vi "Main.vi"() -> ()   [LabVIEW 2023]
doc: "This Continuous Measurement sample project is based on the Queued Message Handler template.\n\nThe Event Handling Loop generates messages based on user interface actions.\n\nThe Message Handling Loop processes messages generated by the Event Handling Loop, or by other messages. There are also Acquisition and Logging message handling loop subVIs, and a chart updating loop."
uses:
  support/Message Queue/Message Cluster.ctl
  Drivers/Resideo Gas Valve/Type Definitions/Temperature Control.ctl
  controls/Product Type.ctl
  controls/UI Data.ctl
  Modbus/Modbus All Data.ctl
  Modbus/Modbus PLC Data All.ctl
  Modbus/Modbus FVIR Control.ctl
  Modbus/Modbus Timing.ctl
  <vilib>/Utility/miscctls.llb/LVDateTimeRec.ctl
  Modbus/Modbus LDO Control.ctl
  WritingDataFile/Data to Save.ctl
  support/Terminate Conditions Cluster.ctl
  Drivers/Inficon Transmitter/Type Definitions/Inficon Data.ctl
  Modbus/Modbus Gas Meter Data.ctl
  Drivers/Alicat LabVIEW Drivers 2v1/Sub-VIs/Data Cluster.ctl
  Drivers/Alicat LabVIEW Drivers 2v1/Sub-VIs/Units of Measure.ctl
  Gas_Rate/HEWH ANSI Rate.ctl
  Drivers/Resideo Gas Valve/Type Definitions/Vesta Info.ctl
  support/Agilent Data.ctl
  support/Event Booleans.ctl
  support/StartStopIntellifaucet.ctl
  support/Mannequin and Gas Position.ctl
  support/Message Queue/Enqueue Message (Single).vi
  <vilib>/Utility/error.llb/Error Cluster From Error Code.vi
  Tenney/support/Message Queue/Enqueue Message (Single).vi
  <vilib>/ErrorRing/Error Ring.xnode
  support/User Event - Stop/User Event - Stop.lvlib
  support/Message Queue/Message Queue.lvlib
  Modbus/Modbus.lvlib
  WritingDataFile/WritingDataFile.lvlib
  SRI8610C - GasChromatograph/SRI8610C-GasChromatograph.lvlib
  Tenney/support/Message Queue/Tenney Message Queue.lvlib
panel:
  out "elements":T1[](array[typedef])
  out "Input Registers":u16[](array[numeric])
  out "States":string[](array[string])
  in  "error in":errorcluster
  out "Version Info":string
  in  "Tab Control":T2(tab)
  out "Actuator spill can is going to Work Pos - FVIR":bool
  out "Actuator spill can is going to Home Pos - FVIR":bool
  out "Actuator mannequin is going to Work Pos - FVIR":bool
  out "Actuator mannequin is going to Home Pos - FVIR":bool
  out "Burner-FVIR":bool caption="Burner - FVIR"
  in  "Move mannequin - Go to Work Pos":bool
  in  "Move mannequin - Go to Home Pos":bool
  in  "Spill can - Go to Work Pos":bool
  in  "Spill can - Go to Home Pos":bool
  in  "Select test case":i32(listbox)
  in  "Stop Test Case FVIR":bool
  in  "Start Test Case FVIR":bool
  out "Start recording data - FVIR":bool
  out "Test chamber is in sequence - FVIR":bool
  out "Can is spilling - FVIR":bool
  out "Mannequin is moving - FVIR":bool
  out "Higher than 0.9% butane":bool
  in  "Water Outlet Valve Close FVIR":bool
  in  "Water Outlet Valve Open FVIR":bool
  in  "Gas Solenoid Valve Close FVIR":bool
  in  "Gas Solenoid Valve Open FVIR":bool
  in  "Water Inlet Valve Close FVIR":bool
  in  "Water Inlet Valve Open FVIR":bool
  out "Water Outlet Flow Proportional - FVIR":bool
  out "Intellifaucet Start - FVIR":bool
  out "Gas Solenoid Valve - FVIR":bool
  out "Water Inlet Valve - FVIR":bool
  out "Water Outlet Valve - FVIR":bool
  in  "Start - SRI Log":bool
  in  "Stop- SRI Log":bool
  in  "Gas Meter Tare Total FVIR":bool
  in  "Gas Meter Tare Rate FVIR":bool
  in  "Reset Flow Meter FVIR":bool caption="Reset Flow Meter"
  in  "Proportioning Valve - FVIR":dbl caption="Proportioning Valve" max=100.0
  in  "Valve % Open - FVIR":dbl=100.0 caption="Valve % Open" min=15.0 max=100.0
  in  "Temp (°F)-FVIR":dbl=70.0 caption="Temperature (°F)" min=32.0 max=203.0
  in  "Start Intellifaucet DRK375 - FVIR":bool
  in  "Stop Intellifaucet DRK375 - FVIR":bool
  out "FVIR Status":string
  in  "Burner OFF FVIR":bool
  in  "Burner ON FVIR":bool
  in  "Test Type - Rate FVIR":string(combo)="Rate"
  out "FVIR Rate Info":string[][](array[string])
  out "FVIR Data":string[][](array[string])
  out "ANSI Display FVIR":string caption="ANSI Display 1"
  in  "Start ANSI FVIR":bool caption="Start ANSI"
  out "Status for error - FVIR":string caption="Error status for FVIR"
  out "Error - FVIR":bool caption="Error"
  in  "Water Heater Temperature (°F) FVIR":bool
  in  "Water Heater Temp (°F) FVIR 2":T3={"Water Heater Temp (°F)"=120, "Differential  (°F)"=10.0} {"Water Heater Temp (°F)" min=32 max=203}
  in  "EnviraCom (On/Off)":bool
  in  "SET Temperature (°F)-EnviraCom":bool
  in  "Short Draw Flow Rate (GPM)":dbl=0.92 format="%#_13g"
  in  "Reset Flow Meter":bool
  in  "Blower OFF":bool
  in  "Blower ON":bool
  in  "Conveyor OFF":bool
  in  "Conveyor ON":bool
  out "Blower":bool
  out "Conveyor":bool
  out "Rotary Actuator (ON/OFF)":bool
  out "Oil spray 1.33cc/min":bool
  out "Oil spray 1.1cc/min":bool
  out "Oil spray 0.8cc/min":bool
  out "Burner-LDO":bool caption="Burner"
  in  "Gas Meter Tare Total":bool
  in  "Gas Meter Tare Rate":bool
  out "LDO Data":string[][](array[string])
  in  "Proportioning Valve - LDO":dbl caption="Proportioning Valve" max=100.0
  in  "Valve % Open - LDO":dbl=50.0 caption="Valve % Open" min=15.0 max=100.0
  in  "Temp (°F)-LDO":dbl=70.0 caption="Temperature (°F)" min=32.0 max=203.0
  in  "Start Intellifaucet DRK375 - LDO":bool
  in  "Stop Intellifaucet DRK375 - LDO":bool
  out "Start recording data - LDO":bool
  out "Test chamber is in sequence":bool
  out "LDO Auto Stop Condition Met?":bool
  in  "Stop Test Case LDO":bool
  in  "Start Test Case LDO":bool
  in  "Water Outlet Valve Close LDO":bool
  in  "Water Outlet Valve Open LDO":bool
  in  "Water Inlet Valve Close LDO":bool
  in  "Water Inlet Valve Open LDO":bool
  in  "Gas Solenoid Valve Close LDO":bool
  in  "Gas Solenoid Valve Open LDO":bool
  in  "Oil Spray 0.8 cc/min Close":bool
  in  "Oil Spray 0.8 cc/min Open":bool
  in  "Oil Spray 1.1 cc/min Close":bool
  in  "Oil Spray 1.1 cc/min Open":bool
  in  "Oil Spray 1.33 cc/min Close":bool
  in  "Oil Spray 1.33 cc/min Open":bool
  in  "Rotary Actuator OFF":bool
  in  "Rotary Actuator ON":bool
  out "Water Outlet Flow Proportional":bool
  out "Intellifaucet Start_LDO":bool
  out "Gas Solenoid Valve":bool
  out "Water Inlet Valve":bool
  out "Water Outlet Valve":bool
  out "LDO Status":string
  in  "Test Type - Rate":string(combo)="Rate"
  out "LDO Rate Info":string[][](array[string])
  out "ANSI Display LDO":string caption="ANSI Display 1"
  in  "Start ANSI LDO":bool caption="Start ANSI"
  in  "Long Draw Flow Rate (GPM)":dbl=0.92 format="%#_13g"
  in  "LDO-Manual Flow Control?":bool=TRUE
  in  "Reset BINs":bool
  in  "Temperature Parameters":T3={"Water Heater Temp (°F)"=135, "Differential  (°F)"=10.0} {"Water Heater Temp (°F)" min=32 max=203}
  in  "Water Heater Temperature (°F)":bool
  in  "Product Type":T4
  out "XY Graph - LDO":T5(graph)
  out "XY Graph - FVIR":T5(graph)
  in  "Y-Axis2 - FVIR":string(combo)
  in  "Y-Axis1 - FVIR":string(combo)
  in  "X-Axis - FVIR":string(combo)
  in  "Y-Axis2 - LDO":string(combo)
  in  "Y-Axis1 - LDO":string(combo)
  in  "X-Axis - LDO":string(combo)
  in  "HHV-NG-Manual":sgl=1069.0
  in  "Manual Heating Value":bool
  out "Error - LDO":bool caption="Error"
  out "Status for error - LDO":string caption="Error status for LDO"
  in  "EnviraCom LDO COM":refnum<visa-resource-name>="EnviraCom_LDO"
  in  "FVIR Save Rate (Default ms)":i32=500
  in  "stop FVIR test":bool
  in  "Pilot Rate (BTU/hr)-FVIR":dbl=800.0
  out "FVIR - Filepath":path
  out "LDO - Filepath":path
  in  "Vesta ON Temperature FVIR":T3={"Water Heater Temp (°F)"=120, "Differential  (°F)"=10.0} {"Water Heater Temp (°F)" min=32 max=203}
  in  "Vesta OFF Temperature FVIR":T3={"Water Heater Temp (°F)"=55, "Differential  (°F)"=10.0} {"Water Heater Temp (°F)" min=32 max=203}
  in  "Vesta ON Temperature LDO":T3={"Water Heater Temp (°F)"=135, "Differential  (°F)"=10.0} {"Water Heater Temp (°F)" min=32 max=203}
  in  "Vesta OFF Temperature LDO":T3={"Water Heater Temp (°F)"=55, "Differential  (°F)"=10.0} {"Water Heater Temp (°F)" min=32 max=203}
  in  "Agilent 34972A":refnum<visa-resource-name>="34972A"
  in  "stop ldo test":bool
  in  "Debug":bool
  out "Message Loop":string[](array[string])
  in  "Time Pause Between Next Mannequin Sequence":u16=60
  in  "Number of Mannequin Movement":u16=3
  in  "Time Delay of Change direction of Mannequin Actuators (mS)":u16=1000
  in  "Full Mannequin Sequence":bool
  in  "FVIR-Flow Rate (GPM)":dbl=3.0 format="%#_13g"
  in  "Temp (°F) - Automatic Mode (FVIR)":dbl=73.0 min=32.0 max=203.0
  in  "Valve % Open - Automatic Mode (FVIR)":dbl=100.0 min=15.0 max=100.0
  in  "Send parameters to PLC FVIR":bool
  in  "Ultramat 23_FVIR":refnum<visa-resource-name>="ULTRAMAT_FVIR"
  in  "VESTA FVIR COM":refnum<visa-resource-name>="VESTA_FVIR"
  in  "FVIR Alicat VISA":refnum<visa-resource-name>="ALICAT_40SLPM_FVIR"
  in  "Ultramat 23_LDO":refnum<visa-resource-name>="ULTRAMAT_LDO"
  in  "LDO Alicat VISA":refnum<visa-resource-name>="ALICAT_40SLPM_LDO"
  in  "VESTA LDO COM":refnum<visa-resource-name>="VESTA_LDO"
  in  "Reset LDO Timers":bool
  in  "Start Auto GPM Gallons-LDO":dbl=5.0 format="%#_13g"
  in  "Clear Unist Alarm":bool
  in  "Temp (°F) - Automatic Mode (LDO)":dbl=70.0 min=32.0 max=203.0
  in  "Valve % Open - Automatic Mode (LDO)":dbl=50.0 min=15.0 max=100.0
  in  "Precondition Purge Gallons":u16=200 caption="Precondition Purge Time (Sec)"
  in  "Pilot Rate (BTU/hr)-LDO":dbl=800.0
  out "FVIR PLC lifebit":bool
  out "Labview lifebit":bool
  in  "Send parameters to PLC LDO":bool
  in  "Burner cycle 1 to 10 - Duty cycle ON (default 55 min.)":u16=55 caption="Burner cycle 1 to 10 - Duty cycle ON"
  in  "Burner cycle 1 to 10 - Duty cycle OFF (default 5 min.)":u16=5 caption="Burner cycle 1 to 10 - Duty cycle OFF"
  in  "Burner cycle 11 to 12 - Duty cycle ON (default 235 min.)":u16=235 caption="Burner cycle 11 to 12 - Duty cycle ON"
  in  "Burner cycle 11 to 12 - Duty cycle OFF (default 5 min.)":u16=5 caption="Burner cycle 11 to 12 - Duty cycle OFF"
  in  "Burner cycle 13 to end - Duty cycle ON (default 55 min.)":u16=55 caption="Burner cycle 13 to end - Duty cycle ON"
  in  "Burner cycle 13 to end - Duty cycle OFF (default 5 min.)":u16=5 caption="Burner cycle 13 to end - Duty cycle OFF"
  in  "Oil 1st sequence ON (default 5 min.)":u16=5 caption="Oil 1st sequence ON"
  in  "Oil 1st sequence OFF (default 5 min.)":u16=25 caption="Oil 1st sequence OFF"
  in  "All subsequent sequence ON (default 3 min.)":u16=3 caption="All subsequent sequence ON"
  in  "All subsequent sequence OFF (default 27 min.)":u16=27 caption="All subsequent sequence OFF"
  in  "Oil spray preconditioning period ON (default 10 min.)":u16=10 caption="Oil spray preconditioning period ON"
  in  "Oil spray preconditioning period OFF  (default 20 min.)":u16=20 caption="Oil spray preconditioning period OFF"
  in  "PLC IP address":string="10.2.0.11"
  in  "Inficon IP Address":string="192.168.1.32"
  in  "Save Rate (ms)":i32=10000
  in  "PLC Loop Rate Standard":u32=1000
  out "EnviraCom is working":bool
  out "Retry Count":dbl
  out "EnviraCom LDO Loop Count":i32
  out "EnviraCom LDO State":string
  out "Vesta is working":bool
  out "Retry Count":dbl
  out "Vesta LDO Loop Count":i32
  out "Vesta LDO State":string
  out "Modbus Loop Rate":i32
  # "Manual mode"
  # "Automatic mode"
  # "Water Outlet Valve"
  # "Gas Solenoid Valve"
  # "Water Inlet Valve"
  # "Status of valves"
  # "Status of actuators"
  # "Status of chamber"
  # "Intellifaucet Control"
  # "Gas Meter"
  # "Water Flow Meter"
  # "Burner ON/OFF"
  # "Manual mode"
  # "Status of devices"
  # "Status of chamber"
  # "Status of valves"
  # "Intellifaucet Control"
  # "This button resets all saved temperature limits. \nKnob must be on Pilot."
  # "Water Flow Meter"
  # "Blower Control"
  # "Conveyor Control"
  # "Gas Meter"
  # "Automatic mode"
  # "Start and stop LDO test"
  # "Water Outlet Valve"
  # "Water Inlet Valve"
  # "Gas Solenoid Valve"
  # "Oil spray at 0.8 cc/min"
  # "Oil spray at 1.1 cc/min"
  # "Oil spray at 1.33 cc/min"
  # "Rotary Actuator\n(Burner ON/OFF)"
  # "LDO Parameters -"
  # "Changing parameters to PLC"
  # "FVIR Changing parameters to PLC"
  # "EnviraCom Communication"
  # "Vesta Communication"
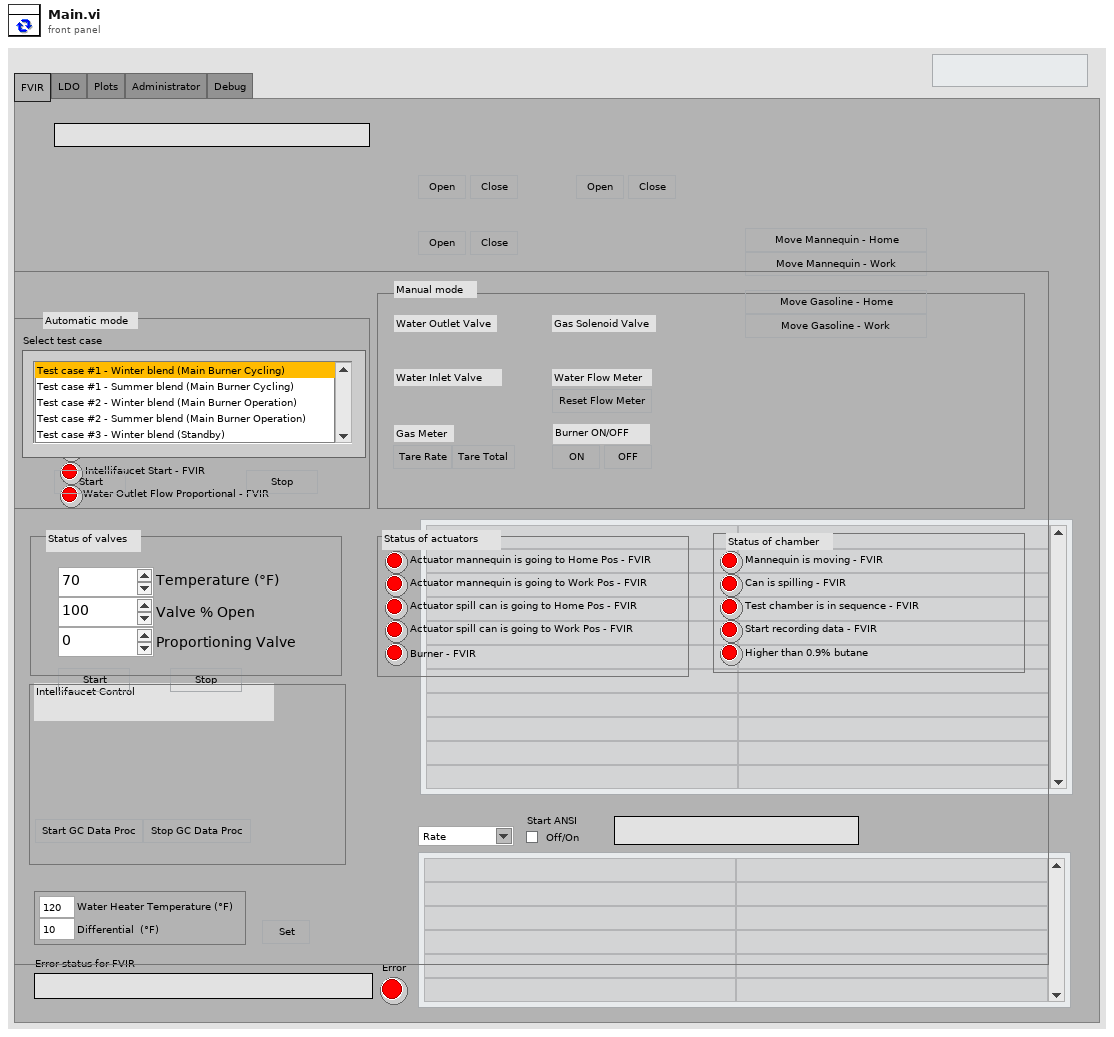
[diagram p1: front panel]
types:
  T1 = typedef "Message Queue.lvlib/Message Cluster.ctl" = cluster{"Message":string, "Message Data":variant}
  T2 = enum32{"FVIR", "LDO", "Plots", "Administrator", "Debug"}
  T3 = typedef "Temperature Control.ctl" = cluster{"Water Heater Temp (°F)":u16, "Differential  (°F)":dbl}
  T4 = typedef "Product Type.ctl" = enum16{"", "Standard ATM", "Power Vent"}
  T5 = cluster{"Time Array Output":dbl[], "Data Array Output":dbl[]}[]
  T6 = typedef "Event Booleans.ctl" = cluster{"Burner ON - LDO":bool, "0.8 ml Bool":bool, "1.1 Bool":bool, "1.33 Bool":bool, "Start recording data-LDO":bool, "Rotary Actuator (ON/OFF)":bool, "Burner ON - FVIR":bool, "Start recording data -FVIR ":bool}
  T7 = typedef "Modbus All Data.ctl" = cluster{"PLC Data":T8, "Inficon Data - ALL":T15, "Gas Data":cluster{"Gas Data - LDO":T16, "Gas Data - FVIR":T16}, "Ultramat 23":cluster{"Ultramat 23 - LDO":string[][], "Ultramat 23 - FVIR":string[][]}, "ANSI Rates":cluster{"ANSI Rate LDO":T19, "ANSI Rate FVIR":T19}, "Vesta Data":cluster{"Vesta LDO":T20, "Vesta FVIR":T20}, "Agilent Data":T21}
  T8 = typedef "Modbus PLC Data All.ctl" = cluster{"PLC Data - FVIR":T9, "PLC Data - LDO":T12, "PLC Registers - ALL":i16[], "Data to Save - ALL":T13, "Terminate Conditions - LDO":T14, "Terminate Conditions - FVIR":cluster{"SRI Butane Values":string[][], "Stop FVIR Test":bool}}
  T9 = typedef "Modbus FVIR Control.ctl" = cluster{"Reset FVIR Totalizer (Status)":bool, "Spare 14":bool, "Actuator mannequin is going to Work Pos - FVIR":bool, "Actuator mannequin is going to Home Pos - FVIR":bool, "Test chamber is in sequence - FVIR ":bool, "Water flow DRK375 is open - FVIR":bool, "Gas Solenoid Valve - FVIR":bool, "Water Inlet Valve - FVIR":bool, "Water Outlet Flow Proportional - FVIR":bool, "Start recording data - FVIR":bool, "Actuator spill can is going to Work Pos - FVIR":bool, "Actuator spill can is going to Home Pos - FVIR":bool, "Water Outlet Valve - FVIR":bool, "Can is spilling - FVIR":bool, "Mannequin is moving - FVIR":bool, "FVIR PLC lifebit":bool, "Status for Error - FVIR":string, "Error-FVIR":bool, "Sensor Data -FVIR":string[][], "Totalized Flow (Gallons)":dbl, "Timing":T10}
  T10 = typedef "Modbus Timing.ctl" = cluster{"First Call Time Ref":dbl, "Precondition Time Ref":dbl, "Test Time Ref":dbl, "Get First Call Time":bool, "Get Precondition Time":bool, "Get Test Time":bool, "Display Time":dbl, "Real-Time Clock":T11, "Absolute Time":dbl}
  T11 = typedef "LVDateTimeRec.ctl" = cluster{"fractional second":dbl, "second":i32, "minute":i32, "hour":i32, "day of month":i32, "month":i32, "year":i32, "day of week":i32, "day of year":i32, "DST":i32}
  T12 = typedef "Modbus LDO Control.ctl" = cluster{"LDO PLC Life Bit":bool, "Start recording data - LDO":bool, "Spare 1":bool, "Water Outlet Valve - LDO":bool, "Water Inlet Valve - LDO":bool, "Gas Solenoid Valve - LDO":bool, "Water flow DRK375 is open - LDO":bool, "Test chamber is in sequence - LDO":bool, "Oil spray 0.8cc/min - LDO":bool, "Oil spray 1.1cc/min - LDO":bool, "Oil spray 1.33cc/min - LDO":bool, "Rotary Actuator (ON/OFF) - LDO":bool, "Water Outlet Flow Proportional - LDO":bool, "Conveyor ON/OFF":bool, "Blower ON/OFF":bool, "Reset LDO Totalizer (Status)":bool, "Status for error - LDO":string, "Error - LDO":bool, "Sensor Data - LDO":string[][], "Thermal Efficiency Rate (GPM)":dbl, "Thermal Efficiency":dbl, "Totalized Flow (Gallons)":dbl, "Counter of oil injections 1.33 cc/min":u16, "Total Cycle Counter":u16, "Counter of oil injections 1.1 cc/min":u16, "Counter of oil injections 0.8 cc/min":u16, "Timing":T10}
  T13 = typedef "Data to Save.ctl" = cluster{"LDO Full Data":string[][], "FVIR Full Data":string[][], "Test Case - FVIR":string, "Test Case - LDO":string}
  T14 = typedef "Terminate Conditions Cluster.ctl" = cluster{"Condition B - Array":dbl[][], "Current Cycle":u16, "Condition C - Array":dbl[][], "Condition A - Array":dbl[][], "400 PPM Disable Counter":bool, "Condition A - Norm":dbl[][], "Condition B - Norm":dbl[][], "Condition C - Norm":dbl[][], "Condition A":bool, "Condition B":bool, "Condition C":bool, "Condition A - Cont Cycle":dbl[][], "Stop Test":bool}
  T15 = typedef "Inficon Data.ctl" = cluster{"Gross Heating Value, Vol (Real, Dry)":dbl, "Nitrogen Component Normalized Mole % (Dry)":dbl, "Methane Component Normalized Mole % (Dry)":dbl, "Carbon Dioxide Component Normalized Mole % (Dry)":dbl, "Ethane Component Normalized Mole % (Dry)":dbl, "Propane Component Normalized Mole % (Dry)":dbl, "i-Pentane Component Normalized Mole % (Dry)":dbl, "i-Butane Component Normalized Mole % (Dry)":dbl, "n-Butane Component Normalized Mole % (Dry)":dbl, "n-Pentane Component Normalized Mole % (Dry)":dbl, "Hexane Component Normalized Mole % (Dry)":dbl, "Heptane Component Normalized Mole % (Dry)":dbl, "Gross Wobbe Index, Real(Dry)":dbl, "Relative Density, Real(Dry)":dbl, "Propylene Component Normalized Mole % (Dry)":dbl, "C4 Olefins Component Normalized Mole % (Dry)":dbl, "Water Component Normalized Mole % (Dry)":dbl}
  T16 = typedef "Modbus Gas Meter Data.ctl" = cluster{"Data Cluster":T17, "Units of Measure Input":T18, "Header Array":string[]}
  T17 = typedef "Data Cluster.ctl" = cluster{"Absolute Pressure":dbl, "Gauge/Diff. Pressure":dbl, "Barometric Pressure":dbl, "Temperature":dbl, "Volumetric Flow":dbl, "Mass Flow":dbl, "Setpoint":dbl, "Valve Drive":dbl, "Totalizer":dbl, "[hr]":dbl, "[min]":dbl, "[sec]":dbl, "Totalizer Average Flow":dbl, "Totalizer Peak Flow":dbl, "Gas selected":string}
  T18 = typedef "Units of Measure.ctl" = cluster{"Abs. Pressure":string, "Gauge/Diff. Press.":string, "Barometric Press.":string, "Temperature":string, "Volume":string, "Mass":string, "Setpoint":string, "Valve Drive":string, "Totalizer":string, "Tot. Timer":string, "Tot. Avg. Flow":string, "Tot. Peak Flow":string}
  T19 = typedef "HEWH ANSI Rate.ctl" = cluster{"Array 1":dbl[], "Array 3":dbl[], "Array 2":dbl[], "Start ANSI":bool, "ANSI Start Time":dbl, "Restart ANSI":bool, "15 Min ANSI Avg (BTU/hr)":dbl, "20 Min ANSI Avg (BTU/hr)":dbl, "25 Min ANSI Avg (BTU/hr)":dbl, "Absolute Pressure":dbl, "Gas Temperature":dbl, "Volumetric Flow Rate":dbl, "Mass Flow Rate":dbl, "Array 4":dbl[], "Array 5":dbl[], "Gas Rate":dbl, "15 Min Pres Avg (PSIA)":dbl, "20 Min Pres Avg (PSIA)":dbl, "25 Min Pres Avg (PSIA)":dbl, "15 Min Temp Avg (°F) ":dbl, "20 Min Temp Avg (°F)":dbl, "25 Min Temp Avg (°F)":dbl, "15 Min Uncorrected Avg (CFH)":dbl, "20 Min Uncorrected Avg (CFH)":dbl, "25 Min Uncorrected Avg (CFH)":dbl, "15 Min Corrected Avg (SCFH)":dbl, "20 Min Corrected Avg (SCFH)":dbl, "25 Min Corrected Avg (SCFH)":dbl, "15 Min Complete":bool, "20 Min Complete":bool, "25 Min Complete":bool, "Heating Value (BTU/ft³)":dbl, "CO CO2 15 Min":string[][], "CO CO2 20 Min":string[][], "CO CO2 25 Min":string[][], "CO CO2 Real Time":string[][]}
  T20 = typedef "Vesta Info.ctl" = cluster{"Temp_W_Raw_U":u16, "Temp_W_Raw_L":u16, "Temperature Water (F)":dbl, "Temperature Water Compensated (F)":dbl, "Temperature Ambient (F)":dbl, "Setpoint Location (F)":dbl, "Heat Request":string, "Fault Ram":string, "PWM DCDC Value":u16, "Pilot Voltage (mV)":dbl, "Setpoint Actual (F)":dbl, "Differential Actual (F)":dbl, "Setpoint User (F)":dbl, "Differential User (F)":dbl, "Termperature FIltered -TCO (F)":dbl, "Temp_C_Raw_1 - Sensor Voltage":string, "Temp_C_Raw_2 - Sensor Voltage":string, "Chamber Sensor Temperature (F)":dbl, "LDO Base Temperature (F)":dbl, "LDO Timer (sec)":i16, "Disabled (0)":bool, "Warming (1)":bool, "Heating (2)":bool, "Cooling Data Write (3)":bool, "Cooling (4)":bool, "Data Read (5)":bool, "N/A":bool, "Temperature Trip (7)":bool, "Burner":bool}
  T21 = typedef "Agilent Data.ctl" = cluster{"Temperature -1 (F)":dbl, "Thermistor Reading -1 (kOhms)":dbl, "Thermistor Reading -2 (kOhms)":dbl, "Temperature -2 (F)":dbl, "Thermistor Reading -3 (kOhms)":dbl, "Temperature -3 (F)":dbl, "Thermistor Reading -4 (kOhms)":dbl, "Temperature -4 (F)":dbl, "Thermistor Reading -5 (kOhms)":dbl, "Temperature -5 (F)":dbl, "Thermistor Reading -6 (kOhms)":dbl, "Temperature -6 (F)":dbl, "Thermistor Reading -7 (kOhms)":dbl, "Temperature -7 (F)":dbl, "Thermistor Reading -8 (kOhms)":dbl, "Temperature -8 (F)":dbl, "Thermistor Reading -9 (kOhms)":dbl, "Temperature -9 (F)":dbl, "Thermistor Reading -10 (kOhms)":dbl, "Temperature -10 (F)":dbl}
  T22 = typedef "UI Data.ctl" = cluster{"Start Ref":refnum<vi>, "Stop Ref":refnum<vi>, "Exit Ref":refnum<vi>, "Status Ref":refnum<vi>, "Connect Ref":refnum<vi>, "Disconnect Ref":refnum<vi>, "Spill can Home pos Ref":refnum<vi>, "Spill can Work pos Ref":refnum<vi>, "Move Mannequin Home pos Ref":refnum<vi>, "Move Mannequin Work pos Ref":refnum<vi>, "Start test case FVIR Ref":refnum<vi>, "Water Outlet Valve Open FVIR Ref":refnum<vi>, "Water Inlet Valve Open FVIR Ref":refnum<vi>, "Gas Solenoid Valve Open FVIR Ref":refnum<vi>, "Water Flow Open FVIR Ref":refnum<vi>, "Listbox Ref":refnum<vi>, "Stop test case FVIR Ref":refnum<vi>, "Water Outlet Valve Close FVIR Ref":refnum<vi>, "Water Inlet Valve Close FVIR Ref":refnum<vi>, "Gas Solenoid Valve Close FVIR Ref":refnum<vi>, "Water Flow Close FVIR Ref":refnum<vi>, "Send Param to PLC FVIR Ref":refnum<vi>, "Water Flow Prop Open FVIR Ref":refnum<vi>, "Water Flow Prop Close FVIR Ref":refnum<vi>, "Start test case LDO Ref":refnum<vi>, "Stop test case LDO Ref":refnum<vi>, "Water Outlet Valve Open LDO Ref":refnum<vi>, "Water Outlet Valve Close LDO Ref":refnum<vi>, "Water Inlet Valve Open LDO Ref":refnum<vi>, "Water Inlet Valve Close LDO Ref":refnum<vi>, "Gas Solenoid Valve Open LDO Ref":refnum<vi>, "Gas Solenoid Valve Close LDO Ref":refnum<vi>, "Water Flow Open LDO Ref":refnum<vi>, "Water Flow Close LDO Ref":refnum<vi>, "Water Flow Prop Open LDO Ref":refnum<vi>, "Water Flow Prop Close LDO Ref":refnum<vi>, "Oil spray 0.8cc/min Open Ref":refnum<vi>, "Oil spray 0.8cc/min Close Ref":refnum<vi>, "Oil spray 1.1cc/min Open Ref":refnum<vi>, "Oil spray 1.1cc/min Close Ref":refnum<vi>, "Oil spray 1.33cc/min Open Ref":refnum<vi>, "Oil spray 1.33cc/min Close Ref":refnum<vi>, "Heater ON Ref":refnum<vi>, "Heater OFF Ref":refnum<vi>, "Send Param to PLC LDO Ref":refnum<vi>}
  T23 = enum8{"Enabled", "Disabled", "Disabled and Grayed Out"}
  T24 = typedef "FileVersionInformation.ctl" = cluster{"FileVersion":string, "ProductName":string, "InternalName":string, "CompanyName":string, "LegalCopyright":string, "FileDescription":string}
  T25 = typedef "Message Queue.lvlib/All Message Queues.ctl" = cluster{"UI":refnum<queue>, "Modbus":refnum<queue>, "Watchdog":refnum<queue>, "ReadDataFile":refnum<queue>, "DataScanning":refnum<queue>, "WriteDataFile":refnum<queue>, "WatchdogWriteFile":refnum<queue>, "OilMachine":refnum<queue>, "Alicat_GasMeter_LDO":refnum<queue>, "Inficon":refnum<queue>, "Ultramat 23_LDO":refnum<queue>, "Alicat_GasMeter_FVIR":refnum<queue>, "Ultramat 23_FVIR":refnum<queue>, "Vesta LDO":refnum<queue>, "Vesta FVIR":refnum<queue>, "Agilent 34972A":refnum<queue>, "EnviraCom LDO":refnum<queue>}
  T26 = typedef "StartStopIntellifaucet.ctl" = enum16{"Start LDO", "Stop LDO", "Start FVIR", "Stop FVIR"}
  T27 = typedef "Mannequin and Gas Position.ctl" = enum16{"Mannequin Home", "Mannequin Work", "Gas Can Home", "Gas Can Work"}
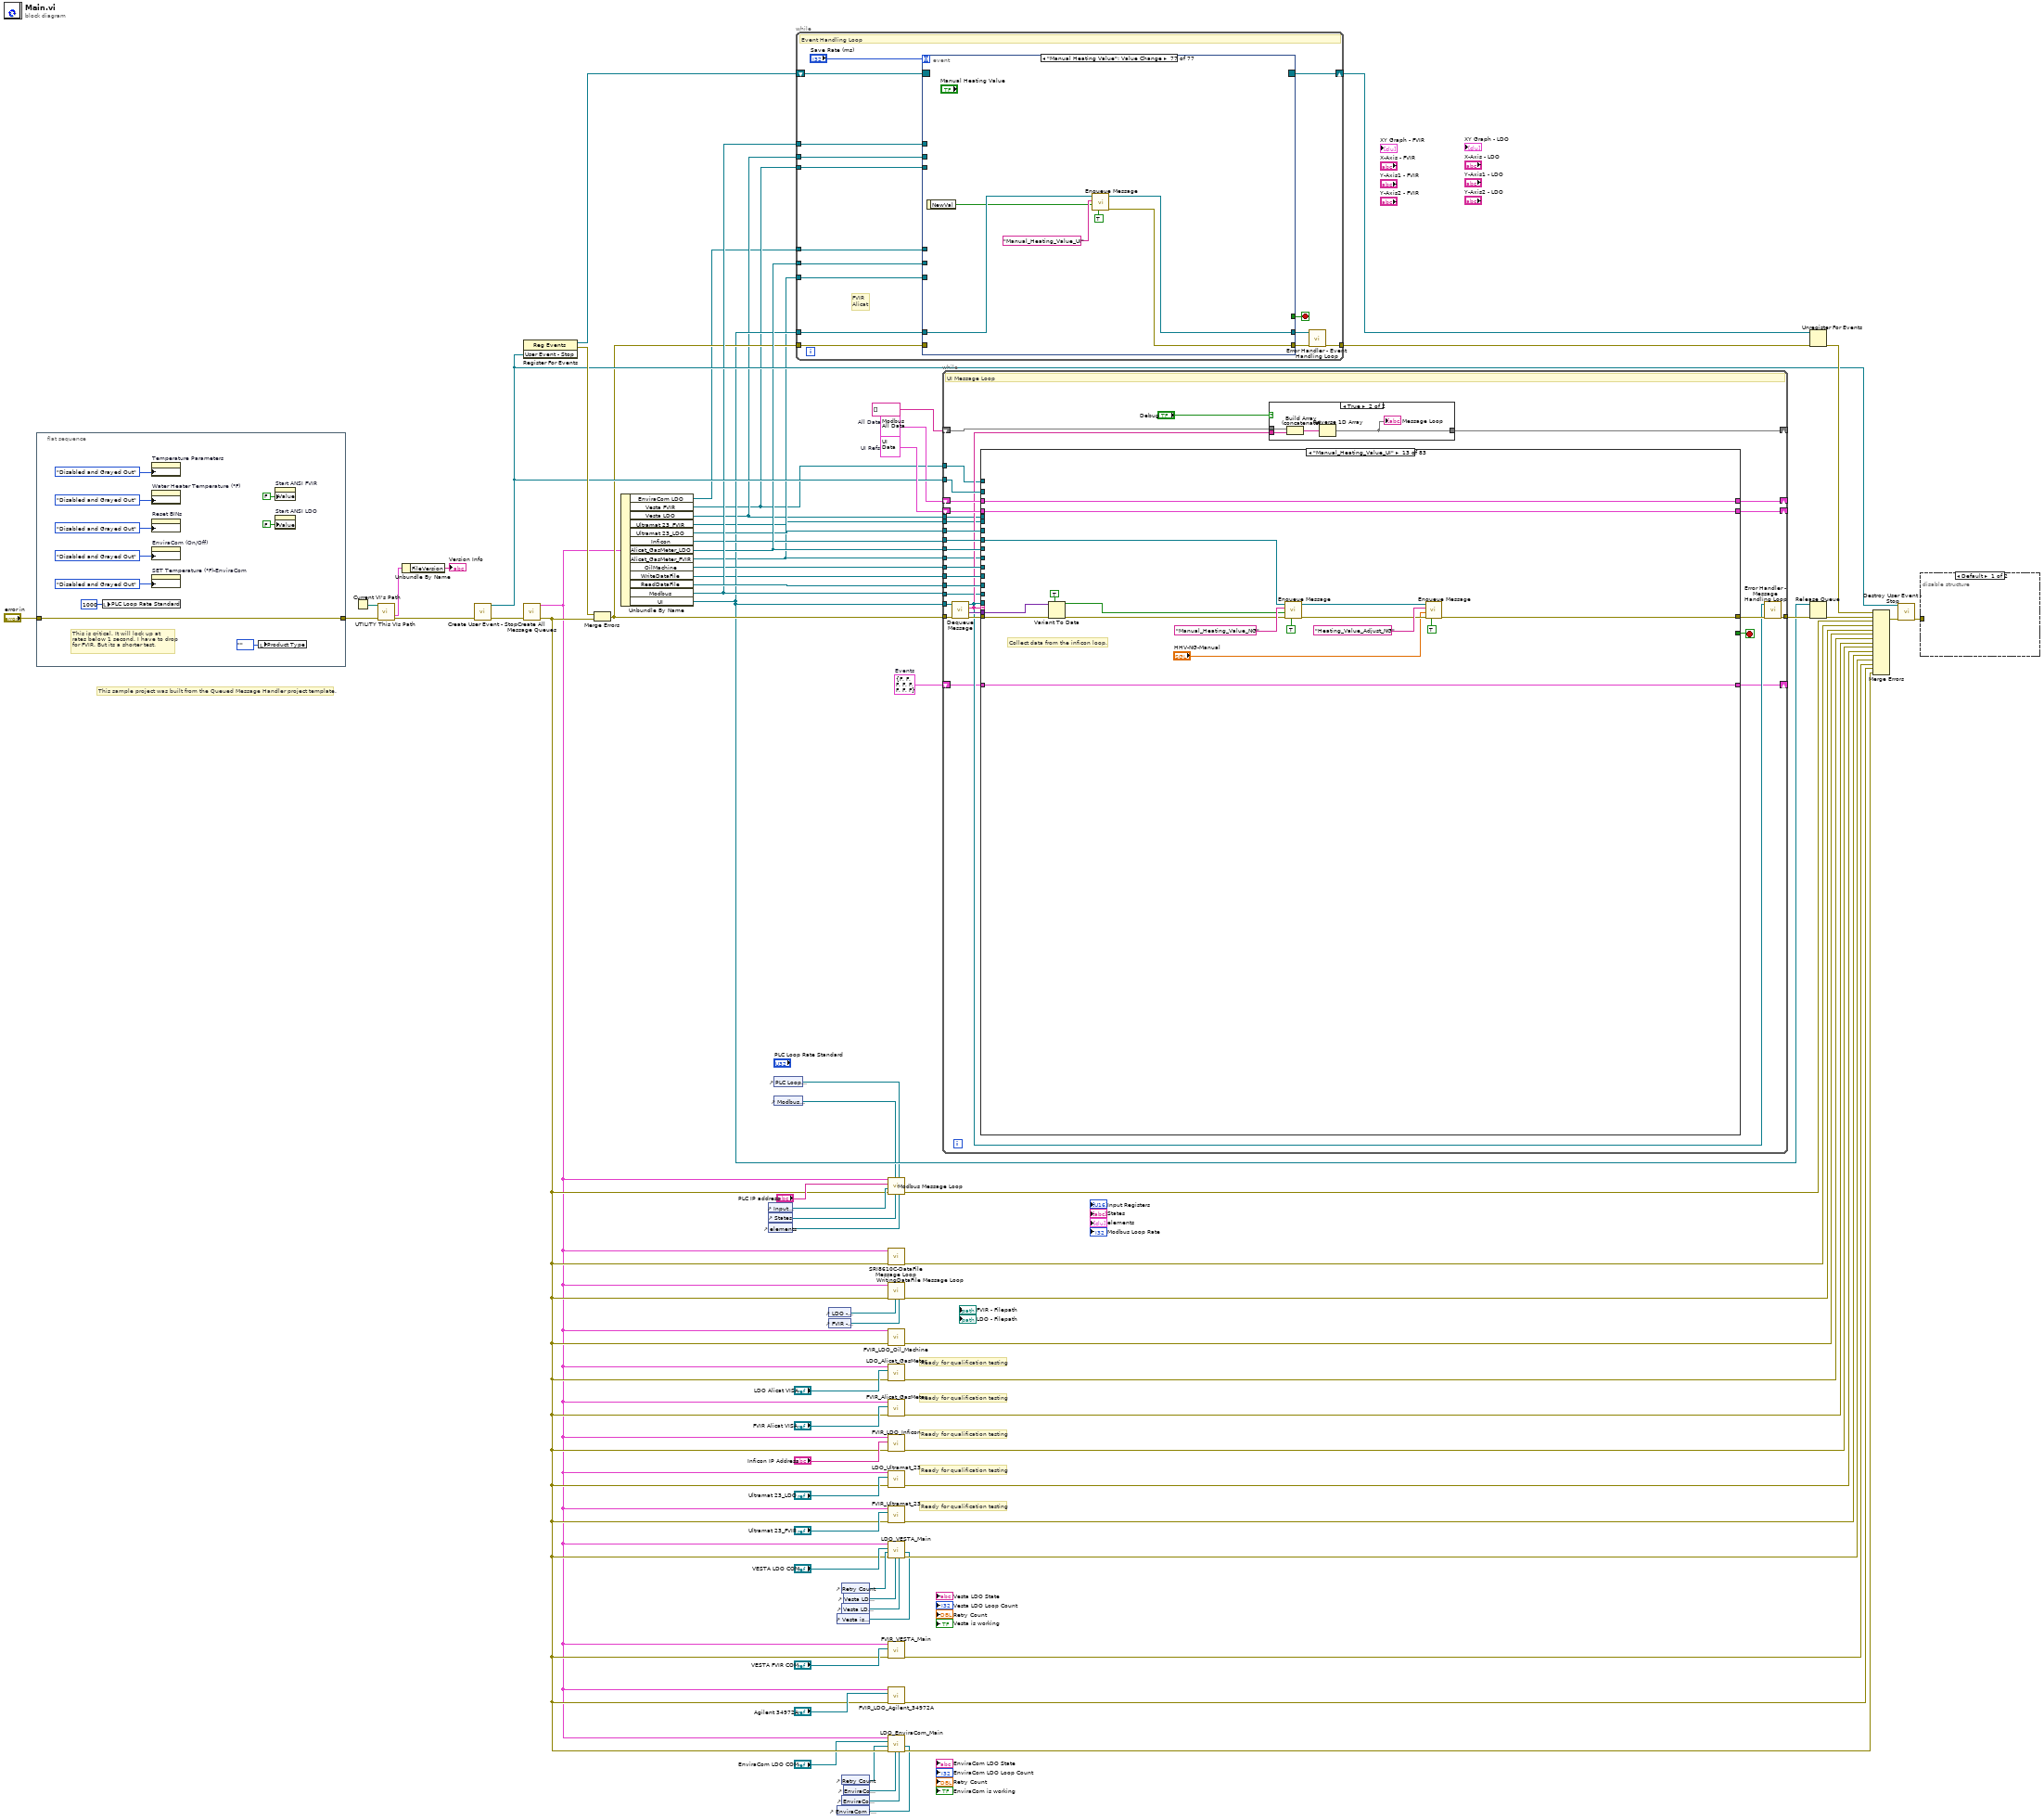
[diagram p0: block diagram]
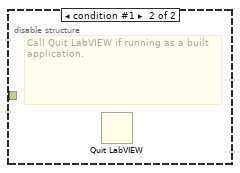
[diagram p2: hidden frame]
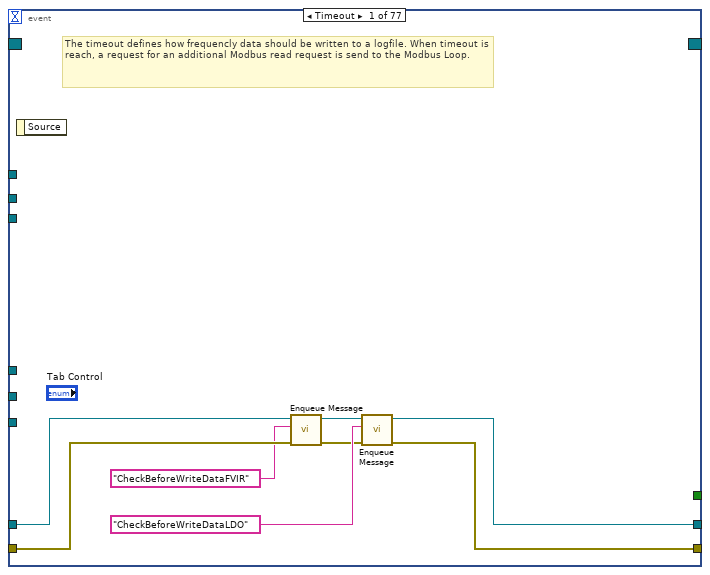
[diagram p3: hidden frame]
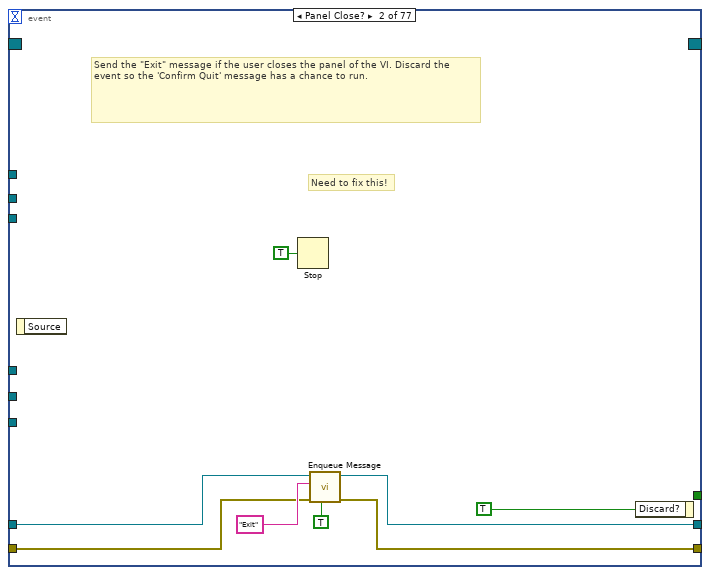
[diagram p4: hidden frame]
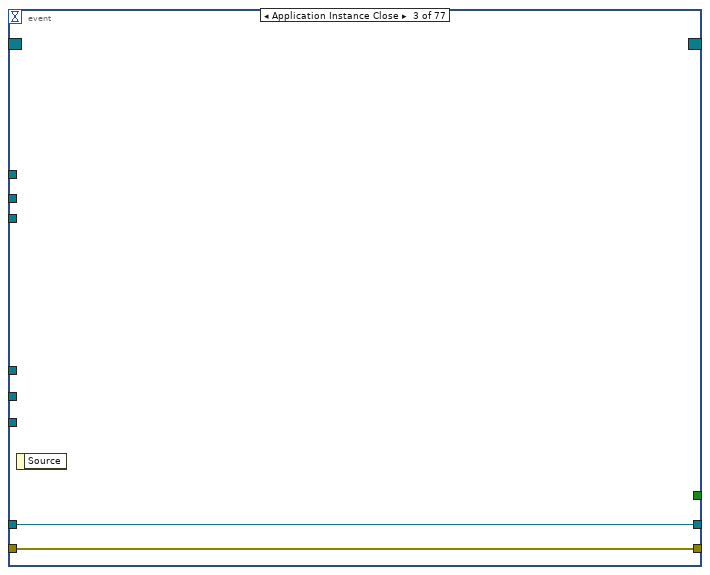
[diagram p5: hidden frame]
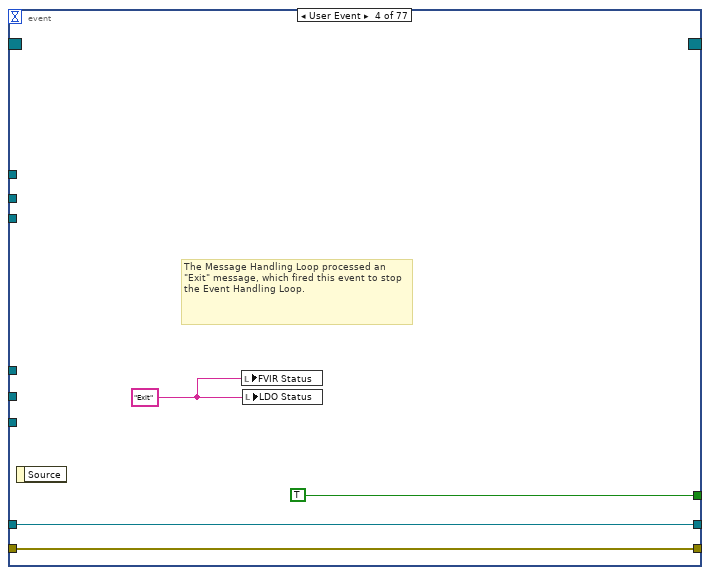
[diagram p6: hidden frame]
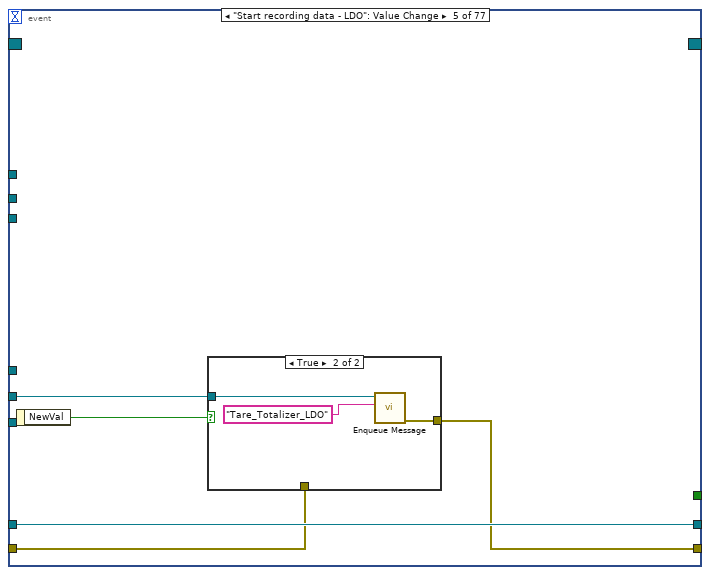
[diagram p7: hidden frame]
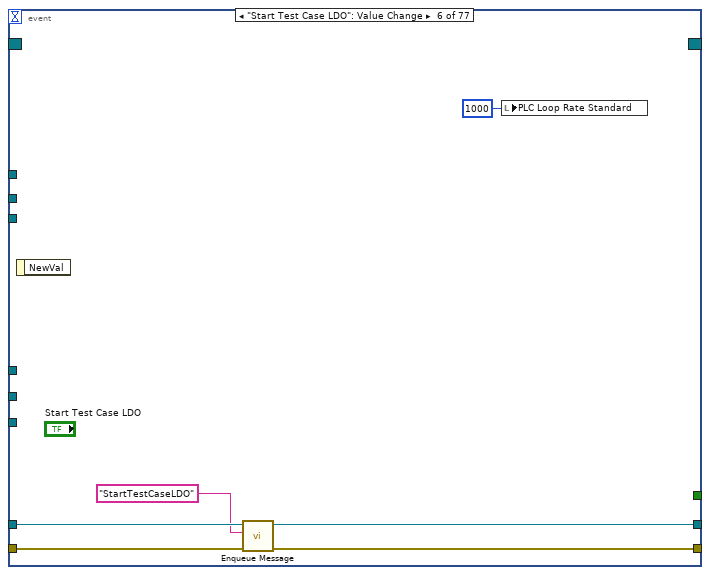
[diagram p9: hidden frame]
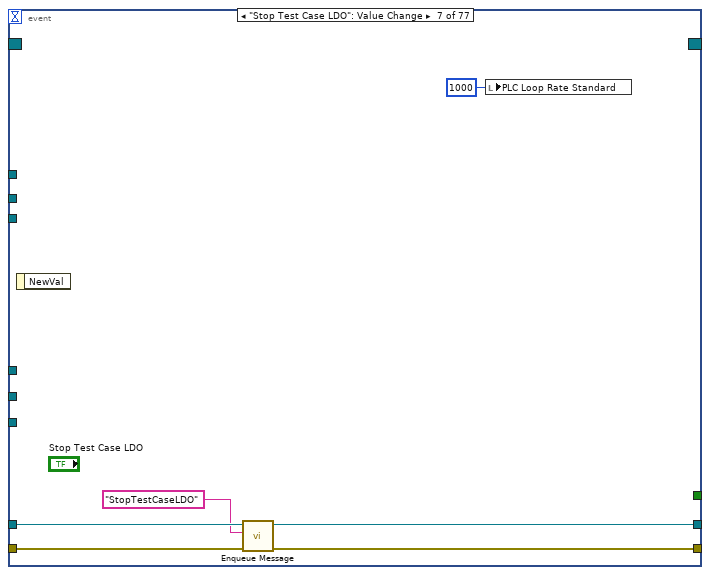
[diagram p10: hidden frame]
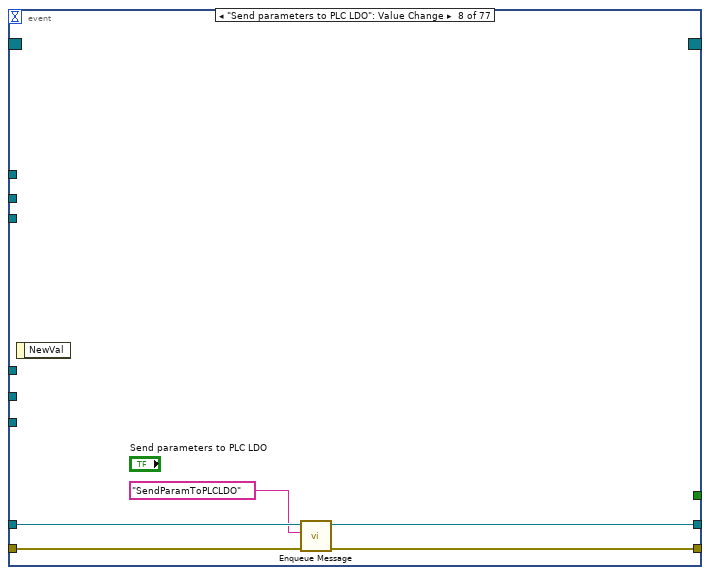
[diagram p11: hidden frame]
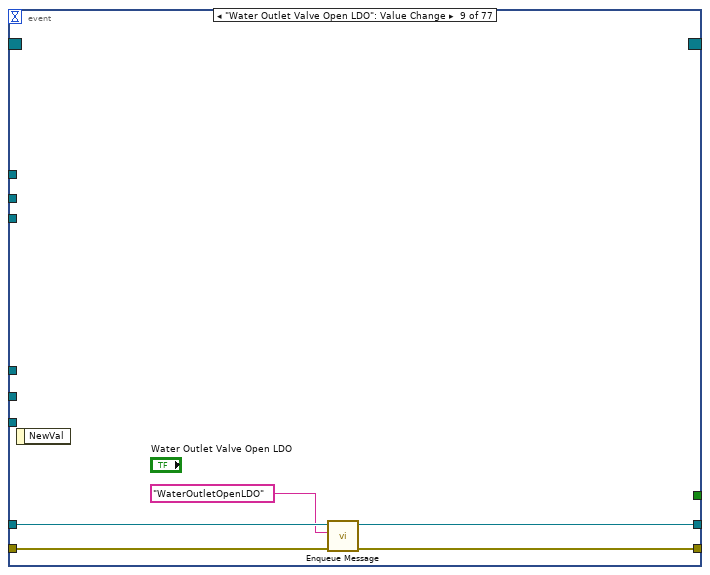
[diagram p12: hidden frame]
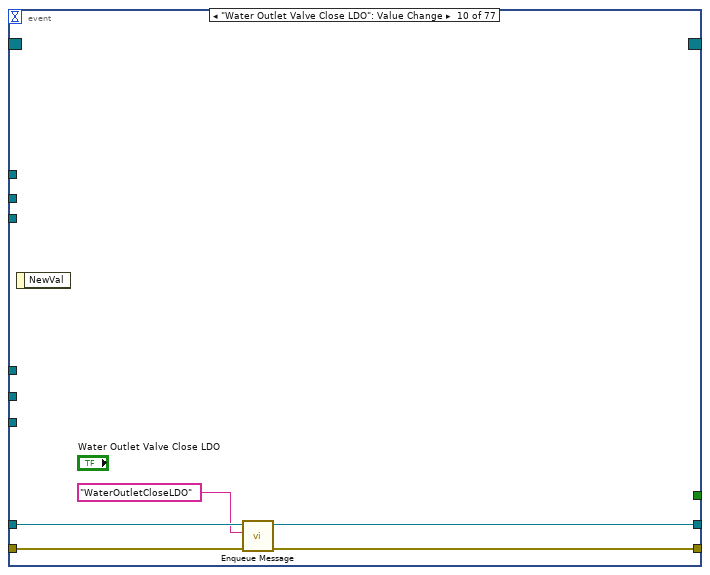
[diagram p13: hidden frame]
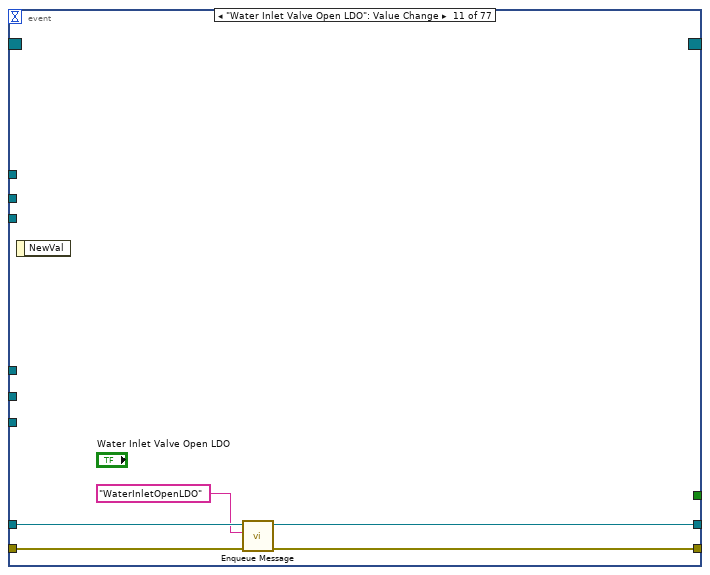
[diagram p14: hidden frame]
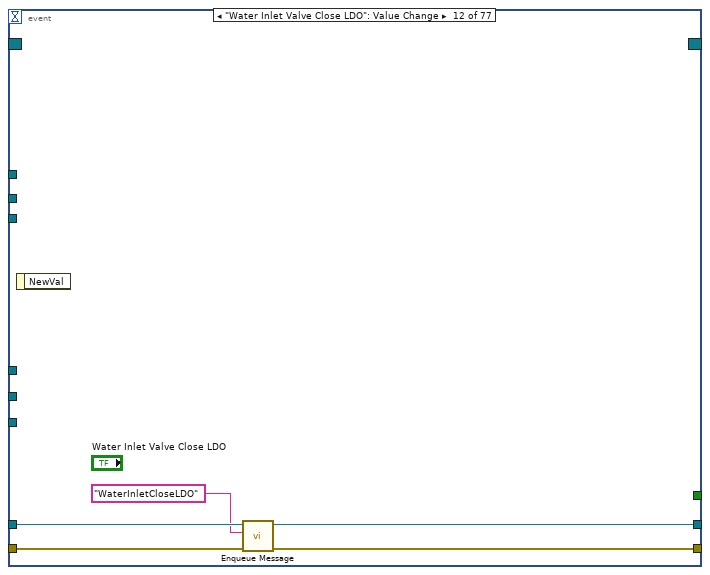
[diagram p15: hidden frame]
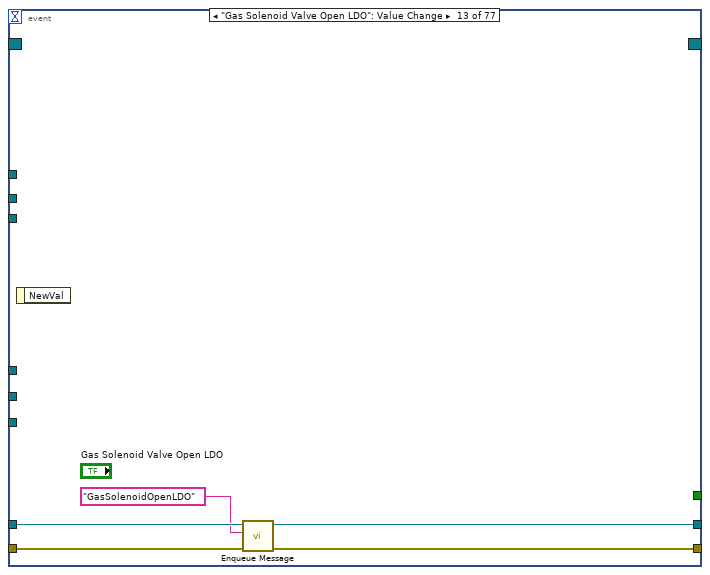
[diagram p16: hidden frame]
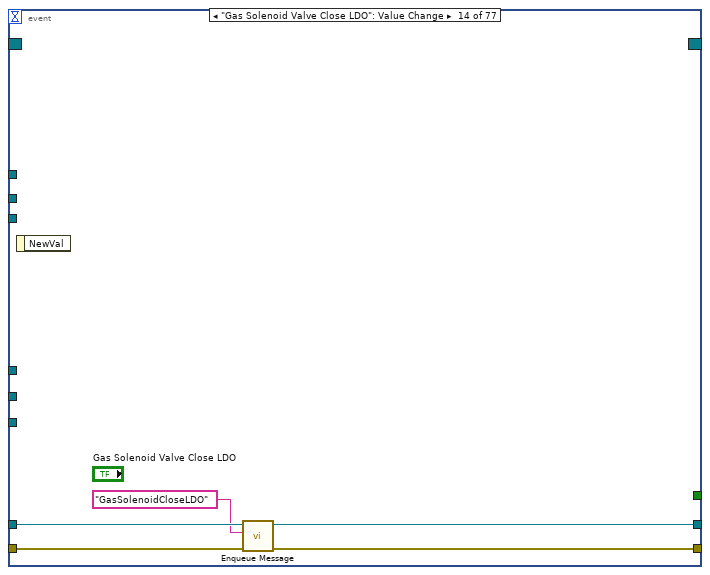
[diagram p17: hidden frame]
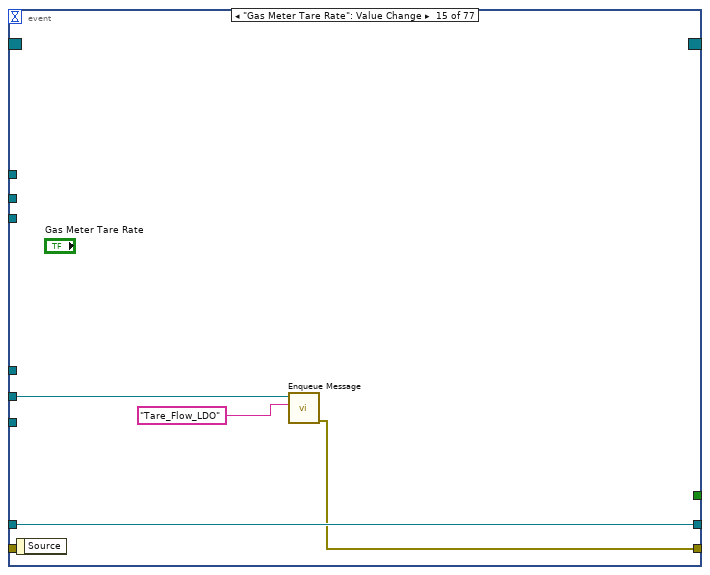
[diagram p18: hidden frame]
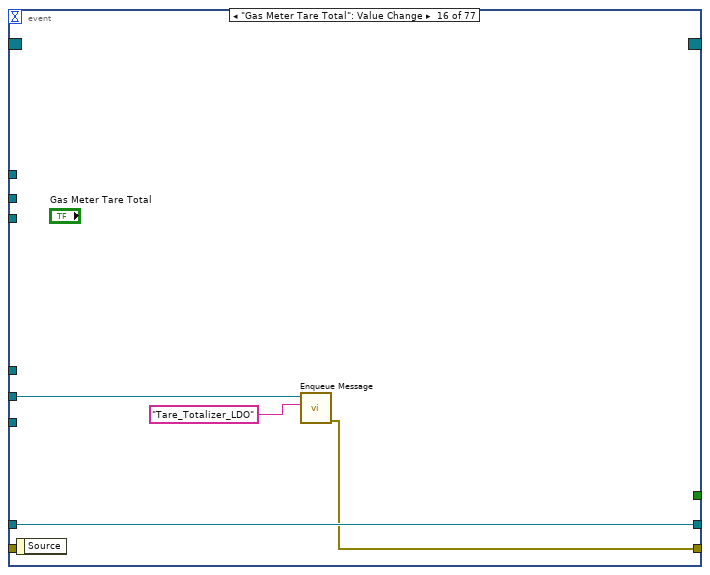
[diagram p19: hidden frame]
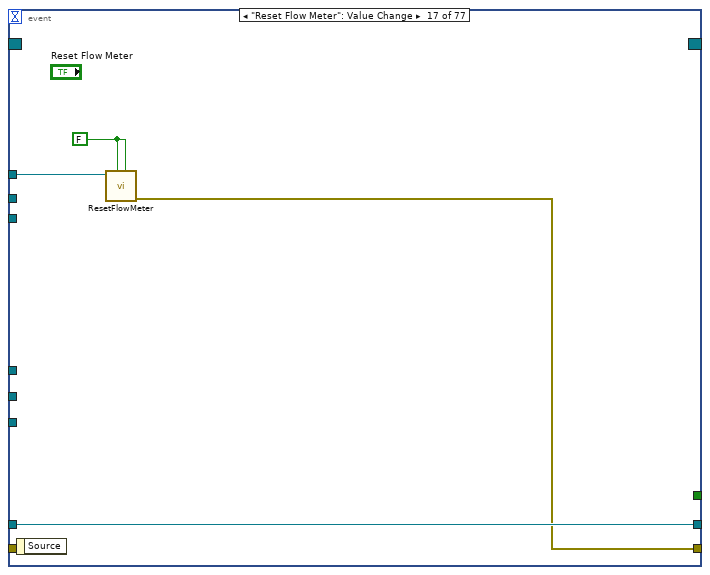
[diagram p20: hidden frame]
diagram:
  w47 = T6 {"Burner ON - LDO"=FALSE, "0.8 ml Bool"=FALSE, "1.1 Bool"=FALSE, "1.33 Bool"=FALSE, "Start recording data-LDO"=FALSE, "Rotary Actuator (ON/OFF)"=FALSE, "Burner ON - FVIR"=FALSE, "Start recording data -FVIR "=FALSE}  # Events
  w56 = T7 {"PLC Data"={"PLC Data - FVIR"={"Reset FVIR Totalizer (Status)"=FALSE, "Spare 14"=FALSE, "Actuator mannequin is going to Work Pos - FVIR"=FALSE, "Actuator mannequin is going to Home Pos - FVIR"=FALSE, "Test chamber is in sequence - FVIR "=FALSE, "Water flow DRK375 is open - FVIR"=FALSE, "Gas Solenoid Valve - FVIR"=FALSE, "Water Inlet Valve - FVIR"=FALSE, "Water Outlet Flow Proportional - FVIR"=FALSE, "Start recording data - FVIR"=FALSE, "Actuator spill can is going to Work Pos - FVIR"=FALSE, "Actuator spill can is going to Home Pos - FVIR"=FALSE, "Water Outlet Valve - FVIR"=FALSE, "Can is spilling - FVIR"=FALSE, "Mannequin is moving - FVIR"=FALSE, "FVIR PLC lifebit"=FALSE, "Status for Error - FVIR"="", "Error-FVIR"=FALSE, "Sensor Data -FVIR"=[], "Totalized Flow (Gallons)"=0.0, "Timing"={"First Call Time Ref"=0.0, "Precondition Time Ref"=0.0, "Test Time Ref"=0.0, "Get First Call Time"=FALSE, "Get Precondition Time"=FALSE, "Get Test Time"=FALSE, "Display Time"=0.0, "Real-Time Clock"={"fractional second"=0.0, "second"=0, "minute"=0, "hour"=0, "day of month"=0, "month"=0, "year"=0, "day of week"=0, "day of year"=0, "DST"=0}, "Absolute Time"=0.0}}, "PLC Data - LDO"={"LDO PLC Life Bit"=FALSE, "Start recording data - LDO"=FALSE, "Spare 1"=FALSE, "Water Outlet Valve - LDO"=FALSE, "Water Inlet Valve - LDO"=FALSE, "Gas Solenoid Valve - LDO"=FALSE, "Water flow DRK375 is open - LDO"=FALSE, "Test chamber is in sequence - LDO"=FALSE, "Oil spray 0.8cc/min - LDO"=FALSE, "Oil spray 1.1cc/min - LDO"=FALSE, "Oil spray 1.33cc/min - LDO"=FALSE, "Rotary Actuator (ON/OFF) - LDO"=FALSE, "Water Outlet Flow Proportional - LDO"=FALSE, "Conveyor ON/OFF"=FALSE, "Blower ON/OFF"=FALSE, "Reset LDO Totalizer (Status)"=FALSE, "Status for error - LDO"="", "Error - LDO"=FALSE, "Sensor Data - LDO"=[], "Thermal Efficiency Rate (GPM)"=0.0, "Thermal Efficiency"=0.0, "Totalized Flow (Gallons)"=0.0, "Counter of oil injections 1.33 cc/min"=0, "Total Cycle Counter"=0, "Counter of oil injections 1.1 cc/min"=0, "Counter of oil injections 0.8 cc/min"=0, "Timing"={"First Call Time Ref"=0.0, "Precondition Time Ref"=0.0, "Test Time Ref"=0.0, "Get First Call Time"=FALSE, "Get Precondition Time"=FALSE, "Get Test Time"=FALSE, "Display Time"=0.0, "Real-Time Clock"={"fractional second"=0.0, "second"=0, "minute"=0, "hour"=0, "day of month"=0, "month"=0, "year"=0, "day of week"=0, "day of year"=0, "DST"=0}, "Absolute Time"=0.0}}, "PLC Registers - ALL"=[], "Data to Save - ALL"={"LDO Full Data"=[], "FVIR Full Data"=[], "Test Case - FVIR"="", "Test Case - LDO"=""}, "Terminate Conditions - LDO"={"Condition B - Array"=[], "Current Cycle"=0, "Condition C - Array"=[], "Condition A - Array"=[], "400 PPM Disable Counter"=FALSE, "Condition A - Norm"=[], "Condition B - Norm"=[], "Condition C - Norm"=[], "Condition A"=FALSE, "Condition B"=FALSE, "Condition C"=FALSE, "Condition A - Cont Cycle"=[], "Stop Test"=FALSE}, "Terminate Conditions - FVIR"={"SRI Butane Values"=[], "Stop FVIR Test"=FALSE}}, "Inficon Data - ALL"={"Gross Heating Value, Vol (Real, Dry)"=0.0, "Nitrogen Component Normalized Mole % (Dry)"=0.0, "Methane Component Normalized Mole % (Dry)"=0.0, "Carbon Dioxide Component Normalized Mole % (Dry)"=0.0, "Ethane Component Normalized Mole % (Dry)"=0.0, "Propane Component Normalized Mole % (Dry)"=0.0, "i-Pentane Component Normalized Mole % (Dry)"=0.0, "i-Butane Component Normalized Mole % (Dry)"=0.0, "n-Butane Component Normalized Mole % (Dry)"=0.0, "n-Pentane Component Normalized Mole % (Dry)"=0.0, "Hexane Component Normalized Mole % (Dry)"=0.0, "Heptane Component Normalized Mole % (Dry)"=0.0, "Gross Wobbe Index, Real(Dry)"=0.0, "Relative Density, Real(Dry)"=0.0, "Propylene Component Normalized Mole % (Dry)"=0.0, "C4 Olefins Component Normalized Mole % (Dry)"=0.0, "Water Component Normalized Mole % (Dry)"=0.0}, "Gas Data"={"Gas Data - LDO"={"Data Cluster"={"Absolute Pressure"=0.0, "Gauge/Diff. Pressure"=0.0, "Barometric Pressure"=0.0, "Temperature"=0.0, "Volumetric Flow"=0.0, "Mass Flow"=0.0, "Setpoint"=0.0, "Valve Drive"=0.0, "Totalizer"=0.0, "[hr]"=0.0, "[min]"=0.0, "[sec]"=0.0, "Totalizer Average Flow"=0.0, "Totalizer Peak Flow"=0.0, "Gas selected"=""}, "Units of Measure Input"={"Abs. Pressure"="", "Gauge/Diff. Press."="", "Barometric Press."="", "Temperature"="", "Volume"="", "Mass"="", "Setpoint"="", "Valve Drive"="", "Totalizer"="", "Tot. Timer"="", "Tot. Avg. Flow"="", "Tot. Peak Flow"=""}, "Header Array"=[]}, "Gas Data - FVIR"={"Data Cluster"={"Absolute Pressure"=0.0, "Gauge/Diff. Pressure"=0.0, "Barometric Pressure"=0.0, "Temperature"=0.0, "Volumetric Flow"=0.0, "Mass Flow"=0.0, "Setpoint"=0.0, "Valve Drive"=0.0, "Totalizer"=0.0, "[hr]"=0.0, "[min]"=0.0, "[sec]"=0.0, "Totalizer Average Flow"=0.0, "Totalizer Peak Flow"=0.0, "Gas selected"=""}, "Units of Measure Input"={"Abs. Pressure"="", "Gauge/Diff. Press."="", "Barometric Press."="", "Temperature"="", "Volume"="", "Mass"="", "Setpoint"="", "Valve Drive"="", "Totalizer"="", "Tot. Timer"="", "Tot. Avg. Flow"="", "Tot. Peak Flow"=""}, "Header Array"=[]}}, "Ultramat 23"={"Ultramat 23 - LDO"=[], "Ultramat 23 - FVIR"=[]}, "ANSI Rates"={"ANSI Rate LDO"={"Array 1"=[], "Array 3"=[], "Array 2"=[], "Start ANSI"=FALSE, "ANSI Start Time"=0.0, "Restart ANSI"=FALSE, "15 Min ANSI Avg (BTU/hr)"=0.0, "20 Min ANSI Avg (BTU/hr)"=0.0, "25 Min ANSI Avg (BTU/hr)"=0.0, "Absolute Pressure"=0.0, "Gas Temperature"=0.0, "Volumetric Flow Rate"=0.0, "Mass Flow Rate"=0.0, "Array 4"=[], "Array 5"=[], "Gas Rate"=0.0, "15 Min Pres Avg (PSIA)"=0.0, "20 Min Pres Avg (PSIA)"=0.0, "25 Min Pres Avg (PSIA)"=0.0, "15 Min Temp Avg (°F) "=0.0, "20 Min Temp Avg (°F)"=0.0, "25 Min Temp Avg (°F)"=0.0, "15 Min Uncorrected Avg (CFH)"=0.0, "20 Min Uncorrected Avg (CFH)"=0.0, "25 Min Uncorrected Avg (CFH)"=0.0, "15 Min Corrected Avg (SCFH)"=0.0, "20 Min Corrected Avg (SCFH)"=0.0, "25 Min Corrected Avg (SCFH)"=0.0, "15 Min Complete"=FALSE, "20 Min Complete"=FALSE, "25 Min Complete"=FALSE, "Heating Value (BTU/ft³)"=0.0, "CO CO2 15 Min"=[], "CO CO2 20 Min"=[], "CO CO2 25 Min"=[], "CO CO2 Real Time"=[]}, "ANSI Rate FVIR"={"Array 1"=[], "Array 3"=[], "Array 2"=[], "Start ANSI"=FALSE, "ANSI Start Time"=0.0, "Restart ANSI"=FALSE, "15 Min ANSI Avg (BTU/hr)"=0.0, "20 Min ANSI Avg (BTU/hr)"=0.0, "25 Min ANSI Avg (BTU/hr)"=0.0, "Absolute Pressure"=0.0, "Gas Temperature"=0.0, "Volumetric Flow Rate"=0.0, "Mass Flow Rate"=0.0, "Array 4"=[], "Array 5"=[], "Gas Rate"=0.0, "15 Min Pres Avg (PSIA)"=0.0, "20 Min Pres Avg (PSIA)"=0.0, "25 Min Pres Avg (PSIA)"=0.0, "15 Min Temp Avg (°F) "=0.0, "20 Min Temp Avg (°F)"=0.0, "25 Min Temp Avg (°F)"=0.0, "15 Min Uncorrected Avg (CFH)"=0.0, "20 Min Uncorrected Avg (CFH)"=0.0, "25 Min Uncorrected Avg (CFH)"=0.0, "15 Min Corrected Avg (SCFH)"=0.0, "20 Min Corrected Avg (SCFH)"=0.0, "25 Min Corrected Avg (SCFH)"=0.0, "15 Min Complete"=FALSE, "20 Min Complete"=FALSE, "25 Min Complete"=FALSE, "Heating Value (BTU/ft³)"=0.0, "CO CO2 15 Min"=[], "CO CO2 20 Min"=[], "CO CO2 25 Min"=[], "CO CO2 Real Time"=[]}}, "Vesta Data"={"Vesta LDO"={"Temp_W_Raw_U"=0, "Temp_W_Raw_L"=0, "Temperature Water (F)"=0.0, "Temperature Water Compensated (F)"=0.0, "Temperature Ambient (F)"=0.0, "Setpoint Location (F)"=0.0, "Heat Request"="", "Fault Ram"="", "PWM DCDC Value"=0, "Pilot Voltage (mV)"=0.0, "Setpoint Actual (F)"=0.0, "Differential Actual (F)"=0.0, "Setpoint User (F)"=0.0, "Differential User (F)"=0.0, "Termperature FIltered -TCO (F)"=0.0, "Temp_C_Raw_1 - Sensor Voltage"="", "Temp_C_Raw_2 - Sensor Voltage"="", "Chamber Sensor Temperature (F)"=0.0, "LDO Base Temperature (F)"=0.0, "LDO Timer (sec)"=0, "Disabled (0)"=FALSE, "Warming (1)"=FALSE, "Heating (2)"=FALSE, "Cooling Data Write (3)"=FALSE, "Cooling (4)"=FALSE, "Data Read (5)"=FALSE, "N/A"=FALSE, "Temperature Trip (7)"=FALSE, "Burner"=FALSE}, "Vesta FVIR"={"Temp_W_Raw_U"=0, "Temp_W_Raw_L"=0, "Temperature Water (F)"=0.0, "Temperature Water Compensated (F)"=0.0, "Temperature Ambient (F)"=0.0, "Setpoint Location (F)"=0.0, "Heat Request"="", "Fault Ram"="", "PWM DCDC Value"=0, "Pilot Voltage (mV)"=0.0, "Setpoint Actual (F)"=0.0, "Differential Actual (F)"=0.0, "Setpoint User (F)"=0.0, "Differential User (F)"=0.0, "Termperature FIltered -TCO (F)"=0.0, "Temp_C_Raw_1 - Sensor Voltage"="", "Temp_C_Raw_2 - Sensor Voltage"="", "Chamber Sensor Temperature (F)"=0.0, "LDO Base Temperature (F)"=0.0, "LDO Timer (sec)"=0, "Disabled (0)"=FALSE, "Warming (1)"=FALSE, "Heating (2)"=FALSE, "Cooling Data Write (3)"=FALSE, "Cooling (4)"=FALSE, "Data Read (5)"=FALSE, "N/A"=FALSE, "Temperature Trip (7)"=FALSE, "Burner"=FALSE}}, "Agilent Data"={"Temperature -1 (F)"=0.0, "Thermistor Reading -1 (kOhms)"=0.0, "Thermistor Reading -2 (kOhms)"=0.0, "Temperature -2 (F)"=0.0, "Thermistor Reading -3 (kOhms)"=0.0, "Temperature -3 (F)"=0.0, "Thermistor Reading -4 (kOhms)"=0.0, "Temperature -4 (F)"=0.0, "Thermistor Reading -5 (kOhms)"=0.0, "Temperature -5 (F)"=0.0, "Thermistor Reading -6 (kOhms)"=0.0, "Temperature -6 (F)"=0.0, "Thermistor Reading -7 (kOhms)"=0.0, "Temperature -7 (F)"=0.0, "Thermistor Reading -8 (kOhms)"=0.0, "Temperature -8 (F)"=0.0, "Thermistor Reading -9 (kOhms)"=0.0, "Temperature -9 (F)"=0.0, "Thermistor Reading -10 (kOhms)"=0.0, "Temperature -10 (F)"=0.0}}  # All Data
  w70 = T22 {"Start Ref"=refnum, "Stop Ref"=refnum, "Exit Ref"=refnum, "Status Ref"=refnum, "Connect Ref"=refnum, "Disconnect Ref"=refnum, "Spill can Home pos Ref"=refnum, "Spill can Work pos Ref"=refnum, "Move Mannequin Home pos Ref"=refnum, "Move Mannequin Work pos Ref"=refnum, "Start test case FVIR Ref"=refnum, "Water Outlet Valve Open FVIR Ref"=refnum, "Water Inlet Valve Open FVIR Ref"=refnum, "Gas Solenoid Valve Open FVIR Ref"=refnum, "Water Flow Open FVIR Ref"=refnum, "Listbox Ref"=refnum, "Stop test case FVIR Ref"=refnum, "Water Outlet Valve Close FVIR Ref"=refnum, "Water Inlet Valve Close FVIR Ref"=refnum, "Gas Solenoid Valve Close FVIR Ref"=refnum, "Water Flow Close FVIR Ref"=refnum, "Send Param to PLC FVIR Ref"=refnum, "Water Flow Prop Open FVIR Ref"=refnum, "Water Flow Prop Close FVIR Ref"=refnum, "Start test case LDO Ref"=refnum, "Stop test case LDO Ref"=refnum, "Water Outlet Valve Open LDO Ref"=refnum, "Water Outlet Valve Close LDO Ref"=refnum, "Water Inlet Valve Open LDO Ref"=refnum, "Water Inlet Valve Close LDO Ref"=refnum, "Gas Solenoid Valve Open LDO Ref"=refnum, "Gas Solenoid Valve Close LDO Ref"=refnum, "Water Flow Open LDO Ref"=refnum, "Water Flow Close LDO Ref"=refnum, "Water Flow Prop Open LDO Ref"=refnum, "Water Flow Prop Close LDO Ref"=refnum, "Oil spray 0.8cc/min Open Ref"=refnum, "Oil spray 0.8cc/min Close Ref"=refnum, "Oil spray 1.1cc/min Open Ref"=refnum, "Oil spray 1.1cc/min Close Ref"=refnum, "Oil spray 1.33cc/min Open Ref"=refnum, "Oil spray 1.33cc/min Close Ref"=refnum, "Heater ON Ref"=refnum, "Heater OFF Ref"=refnum, "Send Param to PLC LDO Ref"=refnum}  # UI Refs
  # "Ready for qualification testing"
  # "Ready for qualification testing"
  # "Ready for qualification testing"
  # "Ready for qualification testing"
  # "Ready for qualification testing"
  # "This sample project was built from the Queued Message Handler project template."
  n1 = flat-sequence {
    tunnel: "error in" -> [w84]
    tunnel: [w84] -> w31
    frame #0 {
      # "This is critical. It will lock up at \nrates below 1 second. I have to drop\nfor FVIR. But its a shorter test."
      n2 = local write "PLC Loop Rate Standard"(u32 1000 ("PLC Loop Rate Standard")) -> ()
      n3 = property on="Temperature Parameters" class="Clust (strict)"("DisabledEnum"=T23."Disabled and Grayed Out" ("Disabled")) -> ()  [unwired: 2 in, 2 out]
      n4 = property on="Water Heater Temperature (°F)" class="Bool"("DisabledEnum"=T23."Disabled and Grayed Out" ("Disabled")) -> ()  [unwired: 2 in, 2 out]
      n5 = property on="Reset BINs" class="Bool"("DisabledEnum"=T23."Disabled and Grayed Out" ("Disabled")) -> ()  [unwired: 2 in, 2 out]
      n6 = property on="EnviraCom (On/Off)" class="Bool (strict)"("DisabledEnum"=T23."Disabled and Grayed Out" ("Disabled")) -> ()  [unwired: 2 in, 2 out]
      n7 = property on="SET Temperature (°F)-EnviraCom" class="Bool"("DisabledEnum"=T23."Disabled and Grayed Out" ("Disabled")) -> ()  [unwired: 2 in, 2 out]
      n8 = local write "Product Type"(Product_Type."" ("Product Type")) -> ()
      n9 = property on="Start ANSI FVIR" class="Bool (strict)"("Value"=FALSE ("Start ANSI FVIR")) -> ()  [unwired: 2 in, 2 out]
      n10 = property on="Start ANSI LDO" class="Bool (strict)"("Value"=FALSE ("Start ANSI LDO")) -> ()  [unwired: 2 in, 2 out]
    }
  }
  n11 = Current VI's Path() -> (path=w41:path)
  n12 = call "UTILITY This VIs Path.vi"("path"=w41, "error in (no error)"=w31) -> ("FileVersionInfo Out"=w40:T24, "error out"=w42:errorcluster)  [unwired: 7 in, 5 out]
  n13 = Unbundle By Name(w40) -> ("FileVersion"=→"Version Info":string)
  n14 = call "Create User Event - Stop.vi"("error in (no error)"=w42) -> ("error out"=w73:errorcluster, "User Event - Stop"=w65:refnum<user-event>)  [unwired: 9 in]
  n15 = register-events(w65) -> (reference out=w67:refnum<event-registration>, error out=w66:errorcluster)  [unwired: 2 in]
  n16 = call "Create All Message Queues.vi"("error in (no error)"=w73) -> ("error out"=w11:errorcluster, "Message Queues out"=w9:T25)  [unwired: 9 in]
  n17 = Merge Errors(w66, w11) -> (w46:errorcluster)
  n18 = Unbundle By Name(w9) -> ("EnviraCom LDO"=w3:refnum<queue>, "Vesta FVIR"=w23:refnum<queue>, "Vesta LDO"=w26:refnum<queue>, "Ultramat 23_FVIR"=w35:refnum<queue>, "Ultramat 23_LDO"=w48:refnum<queue>, "Inficon"=w54:refnum<queue>, "Alicat_GasMeter_LDO"=w55:refnum<queue>, "Alicat_GasMeter_FVIR"=w38:refnum<queue>, "OilMachine"=w58:refnum<queue>, "WriteDataFile"=w34:refnum<queue>, "ReadDataFile"=w64:refnum<queue>, "Modbus"=w63:refnum<queue>, "UI"=w44:refnum<queue>)
  n19 = control-ref of="Input Registers"() -> (w21:refnum<vi>)
  n20 = control-ref of="States"() -> (w22:refnum<vi>)
  n21 = control-ref of="elements"() -> (w20:refnum<vi>)
  n22 = control-ref of="PLC Loop Rate Standard"() -> (w2:refnum<vi>)
  n23 = control-ref of="Modbus Loop Rate"() -> (w1:refnum<vi>)
  n24 = while {
    tunnel: w44 -> [w99]
    tunnel: [w96] -> w74
    shift-right: [w98] -> w71
    shift-left: w67 -> [w100]
    tunnel: w63 -> [w93]
    tunnel: w55 -> [w92]
    tunnel: w46 -> [w91]
    tunnel: w38 -> [w90]
    tunnel: w26 -> [w89]
    tunnel: w23 -> [w88]
    tunnel: w3 -> [w86]
    stop <- w97 stop-if-true
    # "FVIR\nAlicat"
    # "Event Handling Loop"
    n25 = event shown="[76] \"Manual Heating Value\": Value Change" {
      selector: w100 -> [_ _ _ _ _ _ _ _ _ _ _ _ _ _ _ _ _ _ _ _ _ _ _ _ _ _ _ _ _ _ _ _ _ _ _ _ _ _ _ _ _ _ _ _ _ _ _ _ _ _ _ _ _ _ _ _ _ _ _ _ _ _ _ _ _ _ _ _ _ _ _ _ _ _ _ _ _]
      dyn-events: [_ _ _ _ _ _ _ _ _ _ _ _ _ _ _ _ _ _ _ _ _ _ _ _ _ _ _ _ _ _ _ _ _ _ _ _ _ _ _ _ _ _ _ _ _ _ _ _ _ _ _ _ _ _ _ _ _ _ _ _ _ _ _ _ _ _ _ _ _ _ _ _ _ _ _ _ _] -> w98
      timeout: "Save Rate (ms)" -> [_ _ _ _ _ _ _ _ _ _ _ _ _ _ _ _ _ _ _ _ _ _ _ _ _ _ _ _ _ _ _ _ _ _ _ _ _ _ _ _ _ _ _ _ _ _ _ _ _ _ _ _ _ _ _ _ _ _ _ _ _ _ _ _ _ _ _ _ _ _ _ _ _ _ _ _ _]
      tunnel: [_ _ _ TRUE ("Discard?") _ _ _ _ _ _ _ _ _ _ _ _ _ _ _ _ _ _ _ _ _ _ _ _ _ _ _ _ _ _ _ _ _ _ _ _ _ _ _ _ _ _ _ _ _ _ _ _ _ _ _ _ _ _ _ _ _ _ _ _ _ _ _ _ _ _ _ _ _ _ _ _ _] -> w97
      tunnel: w99 -> [w102 w114 w118 w121 w127 w137 w143 w148 w153 w158 w163 w168 w173 w178 w182 w186 w190 w194 w200 w204 w209 w215 w220 w225 w233 w238 w243 w251 w256 w261 w271 w304 w325 w331 w337 w343 w348 w353 w355 w360 w365 w370 w379 w385 w390 w395 w400 w414 w423 w435 w441 w447 w452 w458 w476 w482 w488 w494 w500 w506 w512 w518 w524 w530 w536 w542 w548 w553 w558 w563 w571 w573 w580 w587 w593 w598 w612]
      tunnel: [w108 w112 w117 w119 w125 w135 w141 w146 w151 w156 w161 w166 w171 w176 w179 w183 w188 w191 w198 w201 w206 w213 w218 w224 w231 w236 w241 w249 w254 w259 w268 _ w323 w328 w335 w341 w346 w351 w356 w361 w366 w371 w375 w381 w386 w393 w401 w413 w426 w433 w439 w445 w451 w457 w474 w480 w486 w492 w498 w504 w510 w516 w521 w528 w533 w540 w546 w550 w555 w561 w568 w574 w577 w585 w591 w595 w610] -> w95
      tunnel: [w101 w113 w118 w121 w127 w134 w140 w145 w150 w155 w160 w165 w170 w175 w182 w186 w190 w193 w199 w202 w208 w212 w217 w223 w230 w235 w242 w248 w253 w260 w271 w304 w325 w331 w337 w343 w345 w350 w354 w359 w364 w369 w379 w385 w390 w395 w399 w414 w422 w432 w438 w444 w450 w456 w473 w479 w485 w491 w497 w503 w509 w515 w524 w530 w536 w539 w545 w553 w558 w563 w571 w572 w579 w584 w590 w597 w611] -> w94
      tunnel: w93 -> [_ _ _ _ _ _ _ _ _ _ _ _ _ _ _ _ w189 _ _ _ _ _ _ _ _ _ _ _ _ _ _ _ _ _ _ _ _ _ _ _ _ _ w377 w383 w388 w392 _ _ _ _ _ _ _ _ _ _ _ _ _ _ _ _ w522 w529 w534 _ _ _ _ w562 w569 _ _ _ _ _ _]
      tunnel: w92 -> [_ _ _ _ w126 _ _ _ _ _ _ _ _ _ w180 w184 _ _ _ _ _ _ _ _ _ _ _ _ _ _ _ _ _ _ _ _ _ _ _ _ _ _ _ _ _ _ _ _ _ _ _ _ _ _ _ _ _ _ _ _ _ _ _ _ _ _ _ _ _ _ _ _ _ _ _ _ _]
      tunnel: w91 -> [w107 w110 w117 w119 w123 w133 w139 w144 w149 w154 w159 w164 w169 w174 _ _ _ w192 w197 w203 w207 w211 w216 w221 w229 w234 w239 w247 w252 w257 w269 _ w324 w329 w336 w342 w344 w349 w357 w362 w367 w372 _ _ _ _ w402 w411 w425 w431 w437 w443 w449 w455 w472 w478 w484 w490 w496 w502 w508 w514 _ _ _ w538 w544 _ _ _ _ w575 w578 w583 w589 w596 _]
      tunnel: w90 -> [_ _ _ _ _ _ _ _ _ _ _ _ _ _ _ _ _ _ _ _ _ _ _ _ _ _ _ _ _ _ _ _ _ _ _ _ _ _ _ _ _ _ _ _ _ _ _ w412 _ _ _ _ _ _ _ _ _ _ _ _ _ _ _ _ _ _ _ w551 w556 _ _ _ _ _ _ _ _]
      tunnel: w89 -> [_ _ _ _ _ _ _ _ _ _ _ _ _ _ _ _ _ _ _ _ _ _ _ _ _ _ _ _ _ _ w265 _ w322 _ w334 _ _ _ _ _ _ _ _ _ _ _ _ _ _ _ _ _ _ _ _ _ _ _ _ _ _ _ _ _ _ _ _ _ _ _ _ _ _ _ _ _ _]
      tunnel: w88 -> [_ _ _ _ _ _ _ _ _ _ _ _ _ _ _ _ _ _ _ _ _ _ _ _ _ _ _ _ _ _ _ _ _ _ _ w339 _ _ _ _ _ _ _ _ _ _ _ _ _ _ _ _ _ _ _ _ _ _ _ _ _ _ _ _ _ _ _ _ _ _ _ _ _ _ _ _ _]
      tunnel: w86 -> [_ _ _ _ _ _ _ _ _ _ _ _ _ _ _ _ _ _ _ _ _ _ _ _ _ _ _ _ _ _ w266 _ _ w326 _ _ _ _ _ _ _ _ _ _ _ _ _ _ _ _ _ _ _ _ _ _ _ _ _ _ _ _ _ _ _ _ _ _ _ _ _ _ _ _ _ _ _]
      event Timeout {
        # "The timeout defines how frequencly data should be written to a logfile. When timeout is reach, a request for an additional Modbus read request is send to the Modbus Loop."
        n26 = event-data() -> ()  [unwired: 1 in, 1 out]
        n27 = call-poly "Enqueue Message.vi"("error in (no error)"=w107, "Message"="CheckBeforeWriteDataFVIR", "Message Queue"=w102) -> ("error out"=w104:errorcluster, "dup Message Queue"=w106:refnum<queue>)  [unwired: 7 in]
        n28 = call-poly "Enqueue Message.vi"("error in (no error)"=w104, "Message"="CheckBeforeWriteDataLDO", "Message Queue"=w106) -> ("error out"=w108:errorcluster, "dup Message Queue"=w101:refnum<queue>)  [unwired: 7 in]
      }
      event Panel Close? {
        # "Need to fix this!"
        # "Send the \"Exit\" message if the user closes the panel of the VI. Discard the event so the 'Confirm Quit' message has a chance to run."
        n29 = event-data() -> ()  [unwired: 1 in, 1 out]
        n30 = Stop(stop? (T)=TRUE) -> ()
        n31 = call-poly "Enqueue Message.vi"("Priority Message? (F)"=TRUE, "error in (no error)"=w110, "Message"="Exit", "Message Queue"=w114) -> ("error out"=w112:errorcluster, "dup Message Queue"=w113:refnum<queue>)  [unwired: 6 in]
        n32 = event-data("Discard?"=TRUE) -> ()  [unwired: 1 in, 1 out]
      }
      event Application Instance Close {
        n33 = event-data() -> ()  [unwired: 1 in, 1 out]
      }
      event User Event {
        w120 = "Exit" ("Exit String")
        # "The Message Handling Loop processed an \"Exit\" message, which fired this event to stop the Event Handling Loop."
        n34 = event-data() -> ()  [unwired: 1 in, 1 out]
        n35 = local write "FVIR Status"(w120) -> ()
        n36 = local write "LDO Status"(w120) -> ()
      }
      event "Start recording data - LDO": Value Change {
        n37 = event-data() -> ("NewVal"=w124:bool)  [unwired: 1 in]
        n38 = case shown="True" w124 {
          tunnel: w126 -> [_ w130]
          tunnel: [w128 w129] -> w125
          tunnel: w123 -> [w128 _]
          frame False {
          }
          frame True {
            n39 = call-poly "Enqueue Message.vi"("Message"="Tare_Totalizer_LDO", "Message Queue"=w130) -> ("error out"=w129:errorcluster)  [unwired: 8 in, 1 out]
          }
        }
      }
      event "Start Test Case LDO": Value Change {
        n40 = event-data() -> ()  [unwired: 1 in, 1 out]
        n41 = call-poly "Enqueue Message.vi"("error in (no error)"=w133, "Message"="StartTestCaseLDO", "Message Queue"=w137) -> ("error out"=w135:errorcluster, "dup Message Queue"=w134:refnum<queue>)  [unwired: 7 in]
        n42 = local write "PLC Loop Rate Standard"(u32 1000 ("PLC Loop Rate Standard")) -> ()
      }
      event "Stop Test Case LDO": Value Change {
        n43 = event-data() -> ()  [unwired: 1 in, 1 out]
        n44 = call-poly "Enqueue Message.vi"("error in (no error)"=w139, "Message"="StopTestCaseLDO", "Message Queue"=w143) -> ("error out"=w141:errorcluster, "dup Message Queue"=w140:refnum<queue>)  [unwired: 7 in]
        n45 = local write "PLC Loop Rate Standard"(u32 1000 ("PLC Loop Rate Standard")) -> ()
      }
      event "Send parameters to PLC LDO": Value Change {
        n46 = event-data() -> ()  [unwired: 1 in, 1 out]
        n47 = call-poly "Enqueue Message.vi"("error in (no error)"=w144, "Message"="SendParamToPLCLDO", "Message Queue"=w148) -> ("error out"=w146:errorcluster, "dup Message Queue"=w145:refnum<queue>)  [unwired: 7 in]
      }
      event "Water Outlet Valve Open LDO": Value Change {
        n48 = event-data() -> ()  [unwired: 1 in, 1 out]
        n49 = call-poly "Enqueue Message.vi"("error in (no error)"=w149, "Message"="WaterOutletOpenLDO", "Message Queue"=w153) -> ("error out"=w151:errorcluster, "dup Message Queue"=w150:refnum<queue>)  [unwired: 7 in]
      }
      event "Water Outlet Valve Close LDO": Value Change {
        n50 = event-data() -> ()  [unwired: 1 in, 1 out]
        n51 = call-poly "Enqueue Message.vi"("error in (no error)"=w154, "Message"="WaterOutletCloseLDO", "Message Queue"=w158) -> ("error out"=w156:errorcluster, "dup Message Queue"=w155:refnum<queue>)  [unwired: 7 in]
      }
      event "Water Inlet Valve Open LDO": Value Change {
        n52 = event-data() -> ()  [unwired: 1 in, 1 out]
        n53 = call-poly "Enqueue Message.vi"("error in (no error)"=w159, "Message"="WaterInletOpenLDO", "Message Queue"=w163) -> ("error out"=w161:errorcluster, "dup Message Queue"=w160:refnum<queue>)  [unwired: 7 in]
      }
      event "Water Inlet Valve Close LDO": Value Change {
        n54 = event-data() -> ()  [unwired: 1 in, 1 out]
        n55 = call-poly "Enqueue Message.vi"("error in (no error)"=w164, "Message"="WaterInletCloseLDO", "Message Queue"=w168) -> ("error out"=w166:errorcluster, "dup Message Queue"=w165:refnum<queue>)  [unwired: 7 in]
      }
      event "Gas Solenoid Valve Open LDO": Value Change {
        n56 = event-data() -> ()  [unwired: 1 in, 1 out]
        n57 = call-poly "Enqueue Message.vi"("error in (no error)"=w169, "Message"="GasSolenoidOpenLDO", "Message Queue"=w173) -> ("error out"=w171:errorcluster, "dup Message Queue"=w170:refnum<queue>)  [unwired: 7 in]
      }
      event "Gas Solenoid Valve Close LDO": Value Change {
        n58 = event-data() -> ()  [unwired: 1 in, 1 out]
        n59 = call-poly "Enqueue Message.vi"("error in (no error)"=w174, "Message"="GasSolenoidCloseLDO", "Message Queue"=w178) -> ("error out"=w176:errorcluster, "dup Message Queue"=w175:refnum<queue>)  [unwired: 7 in]
      }
      event "Gas Meter Tare Rate": Value Change {
        n60 = event-data() -> ()  [unwired: 1 in, 1 out]
        n61 = call-poly "Enqueue Message.vi"("Message"="Tare_Flow_LDO", "Message Queue"=w180) -> ("error out"=w179:errorcluster)  [unwired: 8 in, 1 out]
      }
      event "Gas Meter Tare Total": Value Change {
        n62 = event-data() -> ()  [unwired: 1 in, 1 out]
        n63 = call-poly "Enqueue Message.vi"("Message"="Tare_Totalizer_LDO", "Message Queue"=w184) -> ("error out"=w183:errorcluster)  [unwired: 8 in, 1 out]
      }
      event "Reset Flow Meter": Value Change {
        w187 = FALSE ("FVIR?")
        n64 = event-data() -> ()  [unwired: 1 in, 1 out]
        n65 = call "ResetFlowMeter.vi"("Initialize?"=w187, "FVIR?"=w187, "Modbus Queue in"=w189) -> ("error out"=w188:errorcluster)  [unwired: 7 in, 1 out]
      }
      event "Reset LDO Timers": Value Change {
        n66 = event-data() -> ()  [unwired: 1 in, 6 out]
        n67 = call-poly "Enqueue Message.vi"("error in (no error)"=w192, "Message"="ResetLDOTimer", "Message Queue"=w194) -> ("error out"=w191:errorcluster, "dup Message Queue"=w193:refnum<queue>)  [unwired: 7 in]
      }
      event "Start Intellifaucet DRK375 - LDO": Value Change {
        n68 = event-data() -> ()  [unwired: 1 in, 1 out]
        n69 = call "Intellifaucet_Control.vi"("Type"=StartStopIntellifaucet."Start LDO" ("Enum"), "error in (no error)"=w197, "Queue in"=w200) -> ("error out"=w198:errorcluster, "Queue out"=w199:refnum<queue>)  [unwired: 7 in]
      }
      event "Stop Intellifaucet DRK375 - LDO": Value Change {
        n70 = event-data() -> ()  [unwired: 1 in, 1 out]
        n71 = call "Intellifaucet_Control.vi"("Type"=StartStopIntellifaucet."Stop LDO" ("Enum"), "error in (no error)"=w203, "Queue in"=w204) -> ("error out"=w201:errorcluster, "Queue out"=w202:refnum<queue>)  [unwired: 7 in]
      }
      event "Clear Unist Alarm": Value Change {
        n72 = event-data() -> ()  [unwired: 1 in, 6 out]
        n73 = call-poly "Enqueue Message.vi"("error in (no error)"=w207, "Message"="Oil_Alarm", "Message Queue"=w209) -> ("error out"=w206:errorcluster, "dup Message Queue"=w208:refnum<queue>)  [unwired: 7 in]
      }
      event "Oil Spray 0.8 cc/min Open": Value Change {
        n74 = event-data() -> ()  [unwired: 1 in, 1 out]
        n75 = call-poly "Enqueue Message.vi"("error in (no error)"=w211, "Message"="OilSpray08Open", "Message Queue"=w215) -> ("error out"=w213:errorcluster, "dup Message Queue"=w212:refnum<queue>)  [unwired: 7 in]
      }
      event "Oil Spray 0.8 cc/min Close": Value Change {
        n76 = event-data() -> ()  [unwired: 1 in, 1 out]
        n77 = call-poly "Enqueue Message.vi"("error in (no error)"=w216, "Message"="OilSpray08Close", "Message Queue"=w220) -> ("error out"=w218:errorcluster, "dup Message Queue"=w217:refnum<queue>)  [unwired: 7 in]
      }
      event "Oil spray 0.8cc/min": Value Change {
        n78 = event-data() -> ("NewVal"=w226:bool)  [unwired: 1 in]
        n79 = case shown="False" w226 {
          tunnel: ["OilSpray08Close" ("Message") "OilSpray08Open" ("Message")] -> w222
          frame False {
          }
          frame True {
          }
        }
        n80 = call-poly "Enqueue Message.vi"("error in (no error)"=w221, "Message"=w222, "Message Queue"=w225) -> ("error out"=w224:errorcluster, "dup Message Queue"=w223:refnum<queue>)  [unwired: 7 in]
      }
      event "Oil Spray 1.1 cc/min Open": Value Change {
        n81 = event-data() -> ()  [unwired: 1 in, 1 out]
        n82 = call-poly "Enqueue Message.vi"("error in (no error)"=w229, "Message"="OilSpray11Open", "Message Queue"=w233) -> ("error out"=w231:errorcluster, "dup Message Queue"=w230:refnum<queue>)  [unwired: 7 in]
      }
      event "Oil Spray 1.1 cc/min Close": Value Change {
        n83 = event-data() -> ()  [unwired: 1 in, 1 out]
        n84 = call-poly "Enqueue Message.vi"("error in (no error)"=w234, "Message"="OilSpray11Close", "Message Queue"=w238) -> ("error out"=w236:errorcluster, "dup Message Queue"=w235:refnum<queue>)  [unwired: 7 in]
      }
      event "Oil spray 1.1cc/min": Value Change {
        n85 = event-data() -> ("NewVal"=w240:bool)  [unwired: 1 in]
        n86 = case shown="True" w240 {
          tunnel: ["OilSpray11Close" ("Message") "OilSpray11Open" ("Message")] -> w244
          frame False {
          }
          frame True {
          }
        }
        n87 = call-poly "Enqueue Message.vi"("error in (no error)"=w239, "Message"=w244, "Message Queue"=w243) -> ("error out"=w241:errorcluster, "dup Message Queue"=w242:refnum<queue>)  [unwired: 7 in]
      }
      event "Oil Spray 1.33 cc/min Open": Value Change {
        n88 = event-data() -> ()  [unwired: 1 in, 1 out]
        n89 = call-poly "Enqueue Message.vi"("error in (no error)"=w247, "Message"="OilSpray133Open", "Message Queue"=w251) -> ("error out"=w249:errorcluster, "dup Message Queue"=w248:refnum<queue>)  [unwired: 7 in]
      }
      event "Oil Spray 1.33 cc/min Close": Value Change {
        n90 = event-data() -> ()  [unwired: 1 in, 1 out]
        n91 = call-poly "Enqueue Message.vi"("error in (no error)"=w252, "Message"="OilSpray133Close", "Message Queue"=w256) -> ("error out"=w254:errorcluster, "dup Message Queue"=w253:refnum<queue>)  [unwired: 7 in]
      }
      event "Oil spray 1.33cc/min": Value Change {
        n92 = event-data() -> ("NewVal"=w258:bool)  [unwired: 1 in]
        n93 = case shown="True" w258 {
          tunnel: ["OilSpray133Close" ("Message") "OilSpray133Open" ("Message")] -> w262
          frame False {
          }
          frame True {
          }
        }
        n94 = call-poly "Enqueue Message.vi"("error in (no error)"=w257, "Message"=w262, "Message Queue"=w261) -> ("error out"=w259:errorcluster, "dup Message Queue"=w260:refnum<queue>)  [unwired: 7 in]
      }
      event "Rotary Actuator (ON/OFF)": Value Change {
        n95 = event-data() -> ("NewVal"=w270:bool)  [unwired: 1 in]
        n96 = case shown="\"Power Vent\"" "Product Type" {
          tunnel: w270 -> [_ w278 w289]
          tunnel: w269 -> [w272 w277 w290]
          tunnel: w266 -> [_ _ w291]
          tunnel: [w272 w276 w292] -> w268
          tunnel: w265 -> [_ w273 _]
          frame "", Default {
          }
          frame "Standard ATM" {
            n97 = case shown="False" w278 {
              tunnel: "Vesta ON Temperature LDO" -> [_ w285]
              tunnel: "Vesta OFF Temperature LDO" -> [w280 _]
              tunnel: [w282 w287] -> w276
              tunnel: w277 -> [w281 w286]
              tunnel: w273 -> [w279 w284]
              frame False {
                n98 = call-poly "Enqueue Message.vi"("error in (no error)"=w281, "Message Data"=w280, "Message"="PUT_Vesta_Temp_LDO", "Message Queue"=w279) -> ("error out"=w282:errorcluster)  [unwired: 6 in, 1 out]
              }
              frame True {
                n99 = call-poly "Enqueue Message.vi"("error in (no error)"=w286, "Message Data"=w285, "Message"="PUT_Vesta_Temp_LDO", "Message Queue"=w284) -> ("error out"=w287:errorcluster)  [unwired: 6 in, 1 out]
              }
            }
          }
          frame "Power Vent" {
            n100 = case shown="True" w289 {
              tunnel: [w296 w301] -> w292
              tunnel: w290 -> [w295 w300]
              tunnel: w291 -> [w294 w299]
              frame False {
                w293 = FALSE  # Turn OFF Heater
                n101 = call-poly "Enqueue Message.vi"("error in (no error)"=w295, "Message Data"=w293, "Message"="PUT_EnviraCom_Temp_LDO", "Message Queue"=w294) -> ("error out"=w296:errorcluster)  [unwired: 6 in, 1 out]
              }
              frame True {
                w298 = TRUE  # Turn ON Heater
                n102 = call-poly "Enqueue Message.vi"("error in (no error)"=w300, "Message Data"=w298, "Message"="PUT_EnviraCom_Temp_LDO", "Message Queue"=w299) -> ("error out"=w301:errorcluster)  [unwired: 6 in, 1 out]
              }
            }
          }
        }
      }
      event Value Change {
        n103 = event-data() -> ("NewVal"=w303:T4)  [unwired: 1 in, 5 out]
        n104 = case shown="\"Power Vent\"" w303 {
          frame "Standard ATM" {
            n105 = property on="Temperature Parameters" class="Clust (strict)"("DisabledEnum"=T23."Enabled" ("Disabled")) -> ()  [unwired: 2 in, 2 out]
            n106 = property on="Water Heater Temperature (°F)" class="Bool"("DisabledEnum"=T23."Enabled" ("Disabled")) -> ()  [unwired: 2 in, 2 out]
            n107 = property on="Reset BINs" class="Bool"("DisabledEnum"=T23."Enabled" ("Disabled")) -> ()  [unwired: 2 in, 2 out]
            n108 = property on="EnviraCom (On/Off)" class="Bool (strict)"("DisabledEnum"=T23."Disabled and Grayed Out" ("Disabled")) -> ()  [unwired: 2 in, 2 out]
            n109 = property on="SET Temperature (°F)-EnviraCom" class="Bool"("DisabledEnum"=T23."Disabled and Grayed Out" ("Disabled")) -> ()  [unwired: 2 in, 2 out]
          }
          frame "Power Vent" {
            n110 = property on="Temperature Parameters" class="Clust (strict)"("DisabledEnum"=T23."Disabled and Grayed Out" ("Disabled")) -> ()  [unwired: 2 in, 2 out]
            n111 = property on="Water Heater Temperature (°F)" class="Bool"("DisabledEnum"=T23."Disabled and Grayed Out" ("Disabled")) -> ()  [unwired: 2 in, 2 out]
            n112 = property on="Reset BINs" class="Bool"("DisabledEnum"=T23."Disabled and Grayed Out" ("Disabled")) -> ()  [unwired: 2 in, 2 out]
            n113 = property on="EnviraCom (On/Off)" class="Bool (strict)"("DisabledEnum"=T23."Enabled" ("Disabled")) -> ()  [unwired: 2 in, 2 out]
            n114 = property on="SET Temperature (°F)-EnviraCom" class="Bool"("DisabledEnum"=T23."Enabled" ("Disabled")) -> ()  [unwired: 2 in, 2 out]
          }
          frame Default {
            n115 = property on="Temperature Parameters" class="Clust (strict)"("DisabledEnum"=T23."Disabled and Grayed Out" ("Disabled")) -> ()  [unwired: 2 in, 2 out]
            n116 = property on="Water Heater Temperature (°F)" class="Bool"("DisabledEnum"=T23."Disabled and Grayed Out" ("Disabled")) -> ()  [unwired: 2 in, 2 out]
            n117 = property on="Reset BINs" class="Bool"("DisabledEnum"=T23."Disabled and Grayed Out" ("Disabled")) -> ()  [unwired: 2 in, 2 out]
            n118 = property on="EnviraCom (On/Off)" class="Bool (strict)"("DisabledEnum"=T23."Disabled and Grayed Out" ("Disabled")) -> ()  [unwired: 2 in, 2 out]
            n119 = property on="SET Temperature (°F)-EnviraCom" class="Bool"("DisabledEnum"=T23."Disabled and Grayed Out" ("Disabled")) -> ()  [unwired: 2 in, 2 out]
          }
        }
      }
      event "Water Heater Temperature (°F)": Value Change {
        n120 = event-data() -> ()  [unwired: 1 in, 1 out]
        n121 = call-poly "Enqueue Message.vi"("error in (no error)"=w324, "Message Data"="Temperature Parameters", "Message"="PUT_Vesta_Temp_LDO", "Message Queue"=w322) -> ("error out"=w323:errorcluster)  [unwired: 6 in, 1 out]
      }
      event "SET Temperature (°F)-EnviraCom": Value Change {
        n122 = event-data() -> ()  [unwired: 1 in, 6 out]
        n123 = call-poly "Enqueue Message.vi"("error in (no error)"=w329, "Message Data"="EnviraCom (On/Off)", "Message"="PUT_EnviraCom_Temp_LDO", "Message Queue"=w326) -> ("error out"=w328:errorcluster)  [unwired: 6 in, 1 out]
      }
      event "Reset BINs": Value Change {
        # "Setting the temperature to zero\nwill reset the BINs. It has to be in\ncooling state."
        n124 = event-data() -> ()  [unwired: 1 in, 1 out]
        n125 = call-poly "Enqueue Message.vi"("error in (no error)"=w336, "Message Data"=T3 {"Water Heater Temp (°F)"=0, "Differential  (°F)"=10.0} ("Temperature Parameters 2"), "Message"="PUT_Vesta_Temp_LDO", "Message Queue"=w334) -> ("error out"=w335:errorcluster)  [unwired: 6 in, 1 out]
      }
      event "Water Heater Temperature (°F) FVIR": Value Change {
        n126 = event-data() -> ()  [unwired: 1 in, 1 out]
        n127 = call-poly "Enqueue Message.vi"("error in (no error)"=w342, "Message Data"="Water Heater Temp (°F) FVIR 2", "Message"="PUT_Vesta_Temp_FVIR", "Message Queue"=w339) -> ("error out"=w341:errorcluster)  [unwired: 6 in, 1 out]
      }
      event "Rotary Actuator ON": Value Change {
        n128 = event-data() -> ()  [unwired: 1 in, 1 out]
        n129 = call-poly "Enqueue Message.vi"("error in (no error)"=w344, "Message"="HeaterON_LDO", "Message Queue"=w348) -> ("error out"=w346:errorcluster, "dup Message Queue"=w345:refnum<queue>)  [unwired: 7 in]
      }
      event "Rotary Actuator OFF": Value Change {
        n130 = event-data() -> ()  [unwired: 1 in, 1 out]
        n131 = call-poly "Enqueue Message.vi"("error in (no error)"=w349, "Message"="HeaterOFF_LDO", "Message Queue"=w353) -> ("error out"=w351:errorcluster, "dup Message Queue"=w350:refnum<queue>)  [unwired: 7 in]
      }
      event "Conveyor ON": Value Change {
        n132 = event-data() -> ()  [unwired: 1 in, 6 out]
        n133 = call-poly "Enqueue Message.vi"("error in (no error)"=w357, "Message"="ConveyorON", "Message Queue"=w355) -> ("error out"=w356:errorcluster, "dup Message Queue"=w354:refnum<queue>)  [unwired: 7 in]
      }
      event "Conveyor OFF": Value Change {
        n134 = event-data() -> ()  [unwired: 1 in, 6 out]
        n135 = call-poly "Enqueue Message.vi"("error in (no error)"=w362, "Message"="ConveyorOFF", "Message Queue"=w360) -> ("error out"=w361:errorcluster, "dup Message Queue"=w359:refnum<queue>)  [unwired: 7 in]
      }
      event "Blower ON": Value Change {
        n136 = event-data() -> ()  [unwired: 1 in, 6 out]
        n137 = call-poly "Enqueue Message.vi"("error in (no error)"=w367, "Message"="BlowerON", "Message Queue"=w365) -> ("error out"=w366:errorcluster, "dup Message Queue"=w364:refnum<queue>)  [unwired: 7 in]
      }
      event "Blower OFF": Value Change {
        n138 = event-data() -> ()  [unwired: 1 in, 6 out]
        n139 = call-poly "Enqueue Message.vi"("error in (no error)"=w372, "Message"="BlowerOFF", "Message Queue"=w370) -> ("error out"=w371:errorcluster, "dup Message Queue"=w369:refnum<queue>)  [unwired: 7 in]
      }
      event "Temp (°F)-LDO": Value Change {
        n140 = event-data() -> ()  [unwired: 1 in, 1 out]
        n141 = call-poly "Enqueue Message.vi"("Priority Message? (F)"=TRUE, "Message Data"="Temp (°F)-LDO", "Message"="TempChangeDRK375_LDO", "Message Queue"=w377) -> ("error out"=w375:errorcluster)  [unwired: 6 in, 1 out]
      }
      event "Valve % Open - LDO": Value Change {
        n142 = event-data() -> ()  [unwired: 1 in, 1 out]
        n143 = call-poly "Enqueue Message.vi"("Priority Message? (F)"=TRUE, "Message Data"="Valve % Open - LDO", "Message"="ValveChangeDRK375_LDO", "Message Queue"=w383) -> ("error out"=w381:errorcluster)  [unwired: 6 in, 1 out]
      }
      event "Proportioning Valve - LDO": Value Change {
        n144 = event-data() -> ()  [unwired: 1 in, 1 out]
        n145 = call-poly "Enqueue Message.vi"("Message Data"="Proportioning Valve - LDO", "Message"="ValveChangeEPV_LDO", "Message Queue"=w388) -> ("error out"=w386:errorcluster)  [unwired: 7 in, 1 out]
      }
      event "Burner-LDO": Value Change {
        n146 = event-data() -> ("NewVal"=w394:bool)  [unwired: 1 in, 5 out]
        n147 = case shown="False" w394 {
          tunnel: ["Water_Heater_Status_OFF_LDO" ("Message") "Water_Heater_Status_ON_LDO" ("Message")] -> w391
          frame False {
          }
          frame True {
          }
        }
        n148 = call-poly "Enqueue Message.vi"("Message"=w391, "Message Queue"=w392) -> ("error out"=w393:errorcluster)  [unwired: 8 in, 1 out]
      }
      event "Start ANSI LDO": Value Change {
        n149 = event-data() -> ("NewVal"=w398:bool)  [unwired: 1 in]
        n150 = case shown="True" w398 {
          tunnel: w402 -> [w403 w409]
          tunnel: [w403 w408] -> w401
          tunnel: w400 -> [w404 w407]
          tunnel: [w404 w406] -> w399
          frame False {
          }
          frame True {
            n151 = call-poly "Enqueue Message.vi"("error in (no error)"=w409, "Message"="Start ANSI LDO", "Message Queue"=w407) -> ("error out"=w408:errorcluster, "dup Message Queue"=w406:refnum<queue>)  [unwired: 7 in]
          }
        }
      }
      event "Start recording data - FVIR": Value Change {
        n152 = event-data() -> ("NewVal"=w410:bool)  [unwired: 1 in]
        n153 = case shown="True" w410 {
          tunnel: w412 -> [_ w418]
          tunnel: [w415 w417] -> w413
          tunnel: w411 -> [w415 _]
          frame False {
          }
          frame True {
            n154 = call-poly "Enqueue Message.vi"("Priority Message? (F)"=TRUE, "Message"="Tare_Totalizer_FVIR", "Message Queue"=w418) -> ("error out"=w417:errorcluster)  [unwired: 7 in, 1 out]
          }
        }
      }
      event "Start Test Case FVIR": Value Change {
        n155 = event-data() -> ()  [unwired: 1 in, 1 out]
        n156 = call-poly "Enqueue Message.vi"("Priority Message? (F)"=TRUE, "error in (no error)"=w425, "Message"="StartTestCaseFVIR", "Message Queue"=w423) -> ("error out"=w426:errorcluster, "dup Message Queue"=w422:refnum<queue>)  [unwired: 6 in]
        n157 = local write "Save Rate (ms)"("FVIR Save Rate (Default ms)") -> ()
        n158 = local write "PLC Loop Rate Standard"(u32 500 ("PLC Loop Rate Standard")) -> ()
      }
      event "Stop Test Case FVIR": Value Change {
        n159 = event-data() -> ()  [unwired: 1 in, 1 out]
        n160 = call-poly "Enqueue Message.vi"("Priority Message? (F)"=TRUE, "error in (no error)"=w431, "Message"="StopTestCaseFVIR", "Message Queue"=w435) -> ("error out"=w433:errorcluster, "dup Message Queue"=w432:refnum<queue>)  [unwired: 6 in]
        n161 = local write "PLC Loop Rate Standard"(u32 1000 ("PLC Loop Rate Standard")) -> ()
        n162 = local write "Save Rate (ms)"(10000 ("Save Rate (ms)")) -> ()
      }
      event "Send parameters to PLC FVIR": Value Change {
        n163 = event-data() -> ()  [unwired: 1 in, 1 out]
        n164 = call-poly "Enqueue Message.vi"("Priority Message? (F)"=TRUE, "error in (no error)"=w437, "Message"="SendParamToPLCFVIR", "Message Queue"=w441) -> ("error out"=w439:errorcluster, "dup Message Queue"=w438:refnum<queue>)  [unwired: 6 in]
      }
      event "Start - SRI Log": Value Change {
        n165 = event-data() -> ()  [unwired: 1 in, 1 out]
        n166 = call-poly "Enqueue Message.vi"("Priority Message? (F)"=TRUE, "error in (no error)"=w443, "Message"="Start SRI Log", "Message Queue"=w447) -> ("error out"=w445:errorcluster, "dup Message Queue"=w444:refnum<queue>)  [unwired: 6 in]
      }
      event "Stop- SRI Log": Value Change {
        n167 = event-data() -> ()  [unwired: 1 in, 1 out]
        n168 = call-poly "Enqueue Message.vi"("Priority Message? (F)"=TRUE, "error in (no error)"=w449, "Message"="Start SRI Log", "Message Queue"=w452) -> ("error out"=w451:errorcluster, "dup Message Queue"=w450:refnum<queue>)  [unwired: 6 in]
      }
      event "Full Mannequin Sequence": Value Change {
        n169 = event-data() -> ("NewVal"=w454:bool)  [unwired: 1 in]
        n170 = case shown="True" w454 {
          tunnel: w458 -> [w461 w470]
          tunnel: [w460 w468] -> w457
          tunnel: [w459 w467] -> w456
          tunnel: w455 -> [w462 w466]
          frame False {
            n171 = call-poly "Enqueue Message.vi"("Priority Message? (F)"=TRUE, "error in (no error)"=w462, "Message"="StopManSeq", "Message Queue"=w461) -> ("error out"=w460:errorcluster, "dup Message Queue"=w459:refnum<queue>)  [unwired: 6 in]
          }
          frame True {
            n172 = call-poly "Enqueue Message.vi"("Priority Message? (F)"=TRUE, "error in (no error)"=w466, "Message"="StartManSeq", "Message Queue"=w470) -> ("error out"=w468:errorcluster, "dup Message Queue"=w467:refnum<queue>)  [unwired: 6 in]
          }
        }
      }
      event "Move mannequin - Go to Home Pos": Value Change {
        n173 = event-data() -> ()  [unwired: 1 in, 1 out]
        n174 = call-poly "Enqueue Message.vi"("Priority Message? (F)"=TRUE, "error in (no error)"=w472, "Message"="MannequinHomePos", "Message Queue"=w476) -> ("error out"=w474:errorcluster, "dup Message Queue"=w473:refnum<queue>)  [unwired: 6 in]
      }
      event "Move mannequin - Go to Work Pos": Value Change {
        n175 = event-data() -> ()  [unwired: 1 in, 1 out]
        n176 = call-poly "Enqueue Message.vi"("Priority Message? (F)"=TRUE, "error in (no error)"=w478, "Message"="MannequinWorkPos", "Message Queue"=w482) -> ("error out"=w480:errorcluster, "dup Message Queue"=w479:refnum<queue>)  [unwired: 6 in]
      }
      event "Spill can - Go to Home Pos": Value Change {
        n177 = event-data() -> ()  [unwired: 1 in, 1 out]
        n178 = call-poly "Enqueue Message.vi"("Priority Message? (F)"=TRUE, "error in (no error)"=w484, "Message"="SpillCanHomePos", "Message Queue"=w488) -> ("error out"=w486:errorcluster, "dup Message Queue"=w485:refnum<queue>)  [unwired: 6 in]
      }
      event "Spill can - Go to Work Pos": Value Change {
        n179 = event-data() -> ()  [unwired: 1 in, 1 out]
        n180 = call-poly "Enqueue Message.vi"("Priority Message? (F)"=TRUE, "error in (no error)"=w490, "Message"="SpillCanWorkPos", "Message Queue"=w494) -> ("error out"=w492:errorcluster, "dup Message Queue"=w491:refnum<queue>)  [unwired: 6 in]
      }
      event "Water Outlet Valve Open FVIR": Value Change {
        n181 = event-data() -> ()  [unwired: 1 in, 1 out]
        n182 = call-poly "Enqueue Message.vi"("Priority Message? (F)"=TRUE, "error in (no error)"=w496, "Message"="WaterOutletOpenFVIR", "Message Queue"=w500) -> ("error out"=w498:errorcluster, "dup Message Queue"=w497:refnum<queue>)  [unwired: 6 in]
      }
      event "Water Outlet Valve Close FVIR": Value Change {
        n183 = event-data() -> ()  [unwired: 1 in, 1 out]
        n184 = call-poly "Enqueue Message.vi"("Priority Message? (F)"=TRUE, "error in (no error)"=w502, "Message"="WaterOutletCloseFVIR", "Message Queue"=w506) -> ("error out"=w504:errorcluster, "dup Message Queue"=w503:refnum<queue>)  [unwired: 6 in]
      }
      event "Water Inlet Valve Open FVIR": Value Change {
        n185 = event-data() -> ()  [unwired: 1 in, 1 out]
        n186 = call-poly "Enqueue Message.vi"("Priority Message? (F)"=TRUE, "error in (no error)"=w508, "Message"="WaterInletOpenFVIR", "Message Queue"=w512) -> ("error out"=w510:errorcluster, "dup Message Queue"=w509:refnum<queue>)  [unwired: 6 in]
      }
      event "Water Inlet Valve Close FVIR": Value Change {
        n187 = event-data() -> ()  [unwired: 1 in, 1 out]
        n188 = call-poly "Enqueue Message.vi"("Priority Message? (F)"=TRUE, "error in (no error)"=w514, "Message"="WaterInletCloseFVIR", "Message Queue"=w518) -> ("error out"=w516:errorcluster, "dup Message Queue"=w515:refnum<queue>)  [unwired: 6 in]
      }
      event "Temp (°F)-FVIR": Value Change {
        n189 = event-data() -> ()  [unwired: 1 in, 1 out]
        n190 = call-poly "Enqueue Message.vi"("Priority Message? (F)"=TRUE, "Message Data"="Temp (°F)-FVIR", "Message"="TempChangeDRK375_FVIR", "Message Queue"=w522) -> ("error out"=w521:errorcluster)  [unwired: 6 in, 1 out]
      }
      event "Valve % Open - FVIR": Value Change {
        n191 = event-data() -> ()  [unwired: 1 in, 1 out]
        n192 = call-poly "Enqueue Message.vi"("Priority Message? (F)"=TRUE, "Message Data"="Valve % Open - FVIR", "Message"="ValveChangeDRK375_FVIR", "Message Queue"=w529) -> ("error out"=w528:errorcluster)  [unwired: 6 in, 1 out]
      }
      event "Proportioning Valve - FVIR": Value Change {
        n193 = event-data() -> ()  [unwired: 1 in, 6 out]
        n194 = call-poly "Enqueue Message.vi"("Priority Message? (F)"=TRUE, "Message Data"="Proportioning Valve - FVIR", "Message"="ValveChangeEPV_FVIR", "Message Queue"=w534) -> ("error out"=w533:errorcluster)  [unwired: 6 in, 1 out]
      }
      event "Gas Solenoid Valve Open FVIR": Value Change {
        n195 = event-data() -> ()  [unwired: 1 in, 1 out]
        n196 = call-poly "Enqueue Message.vi"("Priority Message? (F)"=TRUE, "error in (no error)"=w538, "Message"="GasSolenoidOpenFVIR", "Message Queue"=w542) -> ("error out"=w540:errorcluster, "dup Message Queue"=w539:refnum<queue>)  [unwired: 6 in]
      }
      event "Gas Solenoid Valve Close FVIR": Value Change {
        n197 = event-data() -> ()  [unwired: 1 in, 1 out]
        n198 = call-poly "Enqueue Message.vi"("Priority Message? (F)"=TRUE, "error in (no error)"=w544, "Message"="GasSolenoidCloseFVIR", "Message Queue"=w548) -> ("error out"=w546:errorcluster, "dup Message Queue"=w545:refnum<queue>)  [unwired: 6 in]
      }
      event "Gas Meter Tare Rate FVIR": Value Change {
        n199 = event-data() -> ()  [unwired: 1 in, 6 out]
        n200 = call-poly "Enqueue Message.vi"("Priority Message? (F)"=TRUE, "Message"="Tare_Flow_FVIR", "Message Queue"=w551) -> ("error out"=w550:errorcluster)  [unwired: 7 in, 1 out]
      }
      event "Gas Meter Tare Total FVIR": Value Change {
        n201 = event-data() -> ()  [unwired: 1 in, 6 out]
        n202 = call-poly "Enqueue Message.vi"("Priority Message? (F)"=TRUE, "Message"="Tare_Totalizer_FVIR", "Message Queue"=w556) -> ("error out"=w555:errorcluster)  [unwired: 7 in, 1 out]
      }
      event "Burner-FVIR": Value Change {
        n203 = event-data() -> ("NewVal"=w560:bool)  [unwired: 1 in, 5 out]
        n204 = case shown="True" w560 {
          tunnel: ["Water_Heater_Status_OFF_FVIR" ("Message") "Water_Heater_Status_ON_FVIR" ("Message")] -> w564
          frame False {
          }
          frame True {
          }
        }
        n205 = call-poly "Enqueue Message.vi"("Priority Message? (F)"=TRUE, "Message"=w564, "Message Queue"=w562) -> ("error out"=w561:errorcluster)  [unwired: 7 in, 1 out]
      }
      event "Reset Flow Meter FVIR": Value Change {
        n206 = event-data() -> ()  [unwired: 1 in, 6 out]
        n207 = call "ResetFlowMeter.vi"("Initialize?"=FALSE, "FVIR?"=TRUE, "Modbus Queue in"=w569) -> ("error out"=w568:errorcluster)  [unwired: 7 in, 1 out]
      }
      event "Start Intellifaucet DRK375 - FVIR": Value Change {
        n208 = event-data() -> ()  [unwired: 1 in, 6 out]
        n209 = call "Intellifaucet_Control.vi"("Type"=StartStopIntellifaucet."Start FVIR" ("Enum"), "error in (no error)"=w575, "Queue in"=w573) -> ("error out"=w574:errorcluster, "Queue out"=w572:refnum<queue>)  [unwired: 7 in]
      }
      event "Stop Intellifaucet DRK375 - FVIR": Value Change {
        n210 = event-data() -> ()  [unwired: 1 in, 6 out]
        n211 = call "Intellifaucet_Control.vi"("Type"=StartStopIntellifaucet."Stop FVIR" ("Enum"), "error in (no error)"=w578, "Queue in"=w580) -> ("error out"=w577:errorcluster, "Queue out"=w579:refnum<queue>)  [unwired: 7 in]
      }
      event "Burner ON FVIR": Value Change {
        n212 = event-data() -> ()  [unwired: 1 in, 1 out]
        n213 = call-poly "Enqueue Message.vi"("Priority Message? (F)"=TRUE, "error in (no error)"=w583, "Message"="HeaterON_FVIR", "Message Queue"=w587) -> ("error out"=w585:errorcluster, "dup Message Queue"=w584:refnum<queue>)  [unwired: 6 in]
      }
      event "Burner OFF FVIR": Value Change {
        n214 = event-data() -> ()  [unwired: 1 in, 1 out]
        n215 = call-poly "Enqueue Message.vi"("Priority Message? (F)"=TRUE, "error in (no error)"=w589, "Message"="HeaterOFF_FVIR", "Message Queue"=w593) -> ("error out"=w591:errorcluster, "dup Message Queue"=w590:refnum<queue>)  [unwired: 6 in]
      }
      event "Start ANSI FVIR": Value Change {
        n216 = event-data() -> ("NewVal"=w594:bool)  [unwired: 1 in]
        n217 = case shown="True" w594 {
          tunnel: w598 -> [w600 w605]
          tunnel: [w600 w604] -> w597
          tunnel: w596 -> [w599 w603]
          tunnel: [w599 w602] -> w595
          frame False {
          }
          frame True {
            n218 = call-poly "Enqueue Message.vi"("Priority Message? (F)"=TRUE, "error in (no error)"=w603, "Message"="Start ANSI FVIR", "Message Queue"=w605) -> ("error out"=w602:errorcluster, "dup Message Queue"=w604:refnum<queue>)  [unwired: 6 in]
          }
        }
      }
      event "Manual Heating Value": Value Change {
        n219 = event-data() -> ("NewVal"=w607:bool)  [unwired: 1 in]
        n220 = call-poly "Enqueue Message.vi"("Priority Message? (F)"=TRUE, "Message Data"=w607, "Message"="Manual_Heating_Value_UI", "Message Queue"=w612) -> ("error out"=w610:errorcluster, "dup Message Queue"=w611:refnum<queue>)  [unwired: 6 in]
      }
    }
    n221 = call "Error Handler - Event Handling Loop.vi"("error in (no error)"=w95, "Message Queue"=w94) -> ("dup error in"=w96:errorcluster)  [unwired: 8 in, 1 out]
  }
  n222 = control-ref of="LDO - Filepath"() -> (w12:refnum<vi>)
  n223 = control-ref of="FVIR - Filepath"() -> (w13:refnum<vi>)
  n224 = control-ref of="Vesta is working"() -> (w14:refnum<vi>)
  n225 = control-ref of="EnviraCom is working"() -> (w4:refnum<vi>)
  n226 = control-ref of="Retry Count"() -> (w15:refnum<vi>)
  n227 = control-ref of="Vesta LDO Loop Count"() -> (w16:refnum<vi>)
  n228 = control-ref of="Retry Count"() -> (w7:refnum<vi>)
  n229 = control-ref of="EnviraCom LDO Loop Count"() -> (w5:refnum<vi>)
  n230 = control-ref of="Vesta LDO State"() -> (w17:refnum<vi>)
  n231 = control-ref of="EnviraCom LDO State"() -> (w6:refnum<vi>)
  n232 = call "Modbus Message Loop.vi"("Elements"=w20, "Loop Rate Standard"=w2, "States"=w22, "Loop Rate"=w1, "error in (no error)"=w11, "Input Registers"=w21, "PLC IP address"="PLC IP address", "Message Queues in"=w9) -> ("error out"=w62:errorcluster)  [unwired: 3 in]
  n233 = call "SRI8610C-DataFile Message Loop.vi"("error in (no error)"=w11, "Message Queues"=w9) -> ("error out"=w29:errorcluster)  [unwired: 8 in]
  n234 = call "WritingDataFile Message Loop.vi"("FV Ref"=w13, "LDO Ref"=w12, "error in (no error)"=w11, "Message Queues"=w9) -> ("error out"=w61:errorcluster)  [unwired: 7 in]
  n235 = call "FVIR_LDO_Oil_Machine.vi"("error in"=w11, "Message Queues"=w9) -> ("error out"=w59:errorcluster)  [unwired: 9 in]
  n236 = call "LDO_Alicat_GasMeter.vi"("error in"=w11, "VISA Refnum in"="LDO Alicat VISA", "Message Queues"=w9) -> ("error out"=w52:errorcluster)  [unwired: 8 in]
  n237 = call "FVIR_Alicat_GasMeter.vi"("error in"=w11, "VISA Refnum in"="FVIR Alicat VISA", "Message Queues"=w9) -> ("error out"=w43:errorcluster)  [unwired: 8 in]
  n238 = call "FVIR_LDO_Inficon.vi"("error in"=w11, "Remote IP Address"="Inficon IP Address", "Message Queues"=w9) -> ("error out"=w51:errorcluster)  [unwired: 8 in]
  n239 = call "LDO_Ultramat_23.vi"("error in"=w11, "VISA resource name"="Ultramat 23_LDO", "Message Queues"=w9) -> ("error out"=w50:errorcluster)  [unwired: 8 in]
  n240 = call "FVIR_Ultramat_23.vi"("error in"=w11, "VISA resource name"="Ultramat 23_FVIR", "Message Queues"=w9) -> ("error out"=w37:errorcluster)  [unwired: 8 in]
  n241 = call "LDO_VESTA_Main.vi"("Vesta is working"=w14, "Loop Count"=w16, "State"=w17, "error in"=w11, "Retry Count"=w15, "VISA resource name"="VESTA LDO COM", "Message Queues"=w9) -> ("error out"=w27:errorcluster)  [unwired: 4 in]
  n242 = call "FVIR_VESTA_Main.vi"("error in"=w11, "VISA resource name"="VESTA FVIR COM", "Message Queues"=w9) -> ("error out"=w24:errorcluster)  [unwired: 8 in]
  n243 = call "FVIR_LDO_Agilent_34972A.vi"("error in"=w11, "VISA Refnum in"="Agilent 34972A", "Message Queues"=w9) -> ("error out"=w19:errorcluster)  [unwired: 8 in]
  n244 = call "LDO_EnviraCom_Main.vi"("Vesta is working"=w4, "Loop Count"=w5, "State"=w6, "error in"=w11, "Retry Count"=w7, "VISA resource name"="EnviraCom LDO COM", "Message Queues"=w9) -> ("error out"=w10:errorcluster)  [unwired: 4 in]
  n245 = while {
    tunnel: w44 -> [w637]
    tunnel: w65 -> [w641]
    shift-right: [w635] -> _
    shift-left: w70 -> [w636]
    tunnel: w46 -> [w640]
    tunnel: [w634] -> w75
    tunnel: w63 -> [w616]
    tunnel: w64 -> [w631]
    tunnel: w34 -> [w630]
    tunnel: w58 -> [w629]
    tunnel: w55 -> [w628]
    shift-right: [w627] -> _
    shift-left: w56 -> [w626]
    tunnel: w54 -> [w625]
    tunnel: w48 -> [w624]
    shift-right: [w622] -> _
    shift-left: w47 -> [w623]
    shift-right: [w619] -> _
    shift-left: string[] [] -> [w621]
    tunnel: w38 -> [w618]
    tunnel: w35 -> [w617]
    tunnel: w26 -> [w614]
    tunnel: w23 -> [w613]
    stop <- w642 stop-if-true
    # "UI Message Loop"
    n246 = call "Dequeue Message.vi"("error in (no error)"=w640, "Message Queue"=w637) -> ("error out"=w639:errorcluster, "Message Data"=w638:variant, "Message"=w620:string, "dup Message Queue"=w632:refnum<queue>)  [unwired: 6 in]
    n247 = case "Message Cases" shown="\"Manual_Heating_Value_UI\"" w620 {
      selector: w620 -> [w651 _ _ _ _ _ _ _ _ _ _ _ _ _ _ _ _ _ _ _ _ _ _ _ _ _ _ _ _ _ _ _ _ _ _ _ _ _ _ _ _ _ _ _ _ _ _ _ _ _ _ _ _ _ _ _ _ _ _ _ _ _ _ _ _ _ _ _ _ _ _ _ _ _ _ _ _ _ _ _ _ _ _]
      tunnel: w632 -> [_ w676 _ _ _ _ _ w812 w832 w878 _ _ _ _ w980 w990 w1021 _ _ w1070 w1082 w1094 w1106 w1118 w1130 w1142 w1154 w1162 w1174 w1186 w1197 w1211 w1223 w1243 w1259 w1270 w1282 w1294 w1306 w1318 w1330 w1342 _ w1360 w1370 w1385 _ w1397 w1408 _ w1449 w1472 w1491 _ _ w1515 w1526 w1538 w1550 w1562 w1574 w1586 w1598 w1610 w1618 w1630 w1648 w1660 w1666 w1678 w1693 w1712 w1731 w1750 w1770 w1780 w1792 _ w1818 w1836 _ w1854 w1865]
      tunnel: w639 -> [_ w675 w684 w736 w740 w766 w789 w815 w845 w886 w927 w932 w951 w958 w975 w991 w1022 w1032 w1043 w1071 w1083 w1095 w1107 w1119 w1131 w1143 w1155 w1165 w1177 w1189 w1201 w1213 w1225 w1244 w1260 w1271 w1283 w1295 w1307 w1319 w1331 w1343 w1352 w1363 w1375 w1384 w1392 w1399 w1421 w1435 w1450 w1466 w1492 w1502 w1508 w1516 w1527 w1539 w1551 w1563 w1575 w1587 w1599 w1611 w1621 w1633 w1649 w1661 w1669 w1681 w1695 w1714 w1733 w1752 w1773 w1785 w1797 w1804 w1817 w1833 w1849 w1856 w1878]
      tunnel: [w650 w670 w684 w737 w742 w776 w788 w790 w833 w876 w922 w931 w941 w957 w979 w987 w999 w1033 w1042 w1073 w1085 w1097 w1109 w1121 w1133 w1145 w1157 w1164 w1176 w1188 w1200 w1212 w1224 w1233 w1249 w1273 w1285 w1297 w1309 w1321 w1333 w1345 w1352 w1358 w1371 w1386 w1394 w1398 w1409 w1435 w1461 w1470 w1477 w1495 w1507 w1517 w1529 w1541 w1553 w1565 w1577 w1589 w1601 w1613 w1620 w1632 w1641 w1653 w1672 w1684 w1688 w1708 w1726 w1744 w1768 w1781 w1793 w1803 w1813 w1827 w1851 w1855 w1866] -> w633
      tunnel: [_ _ _ _ _ TRUE _ _ _ _ _ _ _ _ _ _ _ _ _ _ _ _ _ _ _ _ _ _ _ _ _ _ _ _ _ _ _ _ _ _ _ _ _ _ _ _ _ _ _ _ _ _ _ _ _ _ _ _ _ _ _ _ _ _ _ _ _ _ _ _ _ _ _ _ _ _ _ _ _ _ _ _ _] -> w642
      tunnel: w638 -> [_ _ _ w735 w743 w773 _ w814 _ _ w926 w930 w950 _ _ _ _ w1031 _ _ _ _ _ _ _ _ _ _ _ _ _ _ _ _ _ _ _ _ _ _ _ _ _ w1362 w1374 w1378 _ _ _ _ _ _ _ w1501 _ _ _ _ _ _ _ _ _ _ _ _ _ _ _ _ _ _ _ _ w1772 w1784 w1796 w1802 _ _ _ _ _]
      tunnel: w641 -> [_ _ _ _ _ w777 _ _ _ _ _ _ _ _ _ _ _ _ _ _ _ _ _ _ _ _ _ _ _ _ _ _ _ _ _ _ _ _ _ _ _ _ _ _ _ _ _ _ _ _ _ _ _ _ _ _ _ _ _ _ _ _ _ _ _ _ _ _ _ _ _ _ _ _ _ _ _ _ _ _ _ _ _]
      tunnel: w636 -> [w652 w680 w686 w733 w746 w775 w787 w806 w856 w905 w924 w936 w953 w956 w983 w993 w1020 w1027 w1045 w1068 w1080 w1092 w1104 w1116 w1128 w1140 w1152 w1170 w1182 w1194 w1206 w1218 w1230 w1241 w1257 w1269 w1281 w1293 w1305 w1317 w1329 w1341 w1351 w1364 w1376 w1388 w1396 w1405 w1423 w1438 w1463 w1473 w1490 w1498 w1510 w1514 w1524 w1536 w1548 w1560 w1572 w1584 w1596 w1608 w1626 w1638 w1647 w1659 w1667 w1679 w1694 w1713 w1732 w1751 w1774 w1786 w1798 w1807 w1814 w1830 w1853 w1862 w1880]
      tunnel: [w652 w680 w685 w733 w746 w775 w787 w806 w856 w905 w924 w936 w953 w956 w983 w993 w1020 w1027 w1045 w1068 w1080 w1092 w1104 w1116 w1128 w1140 w1152 w1170 w1182 w1194 w1206 w1218 w1230 w1241 w1257 w1269 w1281 w1293 w1305 w1317 w1329 w1341 w1351 w1364 w1376 w1388 w1396 w1405 w1423 w1438 w1463 w1473 w1490 w1498 w1510 w1514 w1524 w1536 w1548 w1560 w1572 w1584 w1596 w1608 w1626 w1638 w1647 w1659 w1667 w1679 w1694 w1713 w1732 w1751 w1774 w1786 w1798 w1807 w1814 w1830 w1853 w1862 w1880] -> w635
      tunnel: w616 -> [_ w666 _ _ _ w771 _ _ _ _ _ _ _ _ w966 w992 w998 _ w1044 w1069 w1081 w1093 w1105 w1117 w1129 w1141 w1153 w1163 w1175 w1187 w1196 w1210 w1222 w1242 w1258 _ _ _ _ _ _ _ _ _ _ _ _ _ _ _ w1448 w1464 w1480 _ w1509 _ w1525 w1537 w1549 w1561 w1573 w1585 w1597 w1609 w1619 w1631 _ _ w1668 w1680 w1687 w1706 w1725 w1745 _ _ _ _ _ _ _ _ _]
      tunnel: w631 -> [_ _ _ _ _ w769 _ _ _ _ _ _ _ _ _ _ _ _ _ _ _ _ _ _ _ _ _ _ _ _ _ _ _ _ _ _ _ _ _ _ _ _ _ _ _ _ _ _ _ _ _ _ _ _ _ _ _ _ _ _ _ _ _ _ _ _ _ _ _ _ _ _ _ _ _ _ _ _ w1811 w1831 _ _ _]
      tunnel: w630 -> [_ _ _ _ _ w767 _ _ _ _ _ _ _ _ w978 _ _ _ _ _ _ _ _ _ _ _ _ _ _ _ _ _ _ _ _ _ _ _ _ _ _ _ _ _ _ _ w1389 _ _ _ w1460 _ _ _ _ _ _ _ _ _ _ _ _ _ _ _ _ _ _ _ _ _ _ _ _ _ _ _ _ _ w1846 _ _]
      tunnel: w629 -> [_ _ _ _ _ w764 _ _ _ _ _ _ _ _ _ _ _ _ _ _ _ _ _ _ _ _ _ _ _ _ _ _ _ _ _ w1267 w1278 w1290 w1302 w1314 w1326 w1338 _ _ _ _ _ _ _ _ _ _ _ _ _ _ _ _ _ _ _ _ _ _ _ _ _ _ _ _ _ _ _ _ _ _ _ _ _ _ _ _ _]
      tunnel: w628 -> [_ w665 _ _ _ w763 _ _ _ _ _ _ _ _ w964 _ _ _ _ _ _ _ _ _ _ _ _ _ _ _ _ _ _ _ _ _ _ _ _ _ _ _ _ _ _ _ _ _ _ _ _ _ _ _ _ _ _ _ _ _ _ _ _ _ _ _ _ _ _ _ _ _ _ _ _ _ _ _ _ _ _ _ _]
      tunnel: w626 -> [w649 w672 w683 w730 w739 w762 w786 w798 w827 w885 w921 w929 w938 w955 w972 w986 w1005 w1026 w1036 w1065 w1077 w1089 w1101 w1113 w1125 w1137 w1149 w1161 w1173 w1184 w1199 w1209 w1220 w1238 w1254 w1266 w1277 w1289 w1301 w1313 w1325 w1337 w1349 w1356 w1369 w1382 w1391 w1402 w1414 w1437 w1457 w1468 w1485 w1497 w1505 w1512 w1521 w1533 w1545 w1557 w1569 w1581 w1593 w1605 w1617 w1629 w1645 w1657 w1665 w1677 w1692 w1711 w1730 w1749 w1766 w1779 w1791 w1801 w1809 w1829 w1848 w1859 w1871]
      tunnel: [w649 w672 w683 w730 w739 w762 w786 w796 w826 w881 w920 w928 w938 w955 w972 w986 w1005 w1026 w1036 w1065 w1077 w1089 w1101 w1113 w1125 w1137 w1149 w1161 w1173 w1184 w1199 w1209 w1220 w1238 w1254 w1266 w1277 w1289 w1301 w1313 w1325 w1337 w1348 w1355 w1368 w1381 w1391 w1403 w1413 w1437 w1457 w1468 w1485 w1497 w1505 w1512 w1521 w1533 w1545 w1557 w1569 w1581 w1593 w1605 w1617 w1629 w1645 w1657 w1665 w1677 w1692 w1711 w1730 w1749 w1765 w1778 w1790 w1800 w1809 w1829 w1848 w1860 w1870] -> w627
      tunnel: w625 -> [_ _ _ _ _ w760 _ _ _ _ _ _ w937 _ _ _ _ _ _ _ _ _ _ _ _ _ _ _ _ _ _ _ _ _ _ _ _ _ _ _ _ _ _ _ _ _ _ _ _ _ _ _ _ _ _ _ _ _ _ _ _ _ _ _ _ _ _ _ _ _ _ _ _ _ _ _ _ _ _ _ _ _ _]
      tunnel: w624 -> [_ _ _ _ _ w758 _ _ _ _ _ _ _ _ _ _ _ _ _ _ _ _ _ _ _ _ _ _ _ _ _ _ _ _ _ _ _ _ _ _ _ _ _ _ _ _ _ _ _ _ _ _ _ _ _ _ _ _ _ _ _ _ _ _ _ _ _ _ _ _ _ _ _ _ _ _ _ _ _ _ _ _ _]
      tunnel: w623 -> [w648 w671 w682 w729 w738 w757 w785 w795 w838 w884 w923 w935 w952 w954 w973 w985 w1004 w1025 w1037 w1064 w1076 w1088 w1100 w1112 w1124 w1136 w1148 w1160 w1172 w1185 w1198 w1208 w1221 w1237 w1253 w1265 w1276 w1288 w1300 w1312 w1324 w1336 w1350 w1353 w1365 w1377 w1393 w1404 w1422 w1436 w1458 w1467 w1484 w1496 w1506 w1511 w1520 w1532 w1544 w1556 w1568 w1580 w1592 w1604 w1616 w1628 w1644 w1656 w1664 w1676 w1691 w1710 w1729 w1748 w1763 w1775 w1788 w1806 w1808 w1828 w1850 w1861 w1879]
      tunnel: [w648 w671 w682 w729 w738 w757 w785 w795 w830 w883 w923 w935 w952 w954 w973 w985 w1004 w1025 w1037 w1064 w1076 w1088 w1100 w1112 w1124 w1136 w1148 w1160 w1172 w1185 w1198 w1208 w1221 w1237 w1253 w1265 w1276 w1288 w1300 w1312 w1324 w1336 w1350 w1353 w1365 w1377 w1393 w1404 w1422 w1436 w1458 w1467 w1484 w1496 w1506 w1511 w1520 w1532 w1544 w1556 w1568 w1580 w1592 w1604 w1616 w1628 w1644 w1656 w1664 w1676 w1691 w1710 w1729 w1748 w1763 w1775 w1788 w1806 w1808 w1828 w1850 w1861 w1879] -> w622
      tunnel: w618 -> [_ _ _ _ _ w754 _ _ _ _ _ _ _ _ _ _ _ _ _ _ _ _ _ _ _ _ _ _ _ _ _ _ _ _ _ _ _ _ _ _ _ _ _ _ _ _ _ _ _ _ w1446 _ _ _ _ _ _ _ _ _ _ _ _ _ _ _ _ _ _ _ _ _ _ _ _ _ _ _ _ _ _ _ _]
      tunnel: w617 -> [_ _ _ _ _ w752 _ _ _ _ _ _ _ _ _ _ _ _ _ _ _ _ _ _ _ _ _ _ _ _ _ _ _ _ _ _ _ _ _ _ _ _ _ _ _ _ _ _ _ _ _ _ _ _ _ _ _ _ _ _ _ _ _ _ _ _ _ _ _ _ _ _ _ _ _ _ _ _ _ _ _ _ _]
      tunnel: w614 -> [_ w660 _ _ _ w747 _ _ _ _ _ _ _ _ w960 _ _ _ _ _ _ _ _ _ _ _ _ _ _ _ _ _ _ w1232 w1248 _ _ _ _ _ _ _ _ _ _ _ _ _ _ _ _ _ _ _ _ _ _ _ _ _ _ _ _ _ _ _ _ _ _ _ _ _ _ _ _ _ _ _ _ _ _ _ _]
      tunnel: w613 -> [_ w661 _ _ _ _ _ _ _ _ _ _ _ _ _ _ _ _ _ _ _ _ _ _ _ _ _ _ _ _ _ _ _ _ _ _ _ _ _ _ _ _ _ _ _ _ _ _ _ _ w1447 _ _ _ _ _ _ _ _ _ _ _ _ _ _ _ w1640 w1652 _ _ _ _ _ _ _ _ _ _ _ _ _ _ _]
      frame Default {
        # "'Default' case only runs if there is a message that isn't defined in any of the other cases.  Output a programming error."
        n248 = xnode "Error Ring"("parameter 0"=w651) -> ("error out"=w650:errorcluster)
      }
      frame "Initialize" {
        # "Reset all values of the HMI"
        # "Initialize - Get configuration settings, then message the UI to initialize, and broadcast the settings to the other message loops."
        n249 = call-poly "Enqueue Message.vi"("error in (no error)"=w675, "Message Data"=u16[] [0, 0, 0, 0, 0, 0, 0, 0] ("Input Registers"), "Message"="DisplayValuesFromPLC", "Message Queue"=w676) -> ("error out"=w674:errorcluster, "dup Message Queue"=w673:refnum<queue>)  [unwired: 6 in]
        n250 = call-poly "Enqueue Message.vi"("error in (no error)"=w674, "Message"="Init UI Refs", "Message Queue"=w673) -> ("error out"=w668:errorcluster, "dup Message Queue"=w664:refnum<queue>)  [unwired: 7 in]
        n251 = call "Support FVIR Setup.vi"("UI"=w664, "Modbus"=w666, "Initialize?"=TRUE, "Alicat_GasMeter"=w665, "Vesta FVIR"=w661, "error in (no error)"=w668) -> ("UI Output"=w662:refnum<queue>, "error out"=w667:errorcluster)  [unwired: 7 in, 1 out]
        n252 = call "LDO_Setup_Parameters.vi"("UI in"=w662, "Modbus"=w666, "Initialize?"=TRUE, "Alicat_GasMeter"=w665, "Vesta LDO"=w660, "error in (no error)"=w667) -> ("error out"=w670:errorcluster)  [unwired: 9 in]
      }
      frame "Init UI Refs" {
        # "Init UI Refs - Store control references for UI controls.  Also enable/disable controls appropriately."
        n253 = disable-structure shown="Enabled" {
          disable-tunnel: w686 -> [w727 w728]
          disable-tunnel: [w726 w728] -> w685
          frame Disabled {
            n254 = control-ref of="Start - SRI Log"() -> (w723:refnum<vi>)
            n255 = control-ref of="Stop- SRI Log"() -> (w707:refnum<vi>)
            n256 = control-ref of="Start Test Case FVIR"() -> (w708:refnum<vi>)
            n257 = control-ref of="Stop Test Case FVIR"() -> (w720:refnum<vi>)
            n258 = control-ref of="Water Outlet Valve Open FVIR"() -> (w719:refnum<vi>)
            n259 = control-ref of="Water Outlet Valve Close FVIR"() -> (w718:refnum<vi>)
            n260 = control-ref of="Water Inlet Valve Open FVIR"() -> (w717:refnum<vi>)
            n261 = control-ref of="Water Inlet Valve Close FVIR"() -> (w716:refnum<vi>)
            n262 = control-ref of="Gas Solenoid Valve Open FVIR"() -> (w709:refnum<vi>)
            n263 = control-ref of="Gas Solenoid Valve Close FVIR"() -> (w710:refnum<vi>)
            n264 = control-ref of="Spill can - Go to Home Pos"() -> (w711:refnum<vi>)
            n265 = control-ref of="Spill can - Go to Work Pos"() -> (w712:refnum<vi>)
            n266 = control-ref of="Move mannequin - Go to Home Pos"() -> (w713:refnum<vi>)
            n267 = control-ref of="Move mannequin - Go to Work Pos"() -> (w714:refnum<vi>)
            n268 = control-ref of="Send parameters to PLC FVIR"() -> (w706:refnum<vi>)
            n269 = control-ref of="Start Test Case LDO"() -> (w705:refnum<vi>)
            n270 = control-ref of="Stop Test Case LDO"() -> (w704:refnum<vi>)
            n271 = control-ref of="Water Outlet Valve Open LDO"() -> (w703:refnum<vi>)
            n272 = control-ref of="Water Outlet Valve Close LDO"() -> (w702:refnum<vi>)
            n273 = control-ref of="Water Inlet Valve Open LDO"() -> (w701:refnum<vi>)
            n274 = control-ref of="Water Inlet Valve Close LDO"() -> (w700:refnum<vi>)
            n275 = control-ref of="Gas Solenoid Valve Open LDO"() -> (w699:refnum<vi>)
            n276 = control-ref of="Gas Solenoid Valve Close LDO"() -> (w698:refnum<vi>)
            n277 = control-ref of="Start Intellifaucet DRK375 - LDO"() -> (w697:refnum<vi>)
            n278 = control-ref of="Stop Intellifaucet DRK375 - LDO"() -> (w696:refnum<vi>)
            n279 = control-ref of="Oil Spray 0.8 cc/min Open"() -> (w695:refnum<vi>)
            n280 = control-ref of="Oil Spray 0.8 cc/min Close"() -> (w694:refnum<vi>)
            n281 = control-ref of="Oil Spray 1.1 cc/min Open"() -> (w693:refnum<vi>)
            n282 = control-ref of="Oil Spray 1.1 cc/min Close"() -> (w692:refnum<vi>)
            n283 = control-ref of="Oil Spray 1.33 cc/min Open"() -> (w691:refnum<vi>)
            n284 = control-ref of="Oil Spray 1.33 cc/min Close"() -> (w690:refnum<vi>)
            n285 = control-ref of="Rotary Actuator ON"() -> (w689:refnum<vi>)
            n286 = control-ref of="Rotary Actuator OFF"() -> (w688:refnum<vi>)
            n287 = control-ref of="Select test case"() -> (w715:refnum<vi>)
            n288 = control-ref of="FVIR Status"() -> (w687:refnum<vi>)
            n289 = Build Array(w723) -> (w721:refnum<vi>[])
            n290 = Build Array(w688, w689, w690, w691, w692, w693, w694, w695, w696, w697, w698, w699, w700, w701, w702, w703, w704, w705, w706, w715, w714, w713, w712, w711, w710, w709, w716, w717, w718, w719, w720, w708, w707) -> (w722:refnum<vi>[])
            n291 = call "Set Enable State on Multiple Controls.vi"("Enable?"=TRUE, "Controls"=w721) -> ()  [unwired: 10 in]
            n292 = call "Set Enable State on Multiple Controls.vi"("Enable?"=FALSE, "Controls"=w722) -> ()  [unwired: 10 in]
            n293 = Bundle By Name(cluster=w727, "Start Ref"=w723, "Stop Ref"=w707, "Status Ref"=w687, "Start test case FVIR Ref"=w708, "Stop test case FVIR Ref"=w720, "Water Outlet Valve Open FVIR Ref"=w719, "Water Outlet Valve Close FVIR Ref"=w718, "Water Inlet Valve Open FVIR Ref"=w717, "Water Inlet Valve Close FVIR Ref"=w716, "Gas Solenoid Valve Open FVIR Ref"=w709, "Gas Solenoid Valve Close FVIR Ref"=w710, "Spill can Home pos Ref"=w711, "Spill can Work pos Ref"=w712, "Move Mannequin Home pos Ref"=w713, "Move Mannequin Work pos Ref"=w714, "Listbox Ref"=w715, "Send Param to PLC FVIR Ref"=w706, "Start test case LDO Ref"=w705, "Stop test case LDO Ref"=w704, "Water Outlet Valve Open LDO Ref"=w703, "Water Outlet Valve Close LDO Ref"=w702, "Water Inlet Valve Open LDO Ref"=w701, "Water Inlet Valve Close LDO Ref"=w700, "Gas Solenoid Valve Open LDO Ref"=w699, "Gas Solenoid Valve Close LDO Ref"=w698, "Water Flow Open LDO Ref"=w697, "Water Flow Close LDO Ref"=w696, "Oil spray 0.8cc/min Open Ref"=w695, "Oil spray 0.8cc/min Close Ref"=w694, "Oil spray 1.1cc/min Open Ref"=w693, "Oil spray 1.1cc/min Close Ref"=w692, "Oil spray 1.33cc/min Open Ref"=w691, "Oil spray 1.33cc/min Close Ref"=w690, "Heater ON Ref"=w689, "Heater OFF Ref"=w688) -> (w726:T22)
          }
          frame Enabled {
          }
        }
        n294 = property on="Stop Test Case LDO" class="Bool"("DisabledEnum"=T23."Enabled" ("Disabled")) -> ()  [unwired: 2 in, 2 out]
      }
      frame "ShowLabViewLifeBit" {
        # "Update Status - Convert the message data to a string to display in the Status indicator."
        n295 = Variant To Data(error in=w736, type=TRUE, Variant=w735) -> (data=→"Labview lifebit":bool, error out=w734:errorcluster)
        n296 = Merge Errors(w734) -> (w737:errorcluster)
      }
      frame "Error" {
        # "Error - Display an error dialog. This message is sent by the \"Error Handler\" VIs at the end of other loops in this application."
        n297 = Variant To Data(error in=w740, type=errorcluster {"status"=FALSE, "code"=0, "source"=""} ("error constant"), Variant=w743) -> (data=w741:errorcluster, error out=w744:errorcluster)
        n298 = call <vilib>:"Simple Error Handler.vi"("error in (no error)"=w741) -> ()  [unwired: 4 in, 5 out]
        n299 = Merge Errors(w744) -> (w742:errorcluster)
      }
      frame "Exit" {
        w749 = TRUE ("Priority Message? (F)")
        w748 = "Exit" ("Message")
        # "Popup an error dialog if 'Exit' was called as a result of an error."
        # "Stop the VI"
        # "Exit - Send Exit messages to the Acquisition and Logging loops, and fire the user event to stop the Event Handling Loop."
        n300 = Variant To Data(type=errorcluster {"status"=FALSE, "code"=0, "source"=""} ("error constant"), Variant=w773) -> (data=w772:errorcluster)  [unwired: 1 in, 1 out]
        n301 = call <vilib>:"Simple Error Handler.vi"("error in (no error)"=w772) -> ()  [unwired: 4 in, 5 out]
        n302 = call-poly "Enqueue Message.vi"("Priority Message? (F)"=w749, "error in (no error)"=w766, "Message"=w748, "Message Queue"=w771) -> ("error out"=w770:errorcluster)  [unwired: 6 in, 1 out]
        n303 = call-poly "Enqueue Message.vi"("Priority Message? (F)"=w749, "error in (no error)"=w770, "Message"=w748, "Message Queue"=w769) -> ("error out"=w768:errorcluster)  [unwired: 6 in, 1 out]
        n304 = call-poly "Enqueue Message.vi"("Priority Message? (F)"=w749, "error in (no error)"=w768, "Message"=w748, "Message Queue"=w767) -> ("error out"=w765:errorcluster)  [unwired: 6 in, 1 out]
        n305 = call-poly "Enqueue Message.vi"("Priority Message? (F)"=w749, "error in (no error)"=w765, "Message"=w748, "Message Queue"=w764) -> ("error out"=w756:errorcluster)  [unwired: 6 in, 1 out]
        n306 = call-poly "Enqueue Message.vi"("Priority Message? (F)"=w749, "error in (no error)"=w756, "Message"=w748, "Message Queue"=w754) -> ("error out"=w755:errorcluster)  [unwired: 6 in, 1 out]
        n307 = disable-structure shown="Enabled" {
          disable-tunnel: w763 -> [w783 _]
          disable-tunnel: [w782 w784] -> w761
          disable-tunnel: w755 -> [w781 w784]
          disable-tunnel: w749 -> [w780 _]
          disable-tunnel: w748 -> [w779 _]
          frame Disabled {
            n308 = call-poly "Enqueue Message.vi"("Priority Message? (F)"=w780, "error in (no error)"=w781, "Message"=w779, "Message Queue"=w783) -> ("error out"=w782:errorcluster)  [unwired: 6 in, 1 out]
          }
          frame Enabled {
          }
        }
        n309 = call-poly "Enqueue Message.vi"("Priority Message? (F)"=w749, "error in (no error)"=w761, "Message"=w748, "Message Queue"=w760) -> ("error out"=w759:errorcluster)  [unwired: 6 in, 1 out]
        n310 = call-poly "Enqueue Message.vi"("Priority Message? (F)"=w749, "error in (no error)"=w759, "Message"=w748, "Message Queue"=w758) -> ("error out"=w753:errorcluster)  [unwired: 6 in, 1 out]
        n311 = call-poly "Enqueue Message.vi"("Priority Message? (F)"=w749, "error in (no error)"=w753, "Message"=w748, "Message Queue"=w752) -> ("error out"=w751:errorcluster)  [unwired: 6 in, 1 out]
        n312 = call-poly "Enqueue Message.vi"("Priority Message? (F)"=w749, "error in (no error)"=w751, "Message"=w748, "Message Queue"=w747) -> ("error out"=w750:errorcluster)  [unwired: 6 in, 1 out]
        n313 = call "Fire User Event - Stop.vi"("error in (no error)"=w750, "User Event - Stop"=w777) -> ("error out"=w776:errorcluster)  [unwired: 9 in]
      }
      frame "---Display and Processing---" {
        # "Duplicate this frame when creating new messages.  Change this comment in the duplicated frame to describe this message."
        n314 = Merge Errors(w789) -> (w788:errorcluster)
      }
      frame "DisplayValuesFromPLC" {
        # "Update Status - Convert the message data to a string to display in the Status indicator."
        n315 = Unbundle By Name(w798) -> ("PLC Data"=w794:T8)
        n316 = Variant To Data(error in=w815, type=u16[] [1, 0, 0, 0, 0, 0, 0, 0] ("Input Registers"), Variant=w814) -> (data=w810:u16[], error out=w809:errorcluster)
        n317 = call "DisplayValuesFromPLC.vi"("error in"=w809, "PLC Data"=w794, "Input Registers"=w810) -> ("error out"=w808:errorcluster, "PLC Data Out"=w807:T8)  [unwired: 7 in]
        n318 = call "DisplayValuesFromPLC_LDO.vi"("error in"=w808, "PLC Data"=w807) -> ("error out"=w803:errorcluster, "PLC Data Out"=w805:T8)  [unwired: 8 in]
        n319 = call "FVIR Button Disable.vi"("UI Refs"=w806, "error in (no error)"=w803, "PLC Data In"=w805, "Queue in"=w812) -> ("error out"=w802:errorcluster, "PLC Data Out"=w804:T8, "Queue out"=w811:refnum<queue>)  [unwired: 5 in]
        n320 = call "LDO Button Disable.vi"("UI Refs"=w806, "error in (no error)"=w802, "PLC Data In"=w804, "Queue in"=w811) -> ("error out"=w799:errorcluster, "PLC Data Out"=w797:T8, "dup Message Queue"=w800:refnum<queue>)  [unwired: 5 in]
        n321 = call-poly "Enqueue Message.vi"("error in (no error)"=w799, "Message"="DisplayAllData_LDO", "Message Queue"=w800) -> ("error out"=w792:errorcluster, "dup Message Queue"=w791:refnum<queue>)  [unwired: 7 in]
        n322 = Bundle By Name(cluster=w798, "PLC Data"=w797) -> (w796:T7)
        n323 = call-poly "Enqueue Message.vi"("error in (no error)"=w792, "Message"="DisplayAllData_FVIR", "Message Queue"=w791) -> ("error out"=w790:errorcluster)  [unwired: 7 in, 1 out]
      }
      frame "DisplayAllData_LDO" {
        n324 = Unbundle By Name(w827) -> ("PLC Data"=w828:T8)
        n325 = Unbundle By Name(w828) -> ("PLC Data - LDO.Start recording data - LDO"=→"Start recording data - LDO":bool, "PLC Data - LDO.Water Outlet Valve - LDO"=→"Water Outlet Valve":bool, "PLC Data - LDO.Water Inlet Valve - LDO"=→"Water Inlet Valve":bool, "PLC Data - LDO.Gas Solenoid Valve - LDO"=→"Gas Solenoid Valve":bool, "PLC Data - LDO.Water flow DRK375 is open - LDO"=→"Intellifaucet Start_LDO":bool, "PLC Data - LDO.Oil spray 0.8cc/min - LDO"=→"Oil spray 0.8cc/min":bool, "PLC Data - LDO.Oil spray 1.1cc/min - LDO"=→"Oil spray 1.1cc/min":bool, "PLC Data - LDO.Oil spray 1.33cc/min - LDO"=→"Oil spray 1.33cc/min":bool, "PLC Data - LDO.Rotary Actuator (ON/OFF) - LDO"=→"Rotary Actuator (ON/OFF)":bool, "PLC Data - LDO.Water Outlet Flow Proportional - LDO"=→"Water Outlet Flow Proportional":bool, "PLC Data - LDO.Status for error - LDO"=→"Status for error - LDO":string, "PLC Data - LDO.Error - LDO"=→"Error - LDO":bool, "PLC Data - LDO.Test chamber is in sequence - LDO"=→"Test chamber is in sequence":bool, "PLC Data - LDO.Conveyor ON/OFF"=→"Conveyor":bool, "PLC Data - LDO.Blower ON/OFF"=→"Blower":bool)
        n326 = control-ref of="Oil spray 1.1cc/min"() -> (w835:refnum<vi>)
        n327 = control-ref of="Oil spray 0.8cc/min"() -> (w836:refnum<vi>)
        n328 = control-ref of="Rotary Actuator (ON/OFF)"() -> (w818:refnum<vi>)
        n329 = control-ref of="Burner-LDO"() -> (w837:refnum<vi>)
        n330 = control-ref of="Oil spray 1.33cc/min"() -> (w822:refnum<vi>)
        n331 = control-ref of="Start recording data - LDO"() -> (w821:refnum<vi>)
        n332 = call "LDO Array Data.vi"("All Data"=w827, "1.33 ML Ref"=w822, "Start recording data"=w821, "error in (no error)"=w845, "Burner ON Ref"=w837, "Event Booleans in"=w838, "Rotary Actuator (ON/OFF)"=w818, "0.8 ML Ref"=w836, "Pilot Rate (BTU/hr)"="Pilot Rate (BTU/hr)-LDO", "1.1 ML Ref"=w835) -> ("Event Booleans out"=w830:T6, "PLC Data output"=w826:T7, "error out"=w834:errorcluster)  [unwired: 7 in]
        n333 = Unbundle By Name(w826) -> ("PLC Data.PLC Data - LDO.Test chamber is in sequence - LDO"=w819:bool, "PLC Data.Terminate Conditions - LDO.Stop Test"=w820:bool, "PLC Data.Data to Save - ALL.LDO Full Data"=→"LDO Data":string[][], "PLC Data.PLC Data - LDO.Test chamber is in sequence - LDO"=w824:bool, "PLC Data.PLC Data - LDO.Start recording data - LDO"=w823:bool)
        n334 = And(x=w819, y=w820) -> (x .and. y?=→"LDO Auto Stop Condition Met?":bool)
        n335 = And(x=w824, y=w823) -> (x .and. y?=w831:bool)
        n336 = Unbundle By Name(w830) -> ("Burner ON - LDO"=→"Burner-LDO":bool)
        n337 = case shown="False" "stop ldo test" {
          tunnel: w834 -> [w860 w866]
          tunnel: [w859 w867] -> w833
          tunnel: w832 -> [w858 w868]
          tunnel: w831 -> [w857 _]
          frame False {
            n338 = case shown="True" w857 {
              tunnel: w860 -> [w861 w864]
              tunnel: [w861 w863] -> w859
              tunnel: w858 -> [_ w862]
              frame False {
              }
              frame True {
                n339 = call-poly "Enqueue Message.vi"("error in (no error)"=w864, "Message"="LDOUpdateFlowTarget", "Message Queue"=w862) -> ("error out"=w863:errorcluster)  [unwired: 7 in, 1 out]
              }
            }
          }
          frame True {
            n340 = call-poly "Enqueue Message.vi"("error in (no error)"=w866, "Message"="StopTestCaseLDO", "Message Queue"=w868) -> ("error out"=w867:errorcluster)  [unwired: 7 in, 1 out]
          }
        }
      }
      frame "DisplayAllData_FVIR" {
        n341 = Unbundle By Name(w885) -> ("PLC Data"=w888:T8)
        n342 = Unbundle By Name(w888) -> ("PLC Data - FVIR.FVIR PLC lifebit"=→"FVIR PLC lifebit":bool, "PLC Data - FVIR.Mannequin is moving - FVIR"=→"Mannequin is moving - FVIR":bool, "PLC Data - FVIR.Can is spilling - FVIR"=→"Can is spilling - FVIR":bool, "PLC Data - FVIR.Water Outlet Valve - FVIR"=→"Water Outlet Valve - FVIR":bool, "PLC Data - FVIR.Water Inlet Valve - FVIR"=→"Water Inlet Valve - FVIR":bool, "PLC Data - FVIR.Gas Solenoid Valve - FVIR"=→"Gas Solenoid Valve - FVIR":bool, "PLC Data - FVIR.Water flow DRK375 is open - FVIR"=→"Intellifaucet Start - FVIR":bool, "PLC Data - FVIR.Actuator mannequin is going to Home Pos - FVIR"=→"Actuator mannequin is going to Home Pos - FVIR":bool, "PLC Data - FVIR.Actuator mannequin is going to Work Pos - FVIR"=→"Actuator mannequin is going to Work Pos - FVIR":bool, "PLC Data - FVIR.Actuator spill can is going to Home Pos - FVIR"=→"Actuator spill can is going to Home Pos - FVIR":bool, "PLC Data - FVIR.Actuator spill can is going to Work Pos - FVIR"=→"Actuator spill can is going to Work Pos - FVIR":bool, "PLC Data - FVIR.Start recording data - FVIR"=→"Start recording data - FVIR":bool, "PLC Data - FVIR.Status for Error - FVIR"=→"Status for error - FVIR":string, "PLC Data - FVIR.Error-FVIR"=→"Error - FVIR":bool, "PLC Data - FVIR.Water Outlet Flow Proportional - FVIR"=→"Water Outlet Flow Proportional - FVIR":bool, "PLC Data - FVIR.Test chamber is in sequence - FVIR"=→"Test chamber is in sequence - FVIR":bool)
        n343 = control-ref of="Start recording data - FVIR"() -> (w880:refnum<vi>)
        n344 = control-ref of="Burner-FVIR"() -> (w879:refnum<vi>)
        n345 = call "FVIR Array Data.vi"("All Data"=w885, "error in (no error)"=w886, "Burner ON Ref"=w879, "Event Booleans in"=w884, "Start recording data"=w880, "Pilot Rate (BTU/hr)"="Pilot Rate (BTU/hr)-FVIR") -> ("Event Booleans out"=w883:T6, "All Data output"=w881:T7, "Higher than 0.9% butane"=→"Higher than 0.9% butane":bool, "error out"=w877:errorcluster)  [unwired: 10 in]
        n346 = Unbundle By Name(w883) -> ("Burner ON - FVIR"=→"Burner-FVIR":bool)
        n347 = Unbundle By Name(w881) -> ("PLC Data.Data to Save - ALL.FVIR Full Data"=→"FVIR Data":string[][], "PLC Data.PLC Data - FVIR.Test chamber is in sequence - FVIR"=w874:bool, "PLC Data.PLC Data - FVIR.Start recording data - FVIR"=w875:bool)
        n348 = And(x=w874, y=w875) -> (x .and. y?=w873:bool)
        n349 = case shown="False" "stop FVIR test" {
          tunnel: w877 -> [w909 w915]
          tunnel: [w908 w916] -> w876
          tunnel: w878 -> [w907 w917]
          tunnel: w873 -> [w906 _]
          frame False {
            n350 = case shown="True" w906 {
              tunnel: w909 -> [w910 w913]
              tunnel: [w910 w912] -> w908
              tunnel: w907 -> [_ w911]
              frame False {
              }
              frame True {
                n351 = call-poly "Enqueue Message.vi"("error in (no error)"=w913, "Message"="FVIRUpdateFlowTarget", "Message Queue"=w911) -> ("error out"=w912:errorcluster)  [unwired: 7 in, 1 out]
              }
            }
          }
          frame True {
            n352 = call-poly "Enqueue Message.vi"("error in (no error)"=w915, "Message"="StopTestCaseFVIR", "Message Queue"=w917) -> ("error out"=w916:errorcluster)  [unwired: 7 in, 1 out]
          }
        }
      }
      frame "DataToShow_FVIR" {
        # "Update Status - Convert the message data to a string to display in the Status indicator."
        n353 = Variant To Data(error in=w927, type=string[][] [], Variant=w926) -> (data=w919:string[][], error out=w922:errorcluster)
        n354 = Bundle By Name(cluster=w921, "PLC Data.Terminate Conditions - FVIR.SRI Butane Values"=w919) -> (w920:T7)
      }
      frame "DisplayValuesFromInficon" {
        w933 = T15 {"Gross Heating Value, Vol (Real, Dry)"=0.0, "Nitrogen Component Normalized Mole % (Dry)"=0.0, "Methane Component Normalized Mole % (Dry)"=0.0, "Carbon Dioxide Component Normalized Mole % (Dry)"=0.0, "Ethane Component Normalized Mole % (Dry)"=0.0, "Propane Component Normalized Mole % (Dry)"=0.0, "i-Pentane Component Normalized Mole % (Dry)"=0.0, "i-Butane Component Normalized Mole % (Dry)"=0.0, "n-Butane Component Normalized Mole % (Dry)"=0.0, "n-Pentane Component Normalized Mole % (Dry)"=0.0, "Hexane Component Normalized Mole % (Dry)"=0.0, "Heptane Component Normalized Mole % (Dry)"=0.0, "Gross Wobbe Index, Real(Dry)"=0.0, "Relative Density, Real(Dry)"=0.0, "Propylene Component Normalized Mole % (Dry)"=0.0, "C4 Olefins Component Normalized Mole % (Dry)"=0.0, "Water Component Normalized Mole % (Dry)"=0.0}  # Inficon Data Input
        # "Collect data from the inficon loop."
        n355 = Variant To Data(error in=w932, type=w933, Variant=w930) -> (data=w934:T15, error out=w931:errorcluster)
        n356 = Bundle By Name(cluster=w929, "Inficon Data - ALL"=w934) -> (w928:T7)
      }
      frame "Manual_Heating_Value_UI" {
        # "Collect data from the inficon loop."
        n357 = Variant To Data(error in=w951, type=TRUE, Variant=w950) -> (data=w939:bool, error out=w942:errorcluster)
        n358 = call-poly "Enqueue Message.vi"("Priority Message? (F)"=TRUE, "error in (no error)"=w942, "Message Data"=w939, "Message"="Manual_Heating_Value_NG", "Message Queue"=w937) -> ("error out"=w946:errorcluster, "dup Message Queue"=w947:refnum<queue>)  [unwired: 5 in]
        n359 = call-poly "Enqueue Message.vi"("Priority Message? (F)"=TRUE, "error in (no error)"=w946, "Message Data"="HHV-NG-Manual", "Message"="Heating_Value_Adjust_NG", "Message Queue"=w947) -> ("error out"=w941:errorcluster)  [unwired: 5 in, 1 out]
      }
      frame "---LDO Test---" {
        # "Duplicate this frame when creating new messages.  Change this comment in the duplicated frame to describe this message."
        n360 = Merge Errors(w958) -> (w957:errorcluster)
      }
      frame "StartTestCaseLDO" {
        # "Reset the total flow and gas total\nSend latest timing parameters"
        # "Indicate that now a LDO test is active"
        # "Start - Enable/Disable buttons appropriately for an acquisition that has started, and update status display."
        n361 = local read "Vesta ON Temperature LDO"() -> (w959:T3)
        n362 = call-poly "Enqueue Message.vi"("error in (no error)"=w975, "Message Data"="LDO test has started..." ("Acquiring and Logging..."), "Message"="Update Status - LDO", "Message Queue"=w980) -> ("error out"=w968:errorcluster, "dup Message Queue"=w965:refnum<queue>)  [unwired: 6 in]
        n363 = call "LDO_Setup_Parameters.vi"("UI in"=w965, "Modbus"=w966, "Initialize?"=FALSE, "Alicat_GasMeter"=w964, "Vesta LDO"=w960, "Vesta ON Temperature (LDO)"=w959, "error in (no error)"=w968) -> ("error out"=w967:errorcluster)  [unwired: 8 in]
        n364 = call-poly "Enqueue Message.vi"("Priority Message? (F)"=TRUE, "error in (no error)"=w967, "Message"="StartTestCaseLDO", "Message Queue"=w966) -> ("error out"=w974:errorcluster)  [unwired: 6 in, 1 out]
        n365 = Bundle By Name(cluster=w972, "PLC Data.Data to Save - ALL.Test Case - LDO"="LDO_test" ("Acquiring and Logging..."), "PLC Data.Terminate Conditions - LDO"=T14 {"Condition B - Array"=[], "Current Cycle"=0, "Condition C - Array"=[], "Condition A - Array"=[], "400 PPM Disable Counter"=FALSE, "Condition A - Norm"=[], "Condition B - Norm"=[], "Condition C - Norm"=[], "Condition A"=FALSE, "Condition B"=FALSE, "Condition C"=FALSE, "Condition A - Cont Cycle"=[], "Stop Test"=FALSE} ("PLC Data Out.Terminate Conditions")) -> (w970:T7)
        n366 = Unbundle By Name(w970) -> ("PLC Data"=w969:T8)
        n367 = call-poly "Enqueue Message.vi"("error in (no error)"=w974, "Message Data"=w969, "Message"="InsertTextIntoDataFileNameLDO", "Message Queue"=w978) -> ("error out"=w979:errorcluster)  [unwired: 6 in, 1 out]
      }
      frame "StopTestCaseLDO" {
        # "Start - Enable/Disable buttons appropriately for an acquisition that has started, and update status display."
        n368 = call "StopLDOTest.vi"("error in (no error)"=w991, "Queue in"=w992) -> ("error out"=w984:errorcluster)  [unwired: 9 in]
        n369 = call-poly "Enqueue Message.vi"("error in (no error)"=w984, "Message Data"="Current LDO test has stopped ..." ("Acquiring and Logging..."), "Message"="Update Status - LDO", "Message Queue"=w990) -> ("error out"=w987:errorcluster)  [unwired: 6 in, 1 out]
      }
      frame "SendParamToPLCLDO" {
        # "Start - Enable/Disable buttons appropriately for an acquisition that has started, and update status display."
        n370 = call-poly "Enqueue Message.vi"("error in (no error)"=w1022, "Message Data"="Operator clicked on: Send parameters to PLC LDO ..." ("Acquiring and Logging..."), "Message"="Update Status - LDO", "Message Queue"=w1021) -> ("error out"=w1001:errorcluster)  [unwired: 6 in, 1 out]
        n371 = Build Array("Burner cycle 1 to 10 - Duty cycle ON (default 55 min.)", "Burner cycle 1 to 10 - Duty cycle OFF (default 5 min.)", "Burner cycle 11 to 12 - Duty cycle ON (default 235 min.)", "Burner cycle 11 to 12 - Duty cycle OFF (default 5 min.)", "Burner cycle 13 to end - Duty cycle ON (default 55 min.)", "Burner cycle 13 to end - Duty cycle OFF (default 5 min.)", "Oil 1st sequence ON (default 5 min.)", "Oil 1st sequence OFF (default 5 min.)", "All subsequent sequence ON (default 3 min.)", "All subsequent sequence OFF (default 27 min.)", "Oil spray preconditioning period ON (default 10 min.)", "Oil spray preconditioning period OFF  (default 20 min.)", "Precondition Purge Gallons") -> (w1019:u16[])
        n372 = call "LDO_Update_Intellifaucet_Parameters.vi"("FVIR?"=FALSE, "error in (no error)"=w1001, "Valve % Open - Automatic Mode"="Valve % Open - Automatic Mode (LDO)", "Temp (°F) - Automatic Mode"="Temp (°F) - Automatic Mode (LDO)", "Modbus Input"=w998) -> ("error out"=w1000:errorcluster, "dup Message Queue"=w997:refnum<queue>)  [unwired: 5 in]
        n373 = call-poly "Enqueue Message.vi"("Priority Message? (F)"=FALSE, "error in (no error)"=w1000, "Message Data"=w1019, "Message"="SendParamToPLCLDO", "Message Queue"=w997) -> ("error out"=w999:errorcluster)  [unwired: 5 in, 1 out]
      }
      frame "Update status - LDO" {
        # "Update Status - Convert the message data to a string to display in the Status indicator."
        n374 = Variant To Data(error in=w1032, type="", Variant=w1031) -> (data=→"LDO Status":string, error out=w1029:errorcluster)
        n375 = Merge Errors(w1029) -> (w1033:errorcluster)
      }
      frame "LDOUpdateFlowTarget" {
        n376 = Unbundle By Name(w1036) -> ("PLC Data.PLC Data - LDO.Total Cycle Counter"=w1035:u16)
        n377 = Unbundle By Name(w1036) -> ("PLC Data.PLC Data - LDO.Thermal Efficiency Rate (GPM)"=w1041:dbl, "PLC Data.PLC Data - LDO.Totalized Flow (Gallons)"=w1040:dbl)
        n378 = call "FVIR_LDO_LongCycleCheck.vi"("Total Cycle Counter"=w1035) -> ("Short Cycle?"=w1034:bool)  [unwired: 10 in]
        n379 = Greater?(x=w1040, y="Start Auto GPM Gallons-LDO") -> (0:w1038:bool)
        n380 = case shown="True" w1038 {
          tunnel: w1044 -> [w1047 w1057]
          tunnel: w1043 -> [w1049 w1055]
          tunnel: [w1048 w1056] -> w1042
          tunnel: w1041 -> [_ w1053]
          tunnel: w1034 -> [_ w1050]
          frame False {
            n381 = call "Update_Flow_Target.vi"("error in"=w1049, "Output Flow Rate Target (Automated Test)"=0.76, "Modbus"=w1047) -> ("error out"=w1048:errorcluster)  [unwired: 8 in]
          }
          frame True {
            n382 = case shown="True" "LDO-Manual Flow Control?" {
              tunnel: w1053 -> [w1058 _]
              tunnel: [w1058 w1060] -> w1052
              tunnel: w1050 -> [_ w1059]
              frame False {
              }
              frame True {
                n383 = case shown="False" w1059 {
                  tunnel: ["Long Draw Flow Rate (GPM)" "Short Draw Flow Rate (GPM)"] -> w1060
                  frame False {
                  }
                  frame True {
                  }
                }
              }
            }
            n384 = call "Update_Flow_Target.vi"("FVIR?"=FALSE, "error in"=w1055, "Output Flow Rate Target (Automated Test)"=w1052, "Modbus"=w1057) -> ("error out"=w1056:errorcluster)  [unwired: 7 in]
          }
        }
      }
      frame "WaterOutletOpenLDO" {
        # "Start - Enable/Disable buttons appropriately for an acquisition that has started, and update status display."
        n385 = call-poly "Enqueue Message.vi"("error in (no error)"=w1071, "Message Data"="Operator clicked on: Water Outlet Valve Open LDO" ("Acquiring and Logging..."), "Message"="Update Status - LDO", "Message Queue"=w1070) -> ("error out"=w1072:errorcluster)  [unwired: 6 in, 1 out]
        n386 = call-poly "Enqueue Message.vi"("Priority Message? (F)"=TRUE, "error in (no error)"=w1072, "Message"="WaterOutletOpenLDO", "Message Queue"=w1069) -> ("error out"=w1073:errorcluster)  [unwired: 6 in, 1 out]
      }
      frame "WaterOutletCloseLDO" {
        # "Start - Enable/Disable buttons appropriately for an acquisition that has started, and update status display."
        n387 = call-poly "Enqueue Message.vi"("error in (no error)"=w1083, "Message Data"="Operator clicked on: Water Outlet Valve Close LDO" ("Acquiring and Logging..."), "Message"="Update Status - LDO", "Message Queue"=w1082) -> ("error out"=w1084:errorcluster)  [unwired: 6 in, 1 out]
        n388 = call-poly "Enqueue Message.vi"("Priority Message? (F)"=TRUE, "error in (no error)"=w1084, "Message"="WaterOutletCloseLDO", "Message Queue"=w1081) -> ("error out"=w1085:errorcluster)  [unwired: 6 in, 1 out]
      }
      frame "WaterInletOpenLDO" {
        # "Start - Enable/Disable buttons appropriately for an acquisition that has started, and update status display."
        n389 = call-poly "Enqueue Message.vi"("error in (no error)"=w1095, "Message Data"="Operator clicked on: Water Inlet Valve Open LDO" ("Acquiring and Logging..."), "Message"="Update Status - LDO", "Message Queue"=w1094) -> ("error out"=w1096:errorcluster)  [unwired: 6 in, 1 out]
        n390 = call-poly "Enqueue Message.vi"("Priority Message? (F)"=TRUE, "error in (no error)"=w1096, "Message"="WaterInletOpenLDO", "Message Queue"=w1093) -> ("error out"=w1097:errorcluster)  [unwired: 6 in, 1 out]
      }
      frame "WaterInletCloseLDO" {
        # "Start - Enable/Disable buttons appropriately for an acquisition that has started, and update status display."
        n391 = call-poly "Enqueue Message.vi"("error in (no error)"=w1107, "Message Data"="Operator clicked on: Water Inlet Valve Close LDO" ("Acquiring and Logging..."), "Message"="Update Status - LDO", "Message Queue"=w1106) -> ("error out"=w1108:errorcluster)  [unwired: 6 in, 1 out]
        n392 = call-poly "Enqueue Message.vi"("Priority Message? (F)"=TRUE, "error in (no error)"=w1108, "Message"="WaterInletCloseLDO", "Message Queue"=w1105) -> ("error out"=w1109:errorcluster)  [unwired: 6 in, 1 out]
      }
      frame "GasSolenoidOpenLDO" {
        # "Start - Enable/Disable buttons appropriately for an acquisition that has started, and update status display."
        n393 = call-poly "Enqueue Message.vi"("error in (no error)"=w1119, "Message Data"="Operator clicked on: Gas Solenoid Valve Open LDO" ("Acquiring and Logging..."), "Message"="Update Status - LDO", "Message Queue"=w1118) -> ("error out"=w1120:errorcluster)  [unwired: 6 in, 1 out]
        n394 = call-poly "Enqueue Message.vi"("Priority Message? (F)"=TRUE, "error in (no error)"=w1120, "Message"="GasSolenoidOpenLDO", "Message Queue"=w1117) -> ("error out"=w1121:errorcluster)  [unwired: 6 in, 1 out]
      }
      frame "GasSolenoidCloseLDO" {
        # "Start - Enable/Disable buttons appropriately for an acquisition that has started, and update status display."
        n395 = call-poly "Enqueue Message.vi"("error in (no error)"=w1131, "Message Data"="Operator clicked on: Gas Solenoid Valve Close LDO" ("Acquiring and Logging..."), "Message"="Update Status - LDO", "Message Queue"=w1130) -> ("error out"=w1132:errorcluster)  [unwired: 6 in, 1 out]
        n396 = call-poly "Enqueue Message.vi"("Priority Message? (F)"=TRUE, "error in (no error)"=w1132, "Message"="GasSolenoidCloseLDO", "Message Queue"=w1129) -> ("error out"=w1133:errorcluster)  [unwired: 6 in, 1 out]
      }
      frame "WaterFlowStartLDO" {
        # "Start - Enable/Disable buttons appropriately for an acquisition that has started, and update status display."
        n397 = call-poly "Enqueue Message.vi"("error in (no error)"=w1143, "Message Data"="Operator clicked on: Water Flow Intellifaucet DRK375 Start" ("Acquiring and Logging..."), "Message"="Update Status - LDO", "Message Queue"=w1142) -> ("error out"=w1144:errorcluster)  [unwired: 6 in, 1 out]
        n398 = call-poly "Enqueue Message.vi"("Priority Message? (F)"=TRUE, "error in (no error)"=w1144, "Message"="WaterFlowStartLDO", "Message Queue"=w1141) -> ("error out"=w1145:errorcluster)  [unwired: 6 in, 1 out]
      }
      frame "WaterFlowStartZeroLDO" {
        # "Start - Enable/Disable buttons appropriately for an acquisition that has started, and update status display."
        n399 = call-poly "Enqueue Message.vi"("error in (no error)"=w1155, "Message Data"="Operator clicked on: Water Flow Intellifaucet DRK375 Start" ("Acquiring and Logging..."), "Message"="Update Status - LDO", "Message Queue"=w1154) -> ("error out"=w1156:errorcluster)  [unwired: 6 in, 1 out]
        n400 = call-poly "Enqueue Message.vi"("Priority Message? (F)"=TRUE, "error in (no error)"=w1156, "Message"="WaterFlowStartZeroLDO", "Message Queue"=w1153) -> ("error out"=w1157:errorcluster)  [unwired: 6 in, 1 out]
      }
      frame "WaterFlowStopLDO" {
        n401 = call-poly "Enqueue Message.vi"("error in (no error)"=w1165, "Message Data"="Operator clicked on: Water Flow Intellifaucet DRK375 Stop" ("Acquiring and Logging..."), "Message"="Update Status - LDO", "Message Queue"=w1162) -> ("error out"=w1169:errorcluster)  [unwired: 6 in, 1 out]
        n402 = call-poly "Enqueue Message.vi"("Priority Message? (F)"=TRUE, "error in (no error)"=w1169, "Message"="WaterFlowStopLDO", "Message Queue"=w1163) -> ("error out"=w1164:errorcluster)  [unwired: 6 in, 1 out]
      }
      frame "WaterFlowStopZeroLDO" {
        n403 = call-poly "Enqueue Message.vi"("error in (no error)"=w1177, "Message Data"="Operator clicked on: Water Flow Intellifaucet DRK375 Stop" ("Acquiring and Logging..."), "Message"="Update Status - LDO", "Message Queue"=w1174) -> ("error out"=w1181:errorcluster)  [unwired: 6 in, 1 out]
        n404 = call-poly "Enqueue Message.vi"("Priority Message? (F)"=TRUE, "error in (no error)"=w1181, "Message"="WaterFlowStopZeroLDO", "Message Queue"=w1175) -> ("error out"=w1176:errorcluster)  [unwired: 6 in, 1 out]
      }
      frame "ConveyorON" {
        n405 = call-poly "Enqueue Message.vi"("error in (no error)"=w1189, "Message Data"="Operator clicked on: Conveyor ON..." ("Acquiring and Logging..."), "Message"="Update Status - LDO", "Message Queue"=w1186) -> ("error out"=w1193:errorcluster)  [unwired: 6 in, 1 out]
        n406 = call-poly "Enqueue Message.vi"("Priority Message? (F)"=TRUE, "error in (no error)"=w1193, "Message"="ConveyorON", "Message Queue"=w1187) -> ("error out"=w1188:errorcluster)  [unwired: 6 in, 1 out]
      }
      frame "ConveyorOFF" {
        n407 = call-poly "Enqueue Message.vi"("error in (no error)"=w1201, "Message Data"="Operator clicked on: Conveyor OFF..." ("Acquiring and Logging..."), "Message"="Update Status - LDO", "Message Queue"=w1197) -> ("error out"=w1205:errorcluster)  [unwired: 6 in, 1 out]
        n408 = call-poly "Enqueue Message.vi"("Priority Message? (F)"=TRUE, "error in (no error)"=w1205, "Message"="ConveyorOFF", "Message Queue"=w1196) -> ("error out"=w1200:errorcluster)  [unwired: 6 in, 1 out]
      }
      frame "BlowerON" {
        n409 = call-poly "Enqueue Message.vi"("error in (no error)"=w1213, "Message Data"="Operator clicked on: Blower ON..." ("Acquiring and Logging..."), "Message"="Update Status - LDO", "Message Queue"=w1211) -> ("error out"=w1217:errorcluster)  [unwired: 6 in, 1 out]
        n410 = call-poly "Enqueue Message.vi"("Priority Message? (F)"=TRUE, "error in (no error)"=w1217, "Message"="BlowerON", "Message Queue"=w1210) -> ("error out"=w1212:errorcluster)  [unwired: 6 in, 1 out]
      }
      frame "BlowerOFF" {
        n411 = call-poly "Enqueue Message.vi"("error in (no error)"=w1225, "Message Data"="Operator clicked on: Conveyor OFF..." ("Acquiring and Logging..."), "Message"="Update Status - LDO", "Message Queue"=w1223) -> ("error out"=w1229:errorcluster)  [unwired: 6 in, 1 out]
        n412 = call-poly "Enqueue Message.vi"("Priority Message? (F)"=TRUE, "error in (no error)"=w1229, "Message"="BlowerOFF", "Message Queue"=w1222) -> ("error out"=w1224:errorcluster)  [unwired: 6 in, 1 out]
      }
      frame "HeaterON_LDO" {
        # "Start - Enable/Disable buttons appropriately for an acquisition that has started, and update status display."
        n413 = call-poly "Enqueue Message.vi"("error in (no error)"=w1244, "Message Data"="Operator clicked on: Heater ON..." ("Acquiring and Logging..."), "Message"="Update Status - LDO", "Message Queue"=w1243) -> ("error out"=w1245:errorcluster)  [unwired: 6 in, 1 out]
        n414 = call-poly "Enqueue Message.vi"("Priority Message? (F)"=TRUE, "error in (no error)"=w1245, "Message"="HeaterON_LDO", "Message Queue"=w1242) -> ("error out"=w1234:errorcluster)  [unwired: 6 in, 1 out]
        n415 = local read "Vesta ON Temperature LDO"() -> (w1231:T3)
        n416 = call-poly "Enqueue Message.vi"("error in (no error)"=w1234, "Message Data"=w1231, "Message"="PUT_Vesta_Temp_LDO", "Message Queue"=w1232) -> ("error out"=w1233:errorcluster)  [unwired: 6 in, 1 out]
      }
      frame "HeaterOFF_LDO" {
        # "Turn the heater off"
        # "Start - Enable/Disable buttons appropriately for an acquisition that has started, and update status display."
        n417 = call-poly "Enqueue Message.vi"("error in (no error)"=w1260, "Message Data"="Operator clicked on: Heater OFF..." ("Acquiring and Logging..."), "Message"="Update Status - LDO", "Message Queue"=w1259) -> ("error out"=w1261:errorcluster)  [unwired: 6 in, 1 out]
        n418 = call-poly "Enqueue Message.vi"("Priority Message? (F)"=TRUE, "error in (no error)"=w1261, "Message"="HeaterOFF_LDO", "Message Queue"=w1258) -> ("error out"=w1250:errorcluster)  [unwired: 6 in, 1 out]
        n419 = local read "Vesta OFF Temperature LDO"() -> (w1247:T3)
        n420 = call-poly "Enqueue Message.vi"("error in (no error)"=w1250, "Message Data"=w1247, "Message"="PUT_Vesta_Temp_LDO", "Message Queue"=w1248) -> ("error out"=w1249:errorcluster)  [unwired: 6 in, 1 out]
      }
      frame "OilSpray08Open" {
        # "Open the 0.80 oil spray valve."
        # "Start - Enable/Disable buttons appropriately for an acquisition that has started, and update status display."
        n421 = call-poly "Enqueue Message.vi"("error in (no error)"=w1271, "Message Data"="Operator clicked on: Oil Spray 0.8 cc/min Open" ("Acquiring and Logging..."), "Message"="Update Status - LDO", "Message Queue"=w1270) -> ("error out"=w1272:errorcluster)  [unwired: 6 in, 1 out]
        n422 = call-poly "Enqueue Message.vi"("Priority Message? (F)"=TRUE, "error in (no error)"=w1272, "Message"="OilSpray08Open", "Message Queue"=w1267) -> ("error out"=w1273:errorcluster)  [unwired: 6 in, 1 out]
      }
      frame "OilSpray08Close" {
        # "Close the 0.80 oil spray valve."
        # "Start - Enable/Disable buttons appropriately for an acquisition that has started, and update status display."
        n423 = call-poly "Enqueue Message.vi"("error in (no error)"=w1283, "Message Data"="Operator clicked on: Oil Spray 0.8 cc/min Close" ("Acquiring and Logging..."), "Message"="Update Status - LDO", "Message Queue"=w1282) -> ("error out"=w1284:errorcluster)  [unwired: 6 in, 1 out]
        n424 = call-poly "Enqueue Message.vi"("Priority Message? (F)"=TRUE, "error in (no error)"=w1284, "Message"="OilSpray08Close", "Message Queue"=w1278) -> ("error out"=w1285:errorcluster)  [unwired: 6 in, 1 out]
      }
      frame "OilSpray11Open" {
        # "Open the 1.11 oil spray valve."
        # "Start - Enable/Disable buttons appropriately for an acquisition that has started, and update status display."
        n425 = call-poly "Enqueue Message.vi"("error in (no error)"=w1295, "Message Data"="Operator clicked on: Oil Spray 1.1 cc/min Open" ("Acquiring and Logging..."), "Message"="Update Status - LDO", "Message Queue"=w1294) -> ("error out"=w1296:errorcluster)  [unwired: 6 in, 1 out]
        n426 = call-poly "Enqueue Message.vi"("Priority Message? (F)"=TRUE, "error in (no error)"=w1296, "Message"="OilSpray11Open", "Message Queue"=w1290) -> ("error out"=w1297:errorcluster)  [unwired: 6 in, 1 out]
      }
      frame "OilSpray11Close" {
        # "Close the 1.11 oil spray valve."
        # "Start - Enable/Disable buttons appropriately for an acquisition that has started, and update status display."
        n427 = call-poly "Enqueue Message.vi"("error in (no error)"=w1307, "Message Data"="Operator clicked on: Oil Spray 1.1 cc/min Close" ("Acquiring and Logging..."), "Message"="Update Status - LDO", "Message Queue"=w1306) -> ("error out"=w1308:errorcluster)  [unwired: 6 in, 1 out]
        n428 = call-poly "Enqueue Message.vi"("Priority Message? (F)"=TRUE, "error in (no error)"=w1308, "Message"="OilSpray11Close", "Message Queue"=w1302) -> ("error out"=w1309:errorcluster)  [unwired: 6 in, 1 out]
      }
      frame "OilSpray133Open" {
        # "Open the 1.33 oil spray valve."
        # "Start - Enable/Disable buttons appropriately for an acquisition that has started, and update status display."
        n429 = call-poly "Enqueue Message.vi"("error in (no error)"=w1319, "Message Data"="Operator clicked on: Oil Spray 1.33 cc/min Open" ("Acquiring and Logging..."), "Message"="Update Status - LDO", "Message Queue"=w1318) -> ("error out"=w1320:errorcluster)  [unwired: 6 in, 1 out]
        n430 = call-poly "Enqueue Message.vi"("Priority Message? (F)"=TRUE, "error in (no error)"=w1320, "Message"="OilSpray133Open", "Message Queue"=w1314) -> ("error out"=w1321:errorcluster)  [unwired: 6 in, 1 out]
      }
      frame "OilSpray133Close" {
        # "Close the 1.33 oil spray valve."
        # "Start - Enable/Disable buttons appropriately for an acquisition that has started, and update status display."
        n431 = call-poly "Enqueue Message.vi"("error in (no error)"=w1331, "Message Data"="Operator clicked on: Oil Spray 1.33 cc/min Close" ("Acquiring and Logging..."), "Message"="Update Status - LDO", "Message Queue"=w1330) -> ("error out"=w1332:errorcluster)  [unwired: 6 in, 1 out]
        n432 = call-poly "Enqueue Message.vi"("Priority Message? (F)"=TRUE, "error in (no error)"=w1332, "Message"="OilSpray133Close", "Message Queue"=w1326) -> ("error out"=w1333:errorcluster)  [unwired: 6 in, 1 out]
      }
      frame "Oil_Alarm" {
        # "There is an alarm on the oil machine. I can only\nseem to clear the error by sending a serial command.\nNot sure....but its here"
        # "Start - Enable/Disable buttons appropriately for an acquisition that has started, and update status display."
        n433 = call-poly "Enqueue Message.vi"("error in (no error)"=w1343, "Message Data"="Operator clicked on: Oil Spray Alarm" ("Acquiring and Logging..."), "Message"="Update Status - LDO", "Message Queue"=w1342) -> ("error out"=w1344:errorcluster)  [unwired: 6 in, 1 out]
        n434 = call-poly "Enqueue Message.vi"("Priority Message? (F)"=TRUE, "error in (no error)"=w1344, "Message"="Oil_Alarm", "Message Queue"=w1338) -> ("error out"=w1345:errorcluster)  [unwired: 6 in, 1 out]
      }
      frame "ResetLDOTimer" {
        # "i have timers that will reset the elapsed time during the preconditioning and start of test."
        n435 = Bundle By Name(cluster=w1349, "PLC Data.PLC Data - LDO.Timing"=T10 {"First Call Time Ref"=0.0, "Precondition Time Ref"=0.0, "Test Time Ref"=0.0, "Get First Call Time"=FALSE, "Get Precondition Time"=FALSE, "Get Test Time"=FALSE, "Display Time"=0.0, "Real-Time Clock"={"fractional second"=0.0, "second"=0, "minute"=0, "hour"=0, "day of month"=0, "month"=0, "year"=0, "day of week"=0, "day of year"=0, "DST"=0}, "Absolute Time"=0.0} ("PLC Data Out.LDO Control Input.Timing")) -> (w1348:T7)
      }
      frame "DisplayValuesFromAlicat_LDO" {
        # "Display the values from the gas meter LDO loop"
        n436 = Variant To Data(error in=w1363, type=T16 {"Data Cluster"={"Absolute Pressure"=0.0, "Gauge/Diff. Pressure"=0.0, "Barometric Pressure"=0.0, "Temperature"=0.0, "Volumetric Flow"=0.0, "Mass Flow"=0.0, "Setpoint"=0.0, "Valve Drive"=0.0, "Totalizer"=0.0, "[hr]"=0.0, "[min]"=0.0, "[sec]"=0.0, "Totalizer Average Flow"=0.0, "Totalizer Peak Flow"=0.0, "Gas selected"=""}, "Units of Measure Input"={"Abs. Pressure"="", "Gauge/Diff. Press."="", "Barometric Press."="", "Temperature"="", "Volume"="", "Mass"="", "Setpoint"="", "Valve Drive"="", "Totalizer"="", "Tot. Timer"="", "Tot. Avg. Flow"="", "Tot. Peak Flow"=""}, "Header Array"=[]} ("Gas Data"), Variant=w1362) -> (data=w1354:T16, error out=w1359:errorcluster)
        n437 = Bundle By Name(cluster=w1356, "Gas Data.Gas Data - LDO"=w1354) -> (w1355:T7)
        n438 = call-poly "Enqueue Message.vi"("error in (no error)"=w1359, "Message"="DisplayAllData_LDO", "Message Queue"=w1360) -> ("error out"=w1358:errorcluster)  [unwired: 7 in, 1 out]
      }
      frame "DisplayValuesFromUltramat_LDO" {
        # "Display the values from the Ultramat LDO loop"
        n439 = Variant To Data(error in=w1375, type=string[][] [], Variant=w1374) -> (data=w1366:string[][], error out=w1372:errorcluster)
        n440 = Bundle By Name(cluster=w1369, "Ultramat 23.Ultramat 23 - LDO"=w1366) -> (w1368:T7)
        n441 = call-poly "Enqueue Message.vi"("error in (no error)"=w1372, "Message"="DisplayAllData_LDO", "Message Queue"=w1370) -> ("error out"=w1371:errorcluster)  [unwired: 7 in, 1 out]
      }
      frame "DisplayValuesFromVestaLDO" {
        # "Display the values from the Vesta LDO Loop"
        n442 = Variant To Data(error in=w1384, type=T20 {"Temp_W_Raw_U"=0, "Temp_W_Raw_L"=0, "Temperature Water (F)"=0.0, "Temperature Water Compensated (F)"=0.0, "Temperature Ambient (F)"=0.0, "Setpoint Location (F)"=0.0, "Heat Request"="", "Fault Ram"="", "PWM DCDC Value"=0, "Pilot Voltage (mV)"=0.0, "Setpoint Actual (F)"=0.0, "Differential Actual (F)"=0.0, "Setpoint User (F)"=0.0, "Differential User (F)"=0.0, "Termperature FIltered -TCO (F)"=0.0, "Temp_C_Raw_1 - Sensor Voltage"="", "Temp_C_Raw_2 - Sensor Voltage"="", "Chamber Sensor Temperature (F)"=0.0, "LDO Base Temperature (F)"=0.0, "LDO Timer (sec)"=0, "Disabled (0)"=FALSE, "Warming (1)"=FALSE, "Heating (2)"=FALSE, "Cooling Data Write (3)"=FALSE, "Cooling (4)"=FALSE, "Data Read (5)"=FALSE, "N/A"=FALSE, "Temperature Trip (7)"=FALSE, "Burner"=FALSE} ("Vesta Data.Vesta LDO"), Variant=w1378) -> (data=w1379:T20, error out=w1383:errorcluster)
        n443 = Bundle By Name(cluster=w1382, "Vesta Data.Vesta LDO"=w1379) -> (w1381:T7)
        n444 = call-poly "Enqueue Message.vi"("error in (no error)"=w1383, "Message"="DisplayAllData_LDO", "Message Queue"=w1385) -> ("error out"=w1386:errorcluster)  [unwired: 7 in, 1 out]
      }
      frame "CheckBeforeWriteDataLDO" {
        # "Send the latest information to the \ndata save loop"
        n445 = Unbundle By Name(w1391) -> ("PLC Data"=w1390:T8)
        n446 = call-poly "Enqueue Message.vi"("error in (no error)"=w1392, "Message Data"=w1390, "Message"="CheckBeforeWriteDataLDO", "Message Queue"=w1389) -> ("error out"=w1394:errorcluster)  [unwired: 6 in, 1 out]
      }
      frame "Start ANSI LDO" {
        n447 = Unbundle By Name(w1402) -> ("PLC Data.PLC Data - LDO.Timing.Absolute Time"=w1401:dbl)
        n448 = Bundle By Name(cluster=w1402, "ANSI Rates.ANSI Rate LDO.ANSI Start Time"=w1401) -> (w1403:T7)
        n449 = call-poly "Enqueue Message.vi"("error in (no error)"=w1399, "Message"="ANSI Rate LDO", "Message Queue"=w1397) -> ("error out"=w1398:errorcluster)  [unwired: 7 in, 1 out]
      }
      frame "ANSI Rate LDO" {
        n450 = Unbundle By Name(w1414) -> ("ANSI Rates.ANSI Rate LDO"=w1411:T19, "Ultramat 23.Ultramat 23 - LDO"=w1415:string[][], "Gas Data.Gas Data - LDO.Data Cluster"=w1416:T17, "Inficon Data - ALL"=w1417:T15, "PLC Data.PLC Data - LDO.Timing.Absolute Time"=w1407:dbl)
        n451 = call "HEWH ANSI Get Rates.vi"("ANSI Rate in"=w1411, "Test Type - Rate"="Test Type - Rate", "CO CO2 Data Array"=w1415, "Gas Measurment Data"=w1416, "Inficon Data - ALL"=w1417, "error in (no error)"=w1421, "Software Elapsed Time"=w1407) -> ("ANSI Display 1"=→"ANSI Display LDO":string, "ANSI Rate out"=w1412:T19, "Rate Outputs"=→"LDO Rate Info":string[][], "Test Complete"=w1406:bool, "error out"=w1410:errorcluster)  [unwired: 4 in]
        n452 = Bundle By Name(cluster=w1414, "ANSI Rates.ANSI Rate LDO"=w1412) -> (w1413:T7)
        n453 = case shown="True" w1406 {
          tunnel: w1410 -> [w1427 w1433]
          tunnel: [w1426 w1433] -> w1409
          tunnel: w1408 -> [w1425 _]
          frame False {
            n454 = property on="Start ANSI LDO" class="Bool (strict)"() -> ("Value"=w1424:bool)  [unwired: 2 in, 2 out]
            n455 = case shown="True" w1424 {
              tunnel: w1427 -> [w1428 w1431]
              tunnel: [w1428 w1430] -> w1426
              tunnel: w1425 -> [_ w1429]
              frame False {
              }
              frame True {
                n456 = call-poly "Enqueue Message.vi"("error in (no error)"=w1431, "Message"="ANSI Rate LDO", "Message Queue"=w1429) -> ("error out"=w1430:errorcluster)  [unwired: 7 in, 1 out]
              }
            }
          }
          frame True {
            n457 = property on="Start ANSI LDO" class="Bool (strict)"("Value"=FALSE ("Start ANSI LDO")) -> ()  [unwired: 2 in, 2 out]
          }
        }
      }
      frame "---FVIR Test---" {
        # "Duplicate this frame when creating new messages.  Change this comment in the duplicated frame to describe this message."
      }
      frame "StartTestCaseFVIR" {
        # "Indicate that now a FVIR test is active"
        # "Start - Enable/Disable buttons appropriately for an acquisition that has started, and update status display."
        n458 = local read "Time Delay of Change direction of Mannequin Actuators (mS)"() -> (w1444:u16)
        n459 = local read "Time Pause Between Next Mannequin Sequence"() -> (w1442:u16)
        n460 = local read "Number of Mannequin Movement"() -> (w1443:u16)
        n461 = local read "Vesta ON Temperature FVIR"() -> (w1445:T3)
        n462 = Subtract(x=w1442, y=u16 3) -> (x-y=w1440:u16)
        n463 = Build Array(w1444, w1443, w1440) -> (w1439:u16[])
        n464 = call "Support FVIR Setup.vi"("UI"=w1449, "Modbus"=w1448, "Initialize?"=FALSE, "Alicat_GasMeter"=w1446, "Vesta FVIR"=w1447, "Vesta ON Temperature (FVIR)"=w1445, "Select test case"="Select test case", "error in (no error)"=w1450, "Mannequin Data"=w1439) -> ("Test Case - FVIR"=w1453:string, "error out"=w1451:errorcluster)  [unwired: 4 in, 1 out]
        n465 = Bundle By Name(cluster=w1457, "PLC Data.Data to Save - ALL.Test Case - FVIR"=w1453, "PLC Data.PLC Data - FVIR.Timing"=T10 {"First Call Time Ref"=0.0, "Precondition Time Ref"=0.0, "Test Time Ref"=0.0, "Get First Call Time"=FALSE, "Get Precondition Time"=FALSE, "Get Test Time"=FALSE, "Display Time"=0.0, "Real-Time Clock"={"fractional second"=0.0, "second"=0, "minute"=0, "hour"=0, "day of month"=0, "month"=0, "year"=0, "day of week"=0, "day of year"=0, "DST"=0}, "Absolute Time"=0.0}) -> (w1456:T7)
        n466 = Unbundle By Name(w1456) -> ("PLC Data"=w1455:T8)
        n467 = call-poly "Enqueue Message.vi"("error in (no error)"=w1451, "Message Data"=w1455, "Message"="InsertTextIntoDataFileNameFVIR", "Message Queue"=w1460) -> ("error out"=w1461:errorcluster)  [unwired: 6 in, 1 out]
      }
      frame "StopTestCaseFVIR" {
        # "Move the actuators back to the home \nposition and turn off flow."
        # "Start - Enable/Disable buttons appropriately for an acquisition that has started, and update status display."
        n468 = call "Modbus_Stop_FVIR_Test.vi"("error in (no error)"=w1466, "Queue in"=w1464) -> ("error out"=w1465:errorcluster)  [unwired: 9 in]
        n469 = call-poly "Enqueue Message.vi"("error in (no error)"=w1465, "Message Data"="Current FVIR test has stopped ..." ("Acquiring and Logging..."), "Message"="Update Status - FVIR", "Message Queue"=w1472) -> ("error out"=w1470:errorcluster)  [unwired: 6 in, 1 out]
      }
      frame "SendParamToPLCFVIR" {
        # "Start - Enable/Disable buttons appropriately for an acquisition that has started, and update status display."
        n470 = call-poly "Enqueue Message.vi"("error in (no error)"=w1492, "Message Data"="Operator clicked on: Send parameters to PLC FVIR ..." ("Acquiring and Logging..."), "Message"="Update Status - FVIR", "Message Queue"=w1491) -> ("error out"=w1481:errorcluster)  [unwired: 6 in, 1 out]
        n471 = Build Array("Time Delay of Change direction of Mannequin Actuators (mS)", "Number of Mannequin Movement", "Time Pause Between Next Mannequin Sequence") -> (w1487:u16[])
        n472 = call "LDO_Update_Intellifaucet_Parameters.vi"("FVIR?"=TRUE, "error in (no error)"=w1481, "Valve % Open - Automatic Mode"="Valve % Open - Automatic Mode (FVIR)", "Temp (°F) - Automatic Mode"="Temp (°F) - Automatic Mode (FVIR)", "Modbus Input"=w1480) -> ("error out"=w1479:errorcluster, "dup Message Queue"=w1478:refnum<queue>)  [unwired: 5 in]
        n473 = call-poly "Enqueue Message.vi"("Priority Message? (F)"=FALSE, "error in (no error)"=w1479, "Message Data"=w1487, "Message"="SendParamToPLCFVIR", "Message Queue"=w1478) -> ("error out"=w1477:errorcluster)  [unwired: 5 in, 1 out]
      }
      frame "Update status - FVIR" {
        # "Update Status - Convert the message data to a string to display in the Status indicator."
        n474 = Variant To Data(error in=w1502, type="", Variant=w1501) -> (data=→"FVIR Status":string, error out=w1495:errorcluster)
      }
      frame "FVIRUpdateFlowTarget" {
        n475 = call "Update_Flow_Target.vi"("FVIR?"=TRUE, "error in"=w1508, "Output Flow Rate Target (Automated Test)"="FVIR-Flow Rate (GPM)", "Modbus"=w1509) -> ("error out"=w1507:errorcluster)  [unwired: 7 in]
      }
      frame "SRI8610C_Not_Active" {
        # "Start - Enable/Disable buttons appropriately for an acquisition that has started, and update status display."
        n476 = call-poly "Enqueue Message.vi"("error in (no error)"=w1516, "Message Data"="SRI8610C Gas Chromatograph has stopped unexpectedly." ("Acquiring and Logging..."), "Message"="Update Status - FVIR", "Message Queue"=w1515) -> ("error out"=w1517:errorcluster)  [unwired: 6 in, 1 out]
      }
      frame "WaterOutletOpenFVIR" {
        # "Open water outlet valve"
        # "Start - Enable/Disable buttons appropriately for an acquisition that has started, and update status display."
        n477 = call-poly "Enqueue Message.vi"("error in (no error)"=w1527, "Message Data"="Operator clicked on: Water Outlet Valve Open FVIR" ("Acquiring and Logging..."), "Message"="Update Status - FVIR", "Message Queue"=w1526) -> ("error out"=w1528:errorcluster)  [unwired: 6 in, 1 out]
        n478 = call-poly "Enqueue Message.vi"("Priority Message? (F)"=TRUE, "error in (no error)"=w1528, "Message"="WaterOutletOpenFVIR", "Message Queue"=w1525) -> ("error out"=w1529:errorcluster)  [unwired: 6 in, 1 out]
      }
      frame "WaterOutletCloseFVIR" {
        # "Close water outlet valve"
        # "Start - Enable/Disable buttons appropriately for an acquisition that has started, and update status display."
        n479 = call-poly "Enqueue Message.vi"("error in (no error)"=w1539, "Message Data"="Operator clicked on: Water Outlet Valve Close FVIR" ("Acquiring and Logging..."), "Message"="Update Status - FVIR", "Message Queue"=w1538) -> ("error out"=w1540:errorcluster)  [unwired: 6 in, 1 out]
        n480 = call-poly "Enqueue Message.vi"("Priority Message? (F)"=TRUE, "error in (no error)"=w1540, "Message"="WaterOutletCloseFVIR", "Message Queue"=w1537) -> ("error out"=w1541:errorcluster)  [unwired: 6 in, 1 out]
      }
      frame "WaterInletOpenFVIR" {
        # "Open water inlet valve"
        # "Start - Enable/Disable buttons appropriately for an acquisition that has started, and update status display."
        n481 = call-poly "Enqueue Message.vi"("error in (no error)"=w1551, "Message Data"="Operator clicked on: Water Inlet Valve Open FVIR" ("Acquiring and Logging..."), "Message"="Update Status - FVIR", "Message Queue"=w1550) -> ("error out"=w1552:errorcluster)  [unwired: 6 in, 1 out]
        n482 = call-poly "Enqueue Message.vi"("Priority Message? (F)"=TRUE, "error in (no error)"=w1552, "Message"="WaterInletOpenFVIR", "Message Queue"=w1549) -> ("error out"=w1553:errorcluster)  [unwired: 6 in, 1 out]
      }
      frame "WaterInletCloseFVIR" {
        # "Close water inlet valve"
        # "Start - Enable/Disable buttons appropriately for an acquisition that has started, and update status display."
        n483 = call-poly "Enqueue Message.vi"("error in (no error)"=w1563, "Message Data"="Operator clicked on: Water Inlet Valve Close FVIR" ("Acquiring and Logging..."), "Message"="Update Status - FVIR", "Message Queue"=w1562) -> ("error out"=w1564:errorcluster)  [unwired: 6 in, 1 out]
        n484 = call-poly "Enqueue Message.vi"("Priority Message? (F)"=TRUE, "error in (no error)"=w1564, "Message"="WaterInletCloseFVIR", "Message Queue"=w1561) -> ("error out"=w1565:errorcluster)  [unwired: 6 in, 1 out]
      }
      frame "GasSolenoidOpenFVIR" {
        # "Open gas valve"
        # "Start - Enable/Disable buttons appropriately for an acquisition that has started, and update status display."
        n485 = call-poly "Enqueue Message.vi"("error in (no error)"=w1575, "Message Data"="Operator clicked on: Gas Solenoid Valve Open FVIR" ("Acquiring and Logging..."), "Message"="Update Status - FVIR", "Message Queue"=w1574) -> ("error out"=w1576:errorcluster)  [unwired: 6 in, 1 out]
        n486 = call-poly "Enqueue Message.vi"("Priority Message? (F)"=TRUE, "error in (no error)"=w1576, "Message"="GasSolenoidOpenFVIR", "Message Queue"=w1573) -> ("error out"=w1577:errorcluster)  [unwired: 6 in, 1 out]
      }
      frame "GasSolenoidCloseFVIR" {
        # "Close gas valve"
        # "Start - Enable/Disable buttons appropriately for an acquisition that has started, and update status display."
        n487 = call-poly "Enqueue Message.vi"("error in (no error)"=w1587, "Message Data"="Operator clicked on: Gas Solenoid Valve Close FVIR" ("Acquiring and Logging..."), "Message"="Update Status - FVIR", "Message Queue"=w1586) -> ("error out"=w1588:errorcluster)  [unwired: 6 in, 1 out]
        n488 = call-poly "Enqueue Message.vi"("Priority Message? (F)"=TRUE, "error in (no error)"=w1588, "Message"="GasSolenoidCloseFVIR", "Message Queue"=w1585) -> ("error out"=w1589:errorcluster)  [unwired: 6 in, 1 out]
      }
      frame "WaterFlowStartFVIR" {
        # "The intellifaucet requires a pulse input. When you\npress start, this is the on portion"
        # "Start - Enable/Disable buttons appropriately for an acquisition that has started, and update status display."
        n489 = call-poly "Enqueue Message.vi"("error in (no error)"=w1599, "Message Data"="Operator clicked on: Water Flow Intellifaucet DRK375 Start" ("Acquiring and Logging..."), "Message"="Update Status - FVIR", "Message Queue"=w1598) -> ("error out"=w1600:errorcluster)  [unwired: 6 in, 1 out]
        n490 = call-poly "Enqueue Message.vi"("Priority Message? (F)"=TRUE, "error in (no error)"=w1600, "Message"="WaterFlowStartFVIR", "Message Queue"=w1597) -> ("error out"=w1601:errorcluster)  [unwired: 6 in, 1 out]
      }
      frame "WaterFlowStartZeroFVIR" {
        # "The intellifaucet requires a pulse input. When you\npress start, this is the off portion"
        # "Start - Enable/Disable buttons appropriately for an acquisition that has started, and update status display."
        n491 = call-poly "Enqueue Message.vi"("error in (no error)"=w1611, "Message Data"="Operator clicked on: Water Flow Intellifaucet DRK375 Start" ("Acquiring and Logging..."), "Message"="Update Status - FVIR", "Message Queue"=w1610) -> ("error out"=w1612:errorcluster)  [unwired: 6 in, 1 out]
        n492 = call-poly "Enqueue Message.vi"("Priority Message? (F)"=TRUE, "error in (no error)"=w1612, "Message"="WaterFlowStartZeroFVIR", "Message Queue"=w1609) -> ("error out"=w1613:errorcluster)  [unwired: 6 in, 1 out]
      }
      frame "WaterFlowStopFVIR" {
        # "The intellifaucet requires a pulse input. When you\npress start, this is the on portion"
        n493 = call-poly "Enqueue Message.vi"("error in (no error)"=w1621, "Message Data"="Operator clicked on: Water Flow Intellifaucet DRK375 Stop" ("Acquiring and Logging..."), "Message"="Update Status - FVIR", "Message Queue"=w1618) -> ("error out"=w1625:errorcluster)  [unwired: 6 in, 1 out]
        n494 = call-poly "Enqueue Message.vi"("Priority Message? (F)"=TRUE, "error in (no error)"=w1625, "Message"="WaterFlowStopFVIR", "Message Queue"=w1619) -> ("error out"=w1620:errorcluster)  [unwired: 6 in, 1 out]
      }
      frame "WaterFlowStopZeroFVIR" {
        # "The intellifaucet requires a pulse input. When you\npress start, this is the off portion"
        n495 = call-poly "Enqueue Message.vi"("error in (no error)"=w1633, "Message Data"="Operator clicked on: Water Flow Intellifaucet DRK375 Stop" ("Acquiring and Logging..."), "Message"="Update Status - FVIR", "Message Queue"=w1630) -> ("error out"=w1637:errorcluster)  [unwired: 6 in, 1 out]
        n496 = call-poly "Enqueue Message.vi"("Priority Message? (F)"=TRUE, "error in (no error)"=w1637, "Message"="WaterFlowStopZeroFVIR", "Message Queue"=w1631) -> ("error out"=w1632:errorcluster)  [unwired: 6 in, 1 out]
      }
      frame "HeaterON_FVIR" {
        # "Start - Enable/Disable buttons appropriately for an acquisition that has started, and update status display."
        n497 = call-poly "Enqueue Message.vi"("error in (no error)"=w1649, "Message Data"="Operator clicked on: Heater ON..." ("Acquiring and Logging..."), "Message"="Update Status - FVIR", "Message Queue"=w1648) -> ("error out"=w1642:errorcluster)  [unwired: 6 in, 1 out]
        n498 = call-poly "Enqueue Message.vi"("error in (no error)"=w1642, "Message Data"="Vesta ON Temperature FVIR", "Message"="PUT_Vesta_Temp_FVIR", "Message Queue"=w1640) -> ("error out"=w1641:errorcluster)  [unwired: 6 in, 1 out]
      }
      frame "HeaterOFF_FVIR" {
        # "Start - Enable/Disable buttons appropriately for an acquisition that has started, and update status display."
        n499 = call-poly "Enqueue Message.vi"("error in (no error)"=w1661, "Message Data"="Operator clicked on: Heater OFF..." ("Acquiring and Logging..."), "Message"="Update Status - FVIR", "Message Queue"=w1660) -> ("error out"=w1654:errorcluster)  [unwired: 6 in, 1 out]
        n500 = call-poly "Enqueue Message.vi"("error in (no error)"=w1654, "Message Data"="Vesta OFF Temperature FVIR", "Message"="PUT_Vesta_Temp_FVIR", "Message Queue"=w1652) -> ("error out"=w1653:errorcluster)  [unwired: 6 in, 1 out]
      }
      frame "StartManSeq" {
        # "Run the full manniquin sequence"
        # "Start - Enable/Disable buttons appropriately for an acquisition that has started, and update status display."
        n501 = call-poly "Enqueue Message.vi"("error in (no error)"=w1669, "Message Data"="Operator clicked on: Start Mannequin Sequence" ("Acquiring and Logging..."), "Message"="Update Status - FVIR", "Message Queue"=w1666) -> ("error out"=w1670:errorcluster)  [unwired: 6 in, 1 out]
        n502 = call-poly "Enqueue Message.vi"("Priority Message? (F)"=TRUE, "error in (no error)"=w1670, "Message"="StartManSeq", "Message Queue"=w1668) -> ("error out"=w1672:errorcluster)  [unwired: 6 in, 1 out]
      }
      frame "StopManSeq" {
        # "Run the full manniquin sequence"
        # "Start - Enable/Disable buttons appropriately for an acquisition that has started, and update status display."
        n503 = call-poly "Enqueue Message.vi"("error in (no error)"=w1681, "Message Data"="Operator clicked on: Stop Mannequin Sequence" ("Acquiring and Logging..."), "Message"="Update Status - FVIR", "Message Queue"=w1678) -> ("error out"=w1682:errorcluster)  [unwired: 6 in, 1 out]
        n504 = call-poly "Enqueue Message.vi"("Priority Message? (F)"=TRUE, "error in (no error)"=w1682, "Message"="StopManSeq", "Message Queue"=w1680) -> ("error out"=w1684:errorcluster)  [unwired: 6 in, 1 out]
      }
      frame "MannequinHomePos" {
        # "Move the mannequin to the idle position"
        # "Start - Enable/Disable buttons appropriately for an acquisition that has started, and update status display."
        n505 = disable-structure shown="Disabled" {
          disable-tunnel: w1694 -> [w1698 _]
          frame Disabled {
            n506 = Unbundle By Name(w1698) -> ("Stop Ref"=w1703:refnum<vi>, "Start Ref"=w1702:refnum<vi>, "Exit Ref"=w1701:refnum<vi>)
            n507 = Build Array(w1703) -> (w1704:refnum<vi>[])
            n508 = Build Array(w1702, w1701) -> (w1705:refnum<vi>[])
            n509 = call "Set Enable State on Multiple Controls.vi"("Enable?"=TRUE, "Controls"=w1704) -> ()  [unwired: 10 in]
            n510 = call "Set Enable State on Multiple Controls.vi"("Enable?"=FALSE, "Controls"=w1705) -> ()  [unwired: 10 in]
          }
          frame Enabled {
          }
        }
        n511 = call-poly "Enqueue Message.vi"("error in (no error)"=w1695, "Message Data"="Operator clicked on: Move mannequin to Home Pos" ("Acquiring and Logging..."), "Message"="Update Status - FVIR", "Message Queue"=w1693) -> ("error out"=w1689:errorcluster)  [unwired: 6 in, 1 out]
        n512 = call "Manniquin Control.vi"("Position"=Mannequin_and_Gas_Position."Mannequin Home", "error in (no error)"=w1689, "Queue in"=w1687) -> ("error out"=w1688:errorcluster)  [unwired: 7 in, 1 out]
      }
      frame "MannequinWorkPos" {
        # "Move the mannequin toward the water heater"
        # "Start - Enable/Disable buttons appropriately for an acquisition that has started, and update status display."
        n513 = disable-structure shown="Disabled" {
          disable-tunnel: w1713 -> [w1717 _]
          frame Disabled {
            n514 = Unbundle By Name(w1717) -> ("Stop Ref"=w1722:refnum<vi>, "Start Ref"=w1721:refnum<vi>, "Exit Ref"=w1720:refnum<vi>)
            n515 = Build Array(w1722) -> (w1723:refnum<vi>[])
            n516 = Build Array(w1721, w1720) -> (w1724:refnum<vi>[])
            n517 = call "Set Enable State on Multiple Controls.vi"("Enable?"=TRUE, "Controls"=w1723) -> ()  [unwired: 10 in]
            n518 = call "Set Enable State on Multiple Controls.vi"("Enable?"=FALSE, "Controls"=w1724) -> ()  [unwired: 10 in]
          }
          frame Enabled {
          }
        }
        n519 = call-poly "Enqueue Message.vi"("error in (no error)"=w1714, "Message Data"="Operator clicked on: Move mannequin to Work Pos" ("Acquiring and Logging..."), "Message"="Update Status - FVIR", "Message Queue"=w1712) -> ("error out"=w1707:errorcluster)  [unwired: 6 in, 1 out]
        n520 = call "Manniquin Control.vi"("Position"=Mannequin_and_Gas_Position."Mannequin Work", "error in (no error)"=w1707, "Queue in"=w1706) -> ("error out"=w1708:errorcluster)  [unwired: 7 in, 1 out]
      }
      frame "SpillCanHomePos" {
        # "Move the spill can acuator back\nto the idle position"
        # "Start - Enable/Disable buttons appropriately for an acquisition that has started, and update status display."
        n521 = disable-structure shown="Disabled" {
          disable-tunnel: w1732 -> [w1736 _]
          frame Disabled {
            n522 = Unbundle By Name(w1736) -> ("Stop Ref"=w1741:refnum<vi>, "Start Ref"=w1740:refnum<vi>, "Exit Ref"=w1739:refnum<vi>)
            n523 = Build Array(w1741) -> (w1742:refnum<vi>[])
            n524 = Build Array(w1740, w1739) -> (w1743:refnum<vi>[])
            n525 = call "Set Enable State on Multiple Controls.vi"("Enable?"=TRUE, "Controls"=w1742) -> ()  [unwired: 10 in]
            n526 = call "Set Enable State on Multiple Controls.vi"("Enable?"=FALSE, "Controls"=w1743) -> ()  [unwired: 10 in]
          }
          frame Enabled {
          }
        }
        n527 = call-poly "Enqueue Message.vi"("error in (no error)"=w1733, "Message Data"="Operator clicked on: Move gasoline can to Home Pos" ("Acquiring and Logging..."), "Message"="Update Status - FVIR", "Message Queue"=w1731) -> ("error out"=w1727:errorcluster)  [unwired: 6 in, 1 out]
        n528 = call "Manniquin Control.vi"("Position"=Mannequin_and_Gas_Position."Gas Can Home", "error in (no error)"=w1727, "Queue in"=w1725) -> ("error out"=w1726:errorcluster)  [unwired: 7 in, 1 out]
      }
      frame "SpillCanWorkPos" {
        # "Spill the can toward the water heater"
        # "Start - Enable/Disable buttons appropriately for an acquisition that has started, and update status display."
        n529 = disable-structure shown="Disabled" {
          disable-tunnel: w1751 -> [w1755 _]
          frame Disabled {
            n530 = Unbundle By Name(w1755) -> ("Stop Ref"=w1760:refnum<vi>, "Start Ref"=w1759:refnum<vi>, "Exit Ref"=w1758:refnum<vi>)
            n531 = Build Array(w1760) -> (w1761:refnum<vi>[])
            n532 = Build Array(w1759, w1758) -> (w1762:refnum<vi>[])
            n533 = call "Set Enable State on Multiple Controls.vi"("Enable?"=TRUE, "Controls"=w1761) -> ()  [unwired: 10 in]
            n534 = call "Set Enable State on Multiple Controls.vi"("Enable?"=FALSE, "Controls"=w1762) -> ()  [unwired: 10 in]
          }
          frame Enabled {
          }
        }
        n535 = call-poly "Enqueue Message.vi"("error in (no error)"=w1752, "Message Data"="Operator clicked on: Move gasoline can to Work Pos" ("Acquiring and Logging..."), "Message"="Update Status - FVIR", "Message Queue"=w1750) -> ("error out"=w1746:errorcluster)  [unwired: 6 in, 1 out]
        n536 = call "Manniquin Control.vi"("Position"=Mannequin_and_Gas_Position."Gas Can Work", "error in (no error)"=w1746, "Queue in"=w1745) -> ("error out"=w1744:errorcluster)  [unwired: 7 in, 1 out]
      }
      frame "DisplayValuesFromAlicat_FVIR" {
        # "Display the values from the gas meter FVIR loop"
        n537 = Variant To Data(error in=w1773, type=T16 {"Data Cluster"={"Absolute Pressure"=0.0, "Gauge/Diff. Pressure"=0.0, "Barometric Pressure"=0.0, "Temperature"=0.0, "Volumetric Flow"=0.0, "Mass Flow"=0.0, "Setpoint"=0.0, "Valve Drive"=0.0, "Totalizer"=0.0, "[hr]"=0.0, "[min]"=0.0, "[sec]"=0.0, "Totalizer Average Flow"=0.0, "Totalizer Peak Flow"=0.0, "Gas selected"=""}, "Units of Measure Input"={"Abs. Pressure"="", "Gauge/Diff. Press."="", "Barometric Press."="", "Temperature"="", "Volume"="", "Mass"="", "Setpoint"="", "Valve Drive"="", "Totalizer"="", "Tot. Timer"="", "Tot. Avg. Flow"="", "Tot. Peak Flow"=""}, "Header Array"=[]} ("Gas Data"), Variant=w1772) -> (data=w1764:T16, error out=w1769:errorcluster)
        n538 = Bundle By Name(cluster=w1766, "Gas Data.Gas Data - FVIR"=w1764) -> (w1765:T7)
        n539 = call-poly "Enqueue Message.vi"("error in (no error)"=w1769, "Message"="DisplayAllData_FVIR", "Message Queue"=w1770) -> ("error out"=w1768:errorcluster)  [unwired: 7 in, 1 out]
      }
      frame "DisplayValuesFromUltramat_FVIR" {
        # "Display the values from the Ultramat FVIR loop"
        n540 = Variant To Data(error in=w1785, type=string[][] [], Variant=w1784) -> (data=w1776:string[][], error out=w1782:errorcluster)
        n541 = Bundle By Name(cluster=w1779, "Ultramat 23.Ultramat 23 - FVIR"=w1776) -> (w1778:T7)
        n542 = call-poly "Enqueue Message.vi"("error in (no error)"=w1782, "Message"="DisplayAllData_FVIR", "Message Queue"=w1780) -> ("error out"=w1781:errorcluster)  [unwired: 7 in, 1 out]
      }
      frame "DisplayValuesFromVestaFVIR" {
        # "Display the values from the Ultramat FVIR loop"
        n543 = Variant To Data(error in=w1797, type=T20 {"Temp_W_Raw_U"=0, "Temp_W_Raw_L"=0, "Temperature Water (F)"=0.0, "Temperature Water Compensated (F)"=0.0, "Temperature Ambient (F)"=0.0, "Setpoint Location (F)"=0.0, "Heat Request"="", "Fault Ram"="", "PWM DCDC Value"=0, "Pilot Voltage (mV)"=0.0, "Setpoint Actual (F)"=0.0, "Differential Actual (F)"=0.0, "Setpoint User (F)"=0.0, "Differential User (F)"=0.0, "Termperature FIltered -TCO (F)"=0.0, "Temp_C_Raw_1 - Sensor Voltage"="", "Temp_C_Raw_2 - Sensor Voltage"="", "Chamber Sensor Temperature (F)"=0.0, "LDO Base Temperature (F)"=0.0, "LDO Timer (sec)"=0, "Disabled (0)"=FALSE, "Warming (1)"=FALSE, "Heating (2)"=FALSE, "Cooling Data Write (3)"=FALSE, "Cooling (4)"=FALSE, "Data Read (5)"=FALSE, "N/A"=FALSE, "Temperature Trip (7)"=FALSE, "Burner"=FALSE} ("Vesta Data.Vesta LDO"), Variant=w1796) -> (data=w1789:T20, error out=w1794:errorcluster)
        n544 = Bundle By Name(cluster=w1791, "Vesta Data.Vesta FVIR"=w1789) -> (w1790:T7)
        n545 = call-poly "Enqueue Message.vi"("error in (no error)"=w1794, "Message"="DisplayAllData_FVIR", "Message Queue"=w1792) -> ("error out"=w1793:errorcluster)  [unwired: 7 in, 1 out]
      }
      frame "DisplayValuesFromAgilent" {
        w1799 = T21 {"Temperature -1 (F)"=0.0, "Thermistor Reading -1 (kOhms)"=0.0, "Thermistor Reading -2 (kOhms)"=0.0, "Temperature -2 (F)"=0.0, "Thermistor Reading -3 (kOhms)"=0.0, "Temperature -3 (F)"=0.0, "Thermistor Reading -4 (kOhms)"=0.0, "Temperature -4 (F)"=0.0, "Thermistor Reading -5 (kOhms)"=0.0, "Temperature -5 (F)"=0.0, "Thermistor Reading -6 (kOhms)"=0.0, "Temperature -6 (F)"=0.0, "Thermistor Reading -7 (kOhms)"=0.0, "Temperature -7 (F)"=0.0, "Thermistor Reading -8 (kOhms)"=0.0, "Temperature -8 (F)"=0.0, "Thermistor Reading -9 (kOhms)"=0.0, "Temperature -9 (F)"=0.0, "Thermistor Reading -10 (kOhms)"=0.0, "Temperature -10 (F)"=0.0}  # Agilent Data
        # "Collect data from the Agilent loop."
        n546 = Variant To Data(error in=w1804, type=w1799, Variant=w1802) -> (data=w1805:T21, error out=w1803:errorcluster)
        n547 = Bundle By Name(cluster=w1801, "Agilent Data"=w1805) -> (w1800:T7)
      }
      frame "Start SRI Log" {
        # "Currently the hydrocarbon analyzer outputs a text file.\nThe software will read this text file. This is the start reading\nbutton"
        # "Note: So right now, I am writing to the HMI that we only read the log file. \nHowever the acqusition and logging from the original template does also happens, which needs to be \ncleaned up later."
        # "Start - Enable/Disable buttons appropriately for an acquisition that has started, and update status display."
        n548 = disable-structure shown="Disabled" {
          disable-tunnel: w1814 -> [w1826 _]
          frame Disabled {
            # "Enable: Stop\nDisable: Start, Exit, Settings"
            n549 = Unbundle By Name(w1826) -> ("Stop Ref"=w1821:refnum<vi>, "Start Ref"=w1820:refnum<vi>, "Exit Ref"=w1819:refnum<vi>)
            n550 = Build Array(w1820, w1819) -> (w1824:refnum<vi>[])
            n551 = Build Array(w1821) -> (w1823:refnum<vi>[])
            n552 = call "Set Enable State on Multiple Controls.vi"("Enable?"=FALSE, "Controls"=w1824) -> ()  [unwired: 10 in]
            n553 = call "Set Enable State on Multiple Controls.vi"("Enable?"=TRUE, "Controls"=w1823) -> ()  [unwired: 10 in]
          }
          frame Enabled {
          }
        }
        n554 = call-poly "Enqueue Message.vi"("error in (no error)"=w1817, "Message Data"="Starting to read log file..." ("Acquiring and Logging..."), "Message"="Update Status - FVIR", "Message Queue"=w1818) -> ("error out"=w1810:errorcluster)  [unwired: 6 in, 1 out]
        n555 = call-poly "Enqueue Message.vi"("error in (no error)"=w1810, "Message"="Start SRI Log", "Message Queue"=w1811) -> ("error out"=w1813:errorcluster)  [unwired: 7 in, 1 out]
      }
      frame "Stop SRI Log" {
        # "Currently the hydrocarbon analyzer outputs a text file.\nThe software will read this text file. This is the stop reading\nbutton"
        # "Stop - Enable/Disable buttons appropriately for an acquisition that has stopped, and update status display."
        n556 = disable-structure shown="Disabled" {
          disable-tunnel: w1830 -> [w1838 _]
          frame Disabled {
            n557 = Unbundle By Name(w1838) -> ("Stop Ref"=w1844:refnum<vi>, "Start Ref"=w1842:refnum<vi>, "Exit Ref"=w1841:refnum<vi>)
            n558 = Build Array(w1844) -> (w1840:refnum<vi>[])
            n559 = Build Array(w1842, w1841) -> (w1839:refnum<vi>[])
            n560 = call "Set Enable State on Multiple Controls.vi"("Enable?"=FALSE, "Controls"=w1840) -> ()  [unwired: 10 in]
            n561 = call "Set Enable State on Multiple Controls.vi"("Enable?"=TRUE, "Controls"=w1839) -> ()  [unwired: 10 in]
          }
          frame Enabled {
          }
        }
        n562 = call-poly "Enqueue Message.vi"("error in (no error)"=w1833, "Message Data"="Stopping to read log file..." ("Acquiring and Logging..."), "Message"="Update Status - FVIR", "Message Queue"=w1836) -> ("error out"=w1832:errorcluster)  [unwired: 6 in, 1 out]
        n563 = call-poly "Enqueue Message.vi"("error in (no error)"=w1832, "Message"="Stop SRI Log", "Message Queue"=w1831) -> ("error out"=w1827:errorcluster)  [unwired: 7 in, 1 out]
      }
      frame "CheckBeforeWriteDataFVIR" {
        # "Send the latest information to the \ndata save loop"
        n564 = Unbundle By Name(w1848) -> ("PLC Data"=w1847:T8)
        n565 = call-poly "Enqueue Message.vi"("error in (no error)"=w1849, "Message Data"=w1847, "Message"="CheckBeforeWriteDataFVIR", "Message Queue"=w1846) -> ("error out"=w1851:errorcluster)  [unwired: 6 in, 1 out]
      }
      frame "Start ANSI FVIR" {
        n566 = Unbundle By Name(w1859) -> ("PLC Data.PLC Data - FVIR.Timing.Absolute Time"=w1858:dbl)
        n567 = Bundle By Name(cluster=w1859, "ANSI Rates.ANSI Rate FVIR.ANSI Start Time"=w1858) -> (w1860:T7)
        n568 = call-poly "Enqueue Message.vi"("error in (no error)"=w1856, "Message"="ANSI Rate FVIR", "Message Queue"=w1854) -> ("error out"=w1855:errorcluster)  [unwired: 7 in, 1 out]
      }
      frame "ANSI Rate FVIR" {
        n569 = Unbundle By Name(w1871) -> ("ANSI Rates.ANSI Rate FVIR"=w1872:T19, "Ultramat 23.Ultramat 23 - FVIR"=w1873:string[][], "Gas Data.Gas Data - FVIR.Data Cluster"=w1874:T17, "Inficon Data - ALL"=w1877:T15, "PLC Data.PLC Data - FVIR.Timing.Absolute Time"=w1864:dbl)
        n570 = call "HEWH ANSI Get Rates.vi"("ANSI Rate in"=w1872, "Test Type - Rate"="Test Type - Rate FVIR", "CO CO2 Data Array"=w1873, "Gas Measurment Data"=w1874, "Inficon Data - ALL"=w1877, "error in (no error)"=w1878, "Software Elapsed Time"=w1864) -> ("ANSI Display 1"=→"ANSI Display FVIR":string, "ANSI Rate out"=w1869:T19, "Rate Outputs"=→"FVIR Rate Info":string[][], "Test Complete"=w1863:bool, "error out"=w1867:errorcluster)  [unwired: 4 in]
        n571 = Bundle By Name(cluster=w1871, "ANSI Rates.ANSI Rate FVIR"=w1869) -> (w1870:T7)
        n572 = case shown="True" w1863 {
          tunnel: w1867 -> [w1884 w1890]
          tunnel: [w1883 w1890] -> w1866
          tunnel: w1865 -> [w1882 _]
          frame False {
            n573 = property on="Start ANSI FVIR" class="Bool (strict)"() -> ("Value"=w1881:bool)  [unwired: 2 in, 2 out]
            n574 = case shown="False" w1881 {
              tunnel: w1884 -> [w1885 w1888]
              tunnel: [w1885 w1887] -> w1883
              tunnel: w1882 -> [_ w1886]
              frame False {
              }
              frame True {
                n575 = call-poly "Enqueue Message.vi"("error in (no error)"=w1888, "Message"="ANSI Rate FVIR", "Message Queue"=w1886) -> ("error out"=w1887:errorcluster)  [unwired: 7 in, 1 out]
              }
            }
          }
          frame True {
            n576 = property on="Start ANSI FVIR" class="Bool (strict)"("Value"=FALSE ("Start ANSI FVIR")) -> ()  [unwired: 2 in, 2 out]
          }
        }
      }
    }
    n577 = case shown="True" "Debug" {
      tunnel: w621 -> [w643 w647]
      tunnel: w620 -> [_ w646]
      tunnel: [w643 w644] -> w619
      frame False {
      }
      frame True {
        n578 = Build Array (concatenate)(w647, w646) -> (w645:string[])
        n579 = Reverse 1D Array(array=w645) -> (reversed array=w644:string[])
        "Message Loop" <- w644
      }
    }
    n580 = call "Error Handler - Message Handling Loop.vi"("error in (no error)"=w633, "Message Queue"=w632) -> ("dup error in"=w634:errorcluster)  [unwired: 8 in, 1 out]
  }
  n581 = Unregister For Events(event registration refnum=w71, error in=w74) -> (error out=w72:errorcluster)
  n582 = Release Queue(queue=w44, error in (no error)=w75) -> (error out=w60:errorcluster)  [unwired: 1 in, 2 out]
  n583 = Merge Errors(w72, w60, w62, w29, w61, w59, w52, w43, w51, w50, w37, w27, w24, w19, w10) -> (w69:errorcluster)
  n584 = call "Destroy User Event - Stop.vi"("error in (no error)"=w69, "User Event - Stop"=w65) -> ("error out"=w68:errorcluster)  [unwired: 9 in]
  n585 = disable-structure shown="Default" {
    disable-tunnel: w68 -> [_ _]
    frame condition #0 (active) {
    }
    frame condition #1 {
      # "Call Quit LabVIEW if running as a built application."
      n586 = Quit LabVIEW() -> ()  [unwired: 1 in]
    }
  }
